vi "Waveform 64-128 channels LP pt by pt.vi"(4 "Enum":T1(ring), 6 "order":i32=2, 8 "fl":dbl, 10 "fs":dbl, 11 "Array in":waveform(dbl)[](array[waveform])) -> (3 "Array out":waveform(dbl)[](array[waveform]))   [LabVIEW 2016, in "LockinDAQ.lvclass"]
uses:
  LockinDAQ.lvclass
  <vilib>/Analysis/3filter.llb/Filter Passband Type.ctl
  <vilib>/Analysis/baseanly.llb/Mean (DBL).vi
  <vilib>/addons/Digital Filter Design/Process.llb/DFD Filtering (Wfm NChan).vi
  <vilib>/addons/System Identification/Data Preprocess.llb/SI Lowpass Filter (SISO Waveform).vi
  <vilib>/Analysis/3filter.llb/Butterworth Filter (DBL).vi
  <vilib>/ptbypt/NI_PtbyPt.lvlib
  <vilib>/Analysis/NI_AALBase.lvlib
  <vilib>/addons/System Identification/NI_SysID.lvlib
  <vilib>/addons/Digital Filter Design/NI_DigFilterLicensed.lvlib
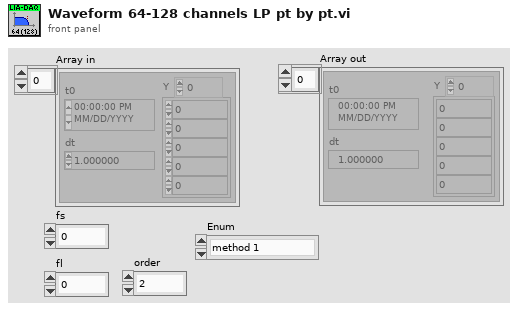
[diagram p1: front panel]
types:
  T1 = enum16{"method 1", "method 2", "method 3", "method 4", "method 5"}
  T2 = typedef "NI_AALBase.lvlib/Filter Passband Type.ctl" = enum32{"Lowpass", "Highpass", "Bandpass", "Bandstop"}
  T3 = enum16{"Lowpass", "Highpass", "Bandpass", "Bandstop"}
  T4 = typedef "NI_DigFilterLicensed.lvlib/DFD Filter Obj.ctl" = cluster{"mSRate_Fs":dbl, "mSRate_Version":string, "mSRate_Comments":string, "mSRate_OrgCoef":T5, "mSRate_CurCoef":T5, "mSRate_Quantized?":bool, "mSRate_QCoef":T5, "mSRate_QSettings":T7[], "mSRate_Order":i32, "mSRate_Scaling":cluster{"mSRate_ScaleByPowerOf2?":bool, "mSRate_ScaleType":T9}}
  T5 = typedef "NI_DigFilterLicensed.lvlib/DFD Filter Coef.ctl" = cluster{"type":T6, "gain":dbl, "coef a (k)":dbl[], "coef b (v)":dbl[]}
  T6 = typedef "NI_DigFilterLicensed.lvlib/DFD Filter Structure Type Selector.ctl" = enum16{"Undefined", "FIR Direct Form", "FIR Direct Form Transposed", "FIR Symmetric", "FIR Antisymmetric", "IIR Direct Form I", "IIR Direct Form I Transposed", "IIR Direct Form II", "IIR Direct Form II Transposed", "IIR Cascaded Second Order Sections Form I", "IIR Cascaded Second Order Sections Form I Transposed", "IIR Cascaded Second Order Sections Form II", "IIR Cascaded Second Order Sections Form II Transposed", "Lattice Allpass (basic sections)", "Lattice Allpass (one multiplier sections)", "Lattice Allpass (normalized sections)", "Lattice AR (basic sections)", "Lattice AR (one multiplier sections)", "Lattice AR (normalized sections)", "Lattice MA (minimum phase)", "Lattice MA (maximum phase)", "Lattice ARMA (basic sections)", "Lattice ARMA (one multiplier sections)", "Lattice ARMA (normalized sections)"}
  T7 = typedef "NI_DigFilterLicensed.lvlib/dfd_Internal Quantization Settings.ctl" = cluster{"source":T8, "wl":i16, "iwl":i16, "overflow mode":enum16{"Saturation", "Wrap"}, "rounding mode":enum16{"Nearest", "Truncation"}, "signed?":bool}
  T8 = typedef "NI_DigFilterLicensed.lvlib/dfd_Internal Quantization Srcs.ctl" = u16
  T9 = typedef "NI_DigFilterLicensed.lvlib/DFD Coef Norm Type.ctl" = enum16{"No Norm", "Time Domain 1-Norm", "Time Domain 2-Norm", "Time Domain Inf-Norm"}
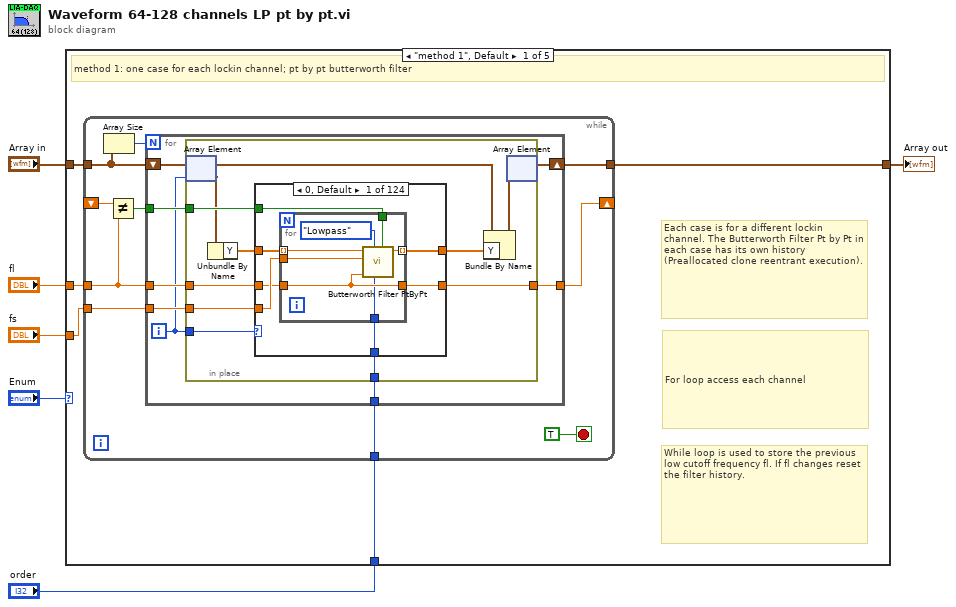
[diagram p0: block diagram]
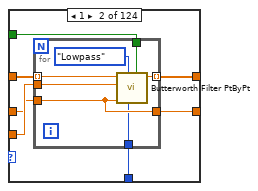
[diagram p2: hidden frame]
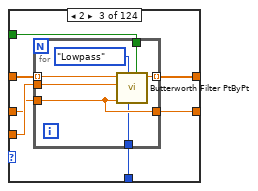
[diagram p3: hidden frame]
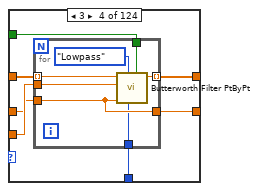
[diagram p4: hidden frame]
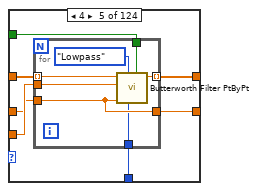
[diagram p5: hidden frame]
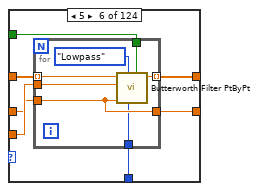
[diagram p6: hidden frame]
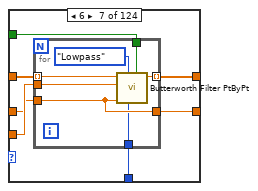
[diagram p7: hidden frame]
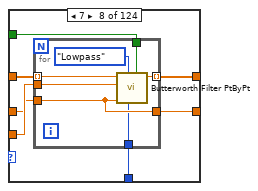
[diagram p8: hidden frame]
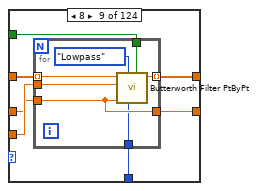
[diagram p9: hidden frame]
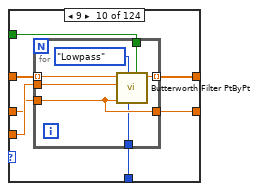
[diagram p10: hidden frame]
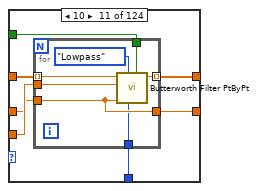
[diagram p11: hidden frame]
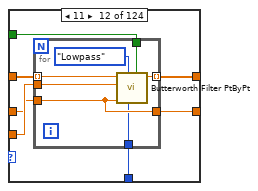
[diagram p12: hidden frame]
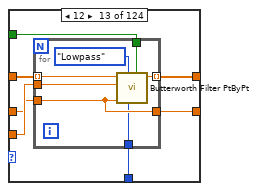
[diagram p13: hidden frame]
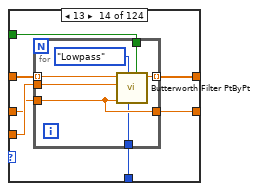
[diagram p14: hidden frame]
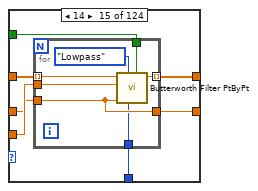
[diagram p15: hidden frame]
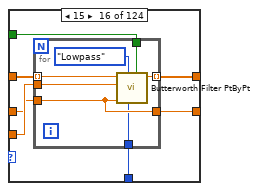
[diagram p16: hidden frame]
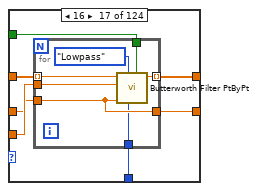
[diagram p17: hidden frame]
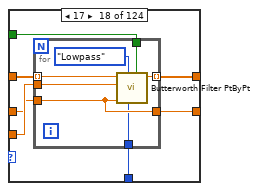
[diagram p18: hidden frame]
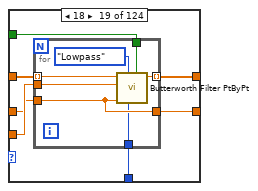
[diagram p19: hidden frame]
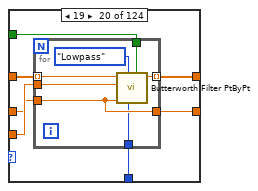
[diagram p20: hidden frame]
diagram:
  n1 = case shown="\"method 1\", Default" "Enum" {
    tunnel: "Array in" -> [w11 w1780 w3493 w3511 w3532]
    tunnel: [w10 w1779 w3492 w3510 w3531] -> w4
    tunnel: "fs" -> [w9 w1778 w3491 w3509 w3530]
    tunnel: "fl" -> [w8 w1777 w3490 w3508 w3529]
    tunnel: "order" -> [w7 w1776 w3489 w3507 w3528]
    frame "method 1", Default {
      # "For loop access each channel"
      # "While loop is used to store the previous low cutoff frequency fl. If fl changes reset the filter history."
      # "Each case is for a different lockin channel. The Butterworth Filter Pt by Pt in each case has its own history (Preallocated clone reentrant execution)."
      # "method 1: one case for each lockin channel; pt by pt butterworth filter"
      n2 = while {
        tunnel: w11 -> [w12]
        tunnel: [w21] -> w10
        tunnel: w9 -> [w18]
        tunnel: w8 -> [w15]
        shift-right: [w19] -> _
        shift-left: _ -> [w17]
        tunnel: w7 -> [w16]
        stop <- TRUE stop-if-true
        n3 = Array Size(array=w12) -> (size(s)=w13:i32)
        n4 = Not Equal?(x=w17, y=w15) -> (x != y?=w14:bool)
        n5 = for {
          N: w13 -> [_]
          tunnel: w18 -> [w29]
          tunnel: w15 -> [w28]
          tunnel: [w27] -> w19
          tunnel: w14 -> [w26]
          tunnel: w16 -> [w25]
          shift-right: [w22] -> w21
          shift-left: w12 -> [w24]
          i -> [w23]
          n6 = in-place {
            in-place-border: w29 -> [w39]
            in-place-border: w28 -> [w38]
            in-place-border: [w37] -> w27
            in-place-border: w26 -> [w36]
            in-place-border: w25 -> [w35]
            in-place-border: w23 -> [w32]
            n7 = in-place-array #1(w24, w23) -> (w31:waveform(dbl))
            n8 = Unbundle By Name(w31) -> ("Y"=w33:dbl[])
            n9 = case shown="0, Default" w32 {
              tunnel: w39 -> [w46 w60 w74 w88 w102 w116 w130 w144 w158 w172 w186 w200 w214 w228 w242 w256 w270 w284 w298 w312 w326 w340 w354 w368 w382 w396 w410 w424 w438 w452 w466 w480 w494 w508 w522 w536 w550 w564 w578 w592 w606 w620 w634 w648 w662 w676 w690 w704 w718 w732 w746 w760 w774 w788 w802 w816 w830 w844 w858 w872 w886 w900 w914 w928 w942 w956 w970 w984 w998 w1012 w1026 w1040 w1054 w1068 w1082 w1096 w1110 w1124 w1138 w1152 w1166 w1180 w1194 w1208 w1222 w1236 w1250 w1264 w1278 w1292 w1306 w1320 w1334 w1348 w1362 w1376 w1390 w1404 w1418 w1432 w1446 w1460 w1474 w1488 w1502 w1516 w1530 w1544 w1558 w1572 w1586 w1600 w1614 w1628 w1642 w1656 w1670 w1684 w1698 w1712 w1726 w1740 w1754 w1768]
              tunnel: w38 -> [w45 w59 w73 w87 w101 w115 w129 w143 w157 w171 w185 w199 w213 w227 w241 w255 w269 w283 w297 w311 w325 w339 w353 w367 w381 w395 w409 w423 w437 w451 w465 w479 w493 w507 w521 w535 w549 w563 w577 w591 w605 w619 w633 w647 w661 w675 w689 w703 w717 w731 w745 w759 w773 w787 w801 w815 w829 w843 w857 w871 w885 w899 w913 w927 w941 w955 w969 w983 w997 w1011 w1025 w1039 w1053 w1067 w1081 w1095 w1109 w1123 w1137 w1151 w1165 w1179 w1193 w1207 w1221 w1235 w1249 w1263 w1277 w1291 w1305 w1319 w1333 w1347 w1361 w1375 w1389 w1403 w1417 w1431 w1445 w1459 w1473 w1487 w1501 w1515 w1529 w1543 w1557 w1571 w1585 w1599 w1613 w1627 w1641 w1655 w1669 w1683 w1697 w1711 w1725 w1739 w1753 w1767]
              tunnel: [w44 w58 w72 w86 w100 w114 w128 w142 w156 w170 w184 w198 w212 w226 w240 w254 w268 w282 w296 w310 w324 w338 w352 w366 w380 w394 w408 w422 w436 w450 w464 w478 w492 w506 w520 w534 w548 w562 w576 w590 w604 w618 w632 w646 w660 w674 w688 w702 w716 w730 w744 w758 w772 w786 w800 w814 w828 w842 w856 w870 w884 w898 w912 w926 w940 w954 w968 w982 w996 w1010 w1024 w1038 w1052 w1066 w1080 w1094 w1108 w1122 w1136 w1150 w1164 w1178 w1192 w1206 w1220 w1234 w1248 w1262 w1276 w1290 w1304 w1318 w1332 w1346 w1360 w1374 w1388 w1402 w1416 w1430 w1444 w1458 w1472 w1486 w1500 w1514 w1528 w1542 w1556 w1570 w1584 w1598 w1612 w1626 w1640 w1654 w1668 w1682 w1696 w1710 w1724 w1738 w1752 w1766] -> w37
              tunnel: w36 -> [w43 w57 w71 w85 w99 w113 w127 w141 w155 w169 w183 w197 w211 w225 w239 w253 w267 w281 w295 w309 w323 w337 w351 w365 w379 w393 w407 w421 w435 w449 w463 w477 w491 w505 w519 w533 w547 w561 w575 w589 w603 w617 w631 w645 w659 w673 w687 w701 w715 w729 w743 w757 w771 w785 w799 w813 w827 w841 w855 w869 w883 w897 w911 w925 w939 w953 w967 w981 w995 w1009 w1023 w1037 w1051 w1065 w1079 w1093 w1107 w1121 w1135 w1149 w1163 w1177 w1191 w1205 w1219 w1233 w1247 w1261 w1275 w1289 w1303 w1317 w1331 w1345 w1359 w1373 w1387 w1401 w1415 w1429 w1443 w1457 w1471 w1485 w1499 w1513 w1527 w1541 w1555 w1569 w1583 w1597 w1611 w1625 w1639 w1653 w1667 w1681 w1695 w1709 w1723 w1737 w1751 w1765]
              tunnel: w35 -> [w42 w56 w70 w84 w98 w112 w126 w140 w154 w168 w182 w196 w210 w224 w238 w252 w266 w280 w294 w308 w322 w336 w350 w364 w378 w392 w406 w420 w434 w448 w462 w476 w490 w504 w518 w532 w546 w560 w574 w588 w602 w616 w630 w644 w658 w672 w686 w700 w714 w728 w742 w756 w770 w784 w798 w812 w826 w840 w854 w868 w882 w896 w910 w924 w938 w952 w966 w980 w994 w1008 w1022 w1036 w1050 w1064 w1078 w1092 w1106 w1120 w1134 w1148 w1162 w1176 w1190 w1204 w1218 w1232 w1246 w1260 w1274 w1288 w1302 w1316 w1330 w1344 w1358 w1372 w1386 w1400 w1414 w1428 w1442 w1456 w1470 w1484 w1498 w1512 w1526 w1540 w1554 w1568 w1582 w1596 w1610 w1624 w1638 w1652 w1666 w1680 w1694 w1708 w1722 w1736 w1750 w1764]
              tunnel: [w41 w55 w69 w83 w97 w111 w125 w139 w153 w167 w181 w195 w209 w223 w237 w251 w265 w279 w293 w307 w321 w335 w349 w363 w377 w391 w405 w419 w433 w447 w461 w475 w489 w503 w517 w531 w545 w559 w573 w587 w601 w615 w629 w643 w657 w671 w685 w699 w713 w727 w741 w755 w769 w783 w797 w811 w825 w839 w853 w867 w881 w895 w909 w923 w937 w951 w965 w979 w993 w1007 w1021 w1035 w1049 w1063 w1077 w1091 w1105 w1119 w1133 w1147 w1161 w1175 w1189 w1203 w1217 w1231 w1245 w1259 w1273 w1287 w1301 w1315 w1329 w1343 w1357 w1371 w1385 w1399 w1413 w1427 w1441 w1455 w1469 w1483 w1497 w1511 w1525 w1539 w1553 w1567 w1581 w1595 w1609 w1623 w1637 w1651 w1665 w1679 w1693 w1707 w1721 w1735 w1749 w1763] -> w34
              tunnel: w33 -> [w40 w54 w68 w82 w96 w110 w124 w138 w152 w166 w180 w194 w208 w222 w236 w250 w264 w278 w292 w306 w320 w334 w348 w362 w376 w390 w404 w418 w432 w446 w460 w474 w488 w502 w516 w530 w544 w558 w572 w586 w600 w614 w628 w642 w656 w670 w684 w698 w712 w726 w740 w754 w768 w782 w796 w810 w824 w838 w852 w866 w880 w894 w908 w922 w936 w950 w964 w978 w992 w1006 w1020 w1034 w1048 w1062 w1076 w1090 w1104 w1118 w1132 w1146 w1160 w1174 w1188 w1202 w1216 w1230 w1244 w1258 w1272 w1286 w1300 w1314 w1328 w1342 w1356 w1370 w1384 w1398 w1412 w1426 w1440 w1454 w1468 w1482 w1496 w1510 w1524 w1538 w1552 w1566 w1580 w1594 w1608 w1622 w1636 w1650 w1664 w1678 w1692 w1706 w1720 w1734 w1748 w1762]
              frame 0, Default {
                n10 = for {
                  tunnel: w40 -> [w53] mode=indexing
                  tunnel: w45 -> [w50]
                  tunnel: w46 -> [w52]
                  tunnel: [w51] -> w41 mode=indexing
                  tunnel: [w50] -> w44
                  tunnel: w43 -> [w48]
                  tunnel: w42 -> [w47]
                  n11 = call <vilib>:"Butterworth Filter PtByPt.vi"("initialize"=w48, "order"=w47, "filter type"=Filter_Passband_Type."Lowpass", "low cutoff freq: fl"=w50, "sampling freq: fs"=w52, "x"=w53) -> ("Filtered x"=w51:dbl)  [unwired: 3 in, 1 out]
                }
              }
              frame 1 {
                n12 = for {
                  tunnel: w54 -> [w67] mode=indexing
                  tunnel: w59 -> [w64]
                  tunnel: w60 -> [w66]
                  tunnel: [w65] -> w55 mode=indexing
                  tunnel: [w64] -> w58
                  tunnel: w57 -> [w62]
                  tunnel: w56 -> [w61]
                  n13 = call <vilib>:"Butterworth Filter PtByPt.vi"("initialize"=w62, "order"=w61, "filter type"=Filter_Passband_Type."Lowpass", "low cutoff freq: fl"=w64, "sampling freq: fs"=w66, "x"=w67) -> ("Filtered x"=w65:dbl)  [unwired: 3 in, 1 out]
                }
              }
              frame 2 {
                n14 = for {
                  tunnel: w68 -> [w81] mode=indexing
                  tunnel: w73 -> [w78]
                  tunnel: w74 -> [w80]
                  tunnel: [w79] -> w69 mode=indexing
                  tunnel: [w78] -> w72
                  tunnel: w71 -> [w76]
                  tunnel: w70 -> [w75]
                  n15 = call <vilib>:"Butterworth Filter PtByPt.vi"("initialize"=w76, "order"=w75, "filter type"=Filter_Passband_Type."Lowpass", "low cutoff freq: fl"=w78, "sampling freq: fs"=w80, "x"=w81) -> ("Filtered x"=w79:dbl)  [unwired: 3 in, 1 out]
                }
              }
              frame 3 {
                n16 = for {
                  tunnel: w82 -> [w95] mode=indexing
                  tunnel: w87 -> [w92]
                  tunnel: w88 -> [w94]
                  tunnel: [w93] -> w83 mode=indexing
                  tunnel: [w92] -> w86
                  tunnel: w85 -> [w90]
                  tunnel: w84 -> [w89]
                  n17 = call <vilib>:"Butterworth Filter PtByPt.vi"("initialize"=w90, "order"=w89, "filter type"=Filter_Passband_Type."Lowpass", "low cutoff freq: fl"=w92, "sampling freq: fs"=w94, "x"=w95) -> ("Filtered x"=w93:dbl)  [unwired: 3 in, 1 out]
                }
              }
              frame 4 {
                n18 = for {
                  tunnel: w96 -> [w109] mode=indexing
                  tunnel: w101 -> [w106]
                  tunnel: w102 -> [w108]
                  tunnel: [w107] -> w97 mode=indexing
                  tunnel: [w106] -> w100
                  tunnel: w99 -> [w104]
                  tunnel: w98 -> [w103]
                  n19 = call <vilib>:"Butterworth Filter PtByPt.vi"("initialize"=w104, "order"=w103, "filter type"=Filter_Passband_Type."Lowpass", "low cutoff freq: fl"=w106, "sampling freq: fs"=w108, "x"=w109) -> ("Filtered x"=w107:dbl)  [unwired: 3 in, 1 out]
                }
              }
              frame 5 {
                n20 = for {
                  tunnel: w110 -> [w123] mode=indexing
                  tunnel: w115 -> [w120]
                  tunnel: w116 -> [w122]
                  tunnel: [w121] -> w111 mode=indexing
                  tunnel: [w120] -> w114
                  tunnel: w113 -> [w118]
                  tunnel: w112 -> [w117]
                  n21 = call <vilib>:"Butterworth Filter PtByPt.vi"("initialize"=w118, "order"=w117, "filter type"=Filter_Passband_Type."Lowpass", "low cutoff freq: fl"=w120, "sampling freq: fs"=w122, "x"=w123) -> ("Filtered x"=w121:dbl)  [unwired: 3 in, 1 out]
                }
              }
              frame 6 {
                n22 = for {
                  tunnel: w124 -> [w137] mode=indexing
                  tunnel: w129 -> [w134]
                  tunnel: w130 -> [w136]
                  tunnel: [w135] -> w125 mode=indexing
                  tunnel: [w134] -> w128
                  tunnel: w127 -> [w132]
                  tunnel: w126 -> [w131]
                  n23 = call <vilib>:"Butterworth Filter PtByPt.vi"("initialize"=w132, "order"=w131, "filter type"=Filter_Passband_Type."Lowpass", "low cutoff freq: fl"=w134, "sampling freq: fs"=w136, "x"=w137) -> ("Filtered x"=w135:dbl)  [unwired: 3 in, 1 out]
                }
              }
              frame 7 {
                n24 = for {
                  tunnel: w138 -> [w151] mode=indexing
                  tunnel: w143 -> [w148]
                  tunnel: w144 -> [w150]
                  tunnel: [w149] -> w139 mode=indexing
                  tunnel: [w148] -> w142
                  tunnel: w141 -> [w146]
                  tunnel: w140 -> [w145]
                  n25 = call <vilib>:"Butterworth Filter PtByPt.vi"("initialize"=w146, "order"=w145, "filter type"=Filter_Passband_Type."Lowpass", "low cutoff freq: fl"=w148, "sampling freq: fs"=w150, "x"=w151) -> ("Filtered x"=w149:dbl)  [unwired: 3 in, 1 out]
                }
              }
              frame 8 {
                n26 = for {
                  tunnel: w152 -> [w165] mode=indexing
                  tunnel: w157 -> [w162]
                  tunnel: w158 -> [w164]
                  tunnel: [w163] -> w153 mode=indexing
                  tunnel: [w162] -> w156
                  tunnel: w155 -> [w160]
                  tunnel: w154 -> [w159]
                  n27 = call <vilib>:"Butterworth Filter PtByPt.vi"("initialize"=w160, "order"=w159, "filter type"=Filter_Passband_Type."Lowpass", "low cutoff freq: fl"=w162, "sampling freq: fs"=w164, "x"=w165) -> ("Filtered x"=w163:dbl)  [unwired: 3 in, 1 out]
                }
              }
              frame 9 {
                n28 = for {
                  tunnel: w166 -> [w179] mode=indexing
                  tunnel: w171 -> [w176]
                  tunnel: w172 -> [w178]
                  tunnel: [w177] -> w167 mode=indexing
                  tunnel: [w176] -> w170
                  tunnel: w169 -> [w174]
                  tunnel: w168 -> [w173]
                  n29 = call <vilib>:"Butterworth Filter PtByPt.vi"("initialize"=w174, "order"=w173, "filter type"=Filter_Passband_Type."Lowpass", "low cutoff freq: fl"=w176, "sampling freq: fs"=w178, "x"=w179) -> ("Filtered x"=w177:dbl)  [unwired: 3 in, 1 out]
                }
              }
              frame 10 {
                n30 = for {
                  tunnel: w180 -> [w193] mode=indexing
                  tunnel: w185 -> [w190]
                  tunnel: w186 -> [w192]
                  tunnel: [w191] -> w181 mode=indexing
                  tunnel: [w190] -> w184
                  tunnel: w183 -> [w188]
                  tunnel: w182 -> [w187]
                  n31 = call <vilib>:"Butterworth Filter PtByPt.vi"("initialize"=w188, "order"=w187, "filter type"=Filter_Passband_Type."Lowpass", "low cutoff freq: fl"=w190, "sampling freq: fs"=w192, "x"=w193) -> ("Filtered x"=w191:dbl)  [unwired: 3 in, 1 out]
                }
              }
              frame 11 {
                n32 = for {
                  tunnel: w194 -> [w207] mode=indexing
                  tunnel: w199 -> [w204]
                  tunnel: w200 -> [w206]
                  tunnel: [w205] -> w195 mode=indexing
                  tunnel: [w204] -> w198
                  tunnel: w197 -> [w202]
                  tunnel: w196 -> [w201]
                  n33 = call <vilib>:"Butterworth Filter PtByPt.vi"("initialize"=w202, "order"=w201, "filter type"=Filter_Passband_Type."Lowpass", "low cutoff freq: fl"=w204, "sampling freq: fs"=w206, "x"=w207) -> ("Filtered x"=w205:dbl)  [unwired: 3 in, 1 out]
                }
              }
              frame 12 {
                n34 = for {
                  tunnel: w208 -> [w221] mode=indexing
                  tunnel: w213 -> [w218]
                  tunnel: w214 -> [w220]
                  tunnel: [w219] -> w209 mode=indexing
                  tunnel: [w218] -> w212
                  tunnel: w211 -> [w216]
                  tunnel: w210 -> [w215]
                  n35 = call <vilib>:"Butterworth Filter PtByPt.vi"("initialize"=w216, "order"=w215, "filter type"=Filter_Passband_Type."Lowpass", "low cutoff freq: fl"=w218, "sampling freq: fs"=w220, "x"=w221) -> ("Filtered x"=w219:dbl)  [unwired: 3 in, 1 out]
                }
              }
              frame 13 {
                n36 = for {
                  tunnel: w222 -> [w235] mode=indexing
                  tunnel: w227 -> [w232]
                  tunnel: w228 -> [w234]
                  tunnel: [w233] -> w223 mode=indexing
                  tunnel: [w232] -> w226
                  tunnel: w225 -> [w230]
                  tunnel: w224 -> [w229]
                  n37 = call <vilib>:"Butterworth Filter PtByPt.vi"("initialize"=w230, "order"=w229, "filter type"=Filter_Passband_Type."Lowpass", "low cutoff freq: fl"=w232, "sampling freq: fs"=w234, "x"=w235) -> ("Filtered x"=w233:dbl)  [unwired: 3 in, 1 out]
                }
              }
              frame 14 {
                n38 = for {
                  tunnel: w236 -> [w249] mode=indexing
                  tunnel: w241 -> [w246]
                  tunnel: w242 -> [w248]
                  tunnel: [w247] -> w237 mode=indexing
                  tunnel: [w246] -> w240
                  tunnel: w239 -> [w244]
                  tunnel: w238 -> [w243]
                  n39 = call <vilib>:"Butterworth Filter PtByPt.vi"("initialize"=w244, "order"=w243, "filter type"=Filter_Passband_Type."Lowpass", "low cutoff freq: fl"=w246, "sampling freq: fs"=w248, "x"=w249) -> ("Filtered x"=w247:dbl)  [unwired: 3 in, 1 out]
                }
              }
              frame 15 {
                n40 = for {
                  tunnel: w250 -> [w263] mode=indexing
                  tunnel: w255 -> [w260]
                  tunnel: w256 -> [w262]
                  tunnel: [w261] -> w251 mode=indexing
                  tunnel: [w260] -> w254
                  tunnel: w253 -> [w258]
                  tunnel: w252 -> [w257]
                  n41 = call <vilib>:"Butterworth Filter PtByPt.vi"("initialize"=w258, "order"=w257, "filter type"=Filter_Passband_Type."Lowpass", "low cutoff freq: fl"=w260, "sampling freq: fs"=w262, "x"=w263) -> ("Filtered x"=w261:dbl)  [unwired: 3 in, 1 out]
                }
              }
              frame 16 {
                n42 = for {
                  tunnel: w264 -> [w277] mode=indexing
                  tunnel: w269 -> [w274]
                  tunnel: w270 -> [w276]
                  tunnel: [w275] -> w265 mode=indexing
                  tunnel: [w274] -> w268
                  tunnel: w267 -> [w272]
                  tunnel: w266 -> [w271]
                  n43 = call <vilib>:"Butterworth Filter PtByPt.vi"("initialize"=w272, "order"=w271, "filter type"=Filter_Passband_Type."Lowpass", "low cutoff freq: fl"=w274, "sampling freq: fs"=w276, "x"=w277) -> ("Filtered x"=w275:dbl)  [unwired: 3 in, 1 out]
                }
              }
              frame 17 {
                n44 = for {
                  tunnel: w278 -> [w291] mode=indexing
                  tunnel: w283 -> [w288]
                  tunnel: w284 -> [w290]
                  tunnel: [w289] -> w279 mode=indexing
                  tunnel: [w288] -> w282
                  tunnel: w281 -> [w286]
                  tunnel: w280 -> [w285]
                  n45 = call <vilib>:"Butterworth Filter PtByPt.vi"("initialize"=w286, "order"=w285, "filter type"=Filter_Passband_Type."Lowpass", "low cutoff freq: fl"=w288, "sampling freq: fs"=w290, "x"=w291) -> ("Filtered x"=w289:dbl)  [unwired: 3 in, 1 out]
                }
              }
              frame 18 {
                n46 = for {
                  tunnel: w292 -> [w305] mode=indexing
                  tunnel: w297 -> [w302]
                  tunnel: w298 -> [w304]
                  tunnel: [w303] -> w293 mode=indexing
                  tunnel: [w302] -> w296
                  tunnel: w295 -> [w300]
                  tunnel: w294 -> [w299]
                  n47 = call <vilib>:"Butterworth Filter PtByPt.vi"("initialize"=w300, "order"=w299, "filter type"=Filter_Passband_Type."Lowpass", "low cutoff freq: fl"=w302, "sampling freq: fs"=w304, "x"=w305) -> ("Filtered x"=w303:dbl)  [unwired: 3 in, 1 out]
                }
              }
              frame 19 {
                n48 = for {
                  tunnel: w306 -> [w319] mode=indexing
                  tunnel: w311 -> [w316]
                  tunnel: w312 -> [w318]
                  tunnel: [w317] -> w307 mode=indexing
                  tunnel: [w316] -> w310
                  tunnel: w309 -> [w314]
                  tunnel: w308 -> [w313]
                  n49 = call <vilib>:"Butterworth Filter PtByPt.vi"("initialize"=w314, "order"=w313, "filter type"=Filter_Passband_Type."Lowpass", "low cutoff freq: fl"=w316, "sampling freq: fs"=w318, "x"=w319) -> ("Filtered x"=w317:dbl)  [unwired: 3 in, 1 out]
                }
              }
              frame 20 {
                n50 = for {
                  tunnel: w320 -> [w333] mode=indexing
                  tunnel: w325 -> [w330]
                  tunnel: w326 -> [w332]
                  tunnel: [w331] -> w321 mode=indexing
                  tunnel: [w330] -> w324
                  tunnel: w323 -> [w328]
                  tunnel: w322 -> [w327]
                  n51 = call <vilib>:"Butterworth Filter PtByPt.vi"("initialize"=w328, "order"=w327, "filter type"=Filter_Passband_Type."Lowpass", "low cutoff freq: fl"=w330, "sampling freq: fs"=w332, "x"=w333) -> ("Filtered x"=w331:dbl)  [unwired: 3 in, 1 out]
                }
              }
              frame 21 {
                n52 = for {
                  tunnel: w334 -> [w347] mode=indexing
                  tunnel: w339 -> [w344]
                  tunnel: w340 -> [w346]
                  tunnel: [w345] -> w335 mode=indexing
                  tunnel: [w344] -> w338
                  tunnel: w337 -> [w342]
                  tunnel: w336 -> [w341]
                  n53 = call <vilib>:"Butterworth Filter PtByPt.vi"("initialize"=w342, "order"=w341, "filter type"=Filter_Passband_Type."Lowpass", "low cutoff freq: fl"=w344, "sampling freq: fs"=w346, "x"=w347) -> ("Filtered x"=w345:dbl)  [unwired: 3 in, 1 out]
                }
              }
              frame 22 {
                n54 = for {
                  tunnel: w348 -> [w361] mode=indexing
                  tunnel: w353 -> [w358]
                  tunnel: w354 -> [w360]
                  tunnel: [w359] -> w349 mode=indexing
                  tunnel: [w358] -> w352
                  tunnel: w351 -> [w356]
                  tunnel: w350 -> [w355]
                  n55 = call <vilib>:"Butterworth Filter PtByPt.vi"("initialize"=w356, "order"=w355, "filter type"=Filter_Passband_Type."Lowpass", "low cutoff freq: fl"=w358, "sampling freq: fs"=w360, "x"=w361) -> ("Filtered x"=w359:dbl)  [unwired: 3 in, 1 out]
                }
              }
              frame 23 {
                n56 = for {
                  tunnel: w362 -> [w375] mode=indexing
                  tunnel: w367 -> [w372]
                  tunnel: w368 -> [w374]
                  tunnel: [w373] -> w363 mode=indexing
                  tunnel: [w372] -> w366
                  tunnel: w365 -> [w370]
                  tunnel: w364 -> [w369]
                  n57 = call <vilib>:"Butterworth Filter PtByPt.vi"("initialize"=w370, "order"=w369, "filter type"=Filter_Passband_Type."Lowpass", "low cutoff freq: fl"=w372, "sampling freq: fs"=w374, "x"=w375) -> ("Filtered x"=w373:dbl)  [unwired: 3 in, 1 out]
                }
              }
              frame 24 {
                n58 = for {
                  tunnel: w376 -> [w389] mode=indexing
                  tunnel: w381 -> [w386]
                  tunnel: w382 -> [w388]
                  tunnel: [w387] -> w377 mode=indexing
                  tunnel: [w386] -> w380
                  tunnel: w379 -> [w384]
                  tunnel: w378 -> [w383]
                  n59 = call <vilib>:"Butterworth Filter PtByPt.vi"("initialize"=w384, "order"=w383, "filter type"=Filter_Passband_Type."Lowpass", "low cutoff freq: fl"=w386, "sampling freq: fs"=w388, "x"=w389) -> ("Filtered x"=w387:dbl)  [unwired: 3 in, 1 out]
                }
              }
              frame 25 {
                n60 = for {
                  tunnel: w390 -> [w403] mode=indexing
                  tunnel: w395 -> [w400]
                  tunnel: w396 -> [w402]
                  tunnel: [w401] -> w391 mode=indexing
                  tunnel: [w400] -> w394
                  tunnel: w393 -> [w398]
                  tunnel: w392 -> [w397]
                  n61 = call <vilib>:"Butterworth Filter PtByPt.vi"("initialize"=w398, "order"=w397, "filter type"=Filter_Passband_Type."Lowpass", "low cutoff freq: fl"=w400, "sampling freq: fs"=w402, "x"=w403) -> ("Filtered x"=w401:dbl)  [unwired: 3 in, 1 out]
                }
              }
              frame 26 {
                n62 = for {
                  tunnel: w404 -> [w417] mode=indexing
                  tunnel: w409 -> [w414]
                  tunnel: w410 -> [w416]
                  tunnel: [w415] -> w405 mode=indexing
                  tunnel: [w414] -> w408
                  tunnel: w407 -> [w412]
                  tunnel: w406 -> [w411]
                  n63 = call <vilib>:"Butterworth Filter PtByPt.vi"("initialize"=w412, "order"=w411, "filter type"=Filter_Passband_Type."Lowpass", "low cutoff freq: fl"=w414, "sampling freq: fs"=w416, "x"=w417) -> ("Filtered x"=w415:dbl)  [unwired: 3 in, 1 out]
                }
              }
              frame 27 {
                n64 = for {
                  tunnel: w418 -> [w431] mode=indexing
                  tunnel: w423 -> [w428]
                  tunnel: w424 -> [w430]
                  tunnel: [w429] -> w419 mode=indexing
                  tunnel: [w428] -> w422
                  tunnel: w421 -> [w426]
                  tunnel: w420 -> [w425]
                  n65 = call <vilib>:"Butterworth Filter PtByPt.vi"("initialize"=w426, "order"=w425, "filter type"=Filter_Passband_Type."Lowpass", "low cutoff freq: fl"=w428, "sampling freq: fs"=w430, "x"=w431) -> ("Filtered x"=w429:dbl)  [unwired: 3 in, 1 out]
                }
              }
              frame 28 {
                n66 = for {
                  tunnel: w432 -> [w445] mode=indexing
                  tunnel: w437 -> [w442]
                  tunnel: w438 -> [w444]
                  tunnel: [w443] -> w433 mode=indexing
                  tunnel: [w442] -> w436
                  tunnel: w435 -> [w440]
                  tunnel: w434 -> [w439]
                  n67 = call <vilib>:"Butterworth Filter PtByPt.vi"("initialize"=w440, "order"=w439, "filter type"=Filter_Passband_Type."Lowpass", "low cutoff freq: fl"=w442, "sampling freq: fs"=w444, "x"=w445) -> ("Filtered x"=w443:dbl)  [unwired: 3 in, 1 out]
                }
              }
              frame 29 {
                n68 = for {
                  tunnel: w446 -> [w459] mode=indexing
                  tunnel: w451 -> [w456]
                  tunnel: w452 -> [w458]
                  tunnel: [w457] -> w447 mode=indexing
                  tunnel: [w456] -> w450
                  tunnel: w449 -> [w454]
                  tunnel: w448 -> [w453]
                  n69 = call <vilib>:"Butterworth Filter PtByPt.vi"("initialize"=w454, "order"=w453, "filter type"=Filter_Passband_Type."Lowpass", "low cutoff freq: fl"=w456, "sampling freq: fs"=w458, "x"=w459) -> ("Filtered x"=w457:dbl)  [unwired: 3 in, 1 out]
                }
              }
              frame 30 {
                n70 = for {
                  tunnel: w460 -> [w473] mode=indexing
                  tunnel: w465 -> [w470]
                  tunnel: w466 -> [w472]
                  tunnel: [w471] -> w461 mode=indexing
                  tunnel: [w470] -> w464
                  tunnel: w463 -> [w468]
                  tunnel: w462 -> [w467]
                  n71 = call <vilib>:"Butterworth Filter PtByPt.vi"("initialize"=w468, "order"=w467, "filter type"=Filter_Passband_Type."Lowpass", "low cutoff freq: fl"=w470, "sampling freq: fs"=w472, "x"=w473) -> ("Filtered x"=w471:dbl)  [unwired: 3 in, 1 out]
                }
              }
              frame 31 {
                n72 = for {
                  tunnel: w474 -> [w487] mode=indexing
                  tunnel: w479 -> [w484]
                  tunnel: w480 -> [w486]
                  tunnel: [w485] -> w475 mode=indexing
                  tunnel: [w484] -> w478
                  tunnel: w477 -> [w482]
                  tunnel: w476 -> [w481]
                  n73 = call <vilib>:"Butterworth Filter PtByPt.vi"("initialize"=w482, "order"=w481, "filter type"=Filter_Passband_Type."Lowpass", "low cutoff freq: fl"=w484, "sampling freq: fs"=w486, "x"=w487) -> ("Filtered x"=w485:dbl)  [unwired: 3 in, 1 out]
                }
              }
              frame 32 {
                n74 = for {
                  tunnel: w488 -> [w501] mode=indexing
                  tunnel: w493 -> [w498]
                  tunnel: w494 -> [w500]
                  tunnel: [w499] -> w489 mode=indexing
                  tunnel: [w498] -> w492
                  tunnel: w491 -> [w496]
                  tunnel: w490 -> [w495]
                  n75 = call <vilib>:"Butterworth Filter PtByPt.vi"("initialize"=w496, "order"=w495, "filter type"=Filter_Passband_Type."Lowpass", "low cutoff freq: fl"=w498, "sampling freq: fs"=w500, "x"=w501) -> ("Filtered x"=w499:dbl)  [unwired: 3 in, 1 out]
                }
              }
              frame 33 {
                n76 = for {
                  tunnel: w502 -> [w515] mode=indexing
                  tunnel: w507 -> [w512]
                  tunnel: w508 -> [w514]
                  tunnel: [w513] -> w503 mode=indexing
                  tunnel: [w512] -> w506
                  tunnel: w505 -> [w510]
                  tunnel: w504 -> [w509]
                  n77 = call <vilib>:"Butterworth Filter PtByPt.vi"("initialize"=w510, "order"=w509, "filter type"=Filter_Passband_Type."Lowpass", "low cutoff freq: fl"=w512, "sampling freq: fs"=w514, "x"=w515) -> ("Filtered x"=w513:dbl)  [unwired: 3 in, 1 out]
                }
              }
              frame 34 {
                n78 = for {
                  tunnel: w516 -> [w529] mode=indexing
                  tunnel: w521 -> [w526]
                  tunnel: w522 -> [w528]
                  tunnel: [w527] -> w517 mode=indexing
                  tunnel: [w526] -> w520
                  tunnel: w519 -> [w524]
                  tunnel: w518 -> [w523]
                  n79 = call <vilib>:"Butterworth Filter PtByPt.vi"("initialize"=w524, "order"=w523, "filter type"=Filter_Passband_Type."Lowpass", "low cutoff freq: fl"=w526, "sampling freq: fs"=w528, "x"=w529) -> ("Filtered x"=w527:dbl)  [unwired: 3 in, 1 out]
                }
              }
              frame 35 {
                n80 = for {
                  tunnel: w530 -> [w543] mode=indexing
                  tunnel: w535 -> [w540]
                  tunnel: w536 -> [w542]
                  tunnel: [w541] -> w531 mode=indexing
                  tunnel: [w540] -> w534
                  tunnel: w533 -> [w538]
                  tunnel: w532 -> [w537]
                  n81 = call <vilib>:"Butterworth Filter PtByPt.vi"("initialize"=w538, "order"=w537, "filter type"=Filter_Passband_Type."Lowpass", "low cutoff freq: fl"=w540, "sampling freq: fs"=w542, "x"=w543) -> ("Filtered x"=w541:dbl)  [unwired: 3 in, 1 out]
                }
              }
              frame 36 {
                n82 = for {
                  tunnel: w544 -> [w557] mode=indexing
                  tunnel: w549 -> [w554]
                  tunnel: w550 -> [w556]
                  tunnel: [w555] -> w545 mode=indexing
                  tunnel: [w554] -> w548
                  tunnel: w547 -> [w552]
                  tunnel: w546 -> [w551]
                  n83 = call <vilib>:"Butterworth Filter PtByPt.vi"("initialize"=w552, "order"=w551, "filter type"=Filter_Passband_Type."Lowpass", "low cutoff freq: fl"=w554, "sampling freq: fs"=w556, "x"=w557) -> ("Filtered x"=w555:dbl)  [unwired: 3 in, 1 out]
                }
              }
              frame 37 {
                n84 = for {
                  tunnel: w558 -> [w571] mode=indexing
                  tunnel: w563 -> [w568]
                  tunnel: w564 -> [w570]
                  tunnel: [w569] -> w559 mode=indexing
                  tunnel: [w568] -> w562
                  tunnel: w561 -> [w566]
                  tunnel: w560 -> [w565]
                  n85 = call <vilib>:"Butterworth Filter PtByPt.vi"("initialize"=w566, "order"=w565, "filter type"=Filter_Passband_Type."Lowpass", "low cutoff freq: fl"=w568, "sampling freq: fs"=w570, "x"=w571) -> ("Filtered x"=w569:dbl)  [unwired: 3 in, 1 out]
                }
              }
              frame 38 {
                n86 = for {
                  tunnel: w572 -> [w585] mode=indexing
                  tunnel: w577 -> [w582]
                  tunnel: w578 -> [w584]
                  tunnel: [w583] -> w573 mode=indexing
                  tunnel: [w582] -> w576
                  tunnel: w575 -> [w580]
                  tunnel: w574 -> [w579]
                  n87 = call <vilib>:"Butterworth Filter PtByPt.vi"("initialize"=w580, "order"=w579, "filter type"=Filter_Passband_Type."Lowpass", "low cutoff freq: fl"=w582, "sampling freq: fs"=w584, "x"=w585) -> ("Filtered x"=w583:dbl)  [unwired: 3 in, 1 out]
                }
              }
              frame 39 {
                n88 = for {
                  tunnel: w586 -> [w599] mode=indexing
                  tunnel: w591 -> [w596]
                  tunnel: w592 -> [w598]
                  tunnel: [w597] -> w587 mode=indexing
                  tunnel: [w596] -> w590
                  tunnel: w589 -> [w594]
                  tunnel: w588 -> [w593]
                  n89 = call <vilib>:"Butterworth Filter PtByPt.vi"("initialize"=w594, "order"=w593, "filter type"=Filter_Passband_Type."Lowpass", "low cutoff freq: fl"=w596, "sampling freq: fs"=w598, "x"=w599) -> ("Filtered x"=w597:dbl)  [unwired: 3 in, 1 out]
                }
              }
              frame 40 {
                n90 = for {
                  tunnel: w600 -> [w613] mode=indexing
                  tunnel: w605 -> [w610]
                  tunnel: w606 -> [w612]
                  tunnel: [w611] -> w601 mode=indexing
                  tunnel: [w610] -> w604
                  tunnel: w603 -> [w608]
                  tunnel: w602 -> [w607]
                  n91 = call <vilib>:"Butterworth Filter PtByPt.vi"("initialize"=w608, "order"=w607, "filter type"=Filter_Passband_Type."Lowpass", "low cutoff freq: fl"=w610, "sampling freq: fs"=w612, "x"=w613) -> ("Filtered x"=w611:dbl)  [unwired: 3 in, 1 out]
                }
              }
              frame 41 {
                n92 = for {
                  tunnel: w614 -> [w627] mode=indexing
                  tunnel: w619 -> [w624]
                  tunnel: w620 -> [w626]
                  tunnel: [w625] -> w615 mode=indexing
                  tunnel: [w624] -> w618
                  tunnel: w617 -> [w622]
                  tunnel: w616 -> [w621]
                  n93 = call <vilib>:"Butterworth Filter PtByPt.vi"("initialize"=w622, "order"=w621, "filter type"=Filter_Passband_Type."Lowpass", "low cutoff freq: fl"=w624, "sampling freq: fs"=w626, "x"=w627) -> ("Filtered x"=w625:dbl)  [unwired: 3 in, 1 out]
                }
              }
              frame 42 {
                n94 = for {
                  tunnel: w628 -> [w641] mode=indexing
                  tunnel: w633 -> [w638]
                  tunnel: w634 -> [w640]
                  tunnel: [w639] -> w629 mode=indexing
                  tunnel: [w638] -> w632
                  tunnel: w631 -> [w636]
                  tunnel: w630 -> [w635]
                  n95 = call <vilib>:"Butterworth Filter PtByPt.vi"("initialize"=w636, "order"=w635, "filter type"=Filter_Passband_Type."Lowpass", "low cutoff freq: fl"=w638, "sampling freq: fs"=w640, "x"=w641) -> ("Filtered x"=w639:dbl)  [unwired: 3 in, 1 out]
                }
              }
              frame 43 {
                n96 = for {
                  tunnel: w642 -> [w655] mode=indexing
                  tunnel: w647 -> [w652]
                  tunnel: w648 -> [w654]
                  tunnel: [w653] -> w643 mode=indexing
                  tunnel: [w652] -> w646
                  tunnel: w645 -> [w650]
                  tunnel: w644 -> [w649]
                  n97 = call <vilib>:"Butterworth Filter PtByPt.vi"("initialize"=w650, "order"=w649, "filter type"=Filter_Passband_Type."Lowpass", "low cutoff freq: fl"=w652, "sampling freq: fs"=w654, "x"=w655) -> ("Filtered x"=w653:dbl)  [unwired: 3 in, 1 out]
                }
              }
              frame 44 {
                n98 = for {
                  tunnel: w656 -> [w669] mode=indexing
                  tunnel: w661 -> [w666]
                  tunnel: w662 -> [w668]
                  tunnel: [w667] -> w657 mode=indexing
                  tunnel: [w666] -> w660
                  tunnel: w659 -> [w664]
                  tunnel: w658 -> [w663]
                  n99 = call <vilib>:"Butterworth Filter PtByPt.vi"("initialize"=w664, "order"=w663, "filter type"=Filter_Passband_Type."Lowpass", "low cutoff freq: fl"=w666, "sampling freq: fs"=w668, "x"=w669) -> ("Filtered x"=w667:dbl)  [unwired: 3 in, 1 out]
                }
              }
              frame 45 {
                n100 = for {
                  tunnel: w670 -> [w683] mode=indexing
                  tunnel: w675 -> [w680]
                  tunnel: w676 -> [w682]
                  tunnel: [w681] -> w671 mode=indexing
                  tunnel: [w680] -> w674
                  tunnel: w673 -> [w678]
                  tunnel: w672 -> [w677]
                  n101 = call <vilib>:"Butterworth Filter PtByPt.vi"("initialize"=w678, "order"=w677, "filter type"=Filter_Passband_Type."Lowpass", "low cutoff freq: fl"=w680, "sampling freq: fs"=w682, "x"=w683) -> ("Filtered x"=w681:dbl)  [unwired: 3 in, 1 out]
                }
              }
              frame 46 {
                n102 = for {
                  tunnel: w684 -> [w697] mode=indexing
                  tunnel: w689 -> [w694]
                  tunnel: w690 -> [w696]
                  tunnel: [w695] -> w685 mode=indexing
                  tunnel: [w694] -> w688
                  tunnel: w687 -> [w692]
                  tunnel: w686 -> [w691]
                  n103 = call <vilib>:"Butterworth Filter PtByPt.vi"("initialize"=w692, "order"=w691, "filter type"=Filter_Passband_Type."Lowpass", "low cutoff freq: fl"=w694, "sampling freq: fs"=w696, "x"=w697) -> ("Filtered x"=w695:dbl)  [unwired: 3 in, 1 out]
                }
              }
              frame 47 {
                n104 = for {
                  tunnel: w698 -> [w711] mode=indexing
                  tunnel: w703 -> [w708]
                  tunnel: w704 -> [w710]
                  tunnel: [w709] -> w699 mode=indexing
                  tunnel: [w708] -> w702
                  tunnel: w701 -> [w706]
                  tunnel: w700 -> [w705]
                  n105 = call <vilib>:"Butterworth Filter PtByPt.vi"("initialize"=w706, "order"=w705, "filter type"=Filter_Passband_Type."Lowpass", "low cutoff freq: fl"=w708, "sampling freq: fs"=w710, "x"=w711) -> ("Filtered x"=w709:dbl)  [unwired: 3 in, 1 out]
                }
              }
              frame 48 {
                n106 = for {
                  tunnel: w712 -> [w725] mode=indexing
                  tunnel: w717 -> [w722]
                  tunnel: w718 -> [w724]
                  tunnel: [w723] -> w713 mode=indexing
                  tunnel: [w722] -> w716
                  tunnel: w715 -> [w720]
                  tunnel: w714 -> [w719]
                  n107 = call <vilib>:"Butterworth Filter PtByPt.vi"("initialize"=w720, "order"=w719, "filter type"=Filter_Passband_Type."Lowpass", "low cutoff freq: fl"=w722, "sampling freq: fs"=w724, "x"=w725) -> ("Filtered x"=w723:dbl)  [unwired: 3 in, 1 out]
                }
              }
              frame 49 {
                n108 = for {
                  tunnel: w726 -> [w739] mode=indexing
                  tunnel: w731 -> [w736]
                  tunnel: w732 -> [w738]
                  tunnel: [w737] -> w727 mode=indexing
                  tunnel: [w736] -> w730
                  tunnel: w729 -> [w734]
                  tunnel: w728 -> [w733]
                  n109 = call <vilib>:"Butterworth Filter PtByPt.vi"("initialize"=w734, "order"=w733, "filter type"=Filter_Passband_Type."Lowpass", "low cutoff freq: fl"=w736, "sampling freq: fs"=w738, "x"=w739) -> ("Filtered x"=w737:dbl)  [unwired: 3 in, 1 out]
                }
              }
              frame 50 {
                n110 = for {
                  tunnel: w740 -> [w753] mode=indexing
                  tunnel: w745 -> [w750]
                  tunnel: w746 -> [w752]
                  tunnel: [w751] -> w741 mode=indexing
                  tunnel: [w750] -> w744
                  tunnel: w743 -> [w748]
                  tunnel: w742 -> [w747]
                  n111 = call <vilib>:"Butterworth Filter PtByPt.vi"("initialize"=w748, "order"=w747, "filter type"=Filter_Passband_Type."Lowpass", "low cutoff freq: fl"=w750, "sampling freq: fs"=w752, "x"=w753) -> ("Filtered x"=w751:dbl)  [unwired: 3 in, 1 out]
                }
              }
              frame 51 {
                n112 = for {
                  tunnel: w754 -> [w767] mode=indexing
                  tunnel: w759 -> [w764]
                  tunnel: w760 -> [w766]
                  tunnel: [w765] -> w755 mode=indexing
                  tunnel: [w764] -> w758
                  tunnel: w757 -> [w762]
                  tunnel: w756 -> [w761]
                  n113 = call <vilib>:"Butterworth Filter PtByPt.vi"("initialize"=w762, "order"=w761, "filter type"=Filter_Passband_Type."Lowpass", "low cutoff freq: fl"=w764, "sampling freq: fs"=w766, "x"=w767) -> ("Filtered x"=w765:dbl)  [unwired: 3 in, 1 out]
                }
              }
              frame 52 {
                n114 = for {
                  tunnel: w768 -> [w781] mode=indexing
                  tunnel: w773 -> [w778]
                  tunnel: w774 -> [w780]
                  tunnel: [w779] -> w769 mode=indexing
                  tunnel: [w778] -> w772
                  tunnel: w771 -> [w776]
                  tunnel: w770 -> [w775]
                  n115 = call <vilib>:"Butterworth Filter PtByPt.vi"("initialize"=w776, "order"=w775, "filter type"=Filter_Passband_Type."Lowpass", "low cutoff freq: fl"=w778, "sampling freq: fs"=w780, "x"=w781) -> ("Filtered x"=w779:dbl)  [unwired: 3 in, 1 out]
                }
              }
              frame 53 {
                n116 = for {
                  tunnel: w782 -> [w795] mode=indexing
                  tunnel: w787 -> [w792]
                  tunnel: w788 -> [w794]
                  tunnel: [w793] -> w783 mode=indexing
                  tunnel: [w792] -> w786
                  tunnel: w785 -> [w790]
                  tunnel: w784 -> [w789]
                  n117 = call <vilib>:"Butterworth Filter PtByPt.vi"("initialize"=w790, "order"=w789, "filter type"=Filter_Passband_Type."Lowpass", "low cutoff freq: fl"=w792, "sampling freq: fs"=w794, "x"=w795) -> ("Filtered x"=w793:dbl)  [unwired: 3 in, 1 out]
                }
              }
              frame 54 {
                n118 = for {
                  tunnel: w796 -> [w809] mode=indexing
                  tunnel: w801 -> [w806]
                  tunnel: w802 -> [w808]
                  tunnel: [w807] -> w797 mode=indexing
                  tunnel: [w806] -> w800
                  tunnel: w799 -> [w804]
                  tunnel: w798 -> [w803]
                  n119 = call <vilib>:"Butterworth Filter PtByPt.vi"("initialize"=w804, "order"=w803, "filter type"=Filter_Passband_Type."Lowpass", "low cutoff freq: fl"=w806, "sampling freq: fs"=w808, "x"=w809) -> ("Filtered x"=w807:dbl)  [unwired: 3 in, 1 out]
                }
              }
              frame 55 {
                n120 = for {
                  tunnel: w810 -> [w823] mode=indexing
                  tunnel: w815 -> [w820]
                  tunnel: w816 -> [w822]
                  tunnel: [w821] -> w811 mode=indexing
                  tunnel: [w820] -> w814
                  tunnel: w813 -> [w818]
                  tunnel: w812 -> [w817]
                  n121 = call <vilib>:"Butterworth Filter PtByPt.vi"("initialize"=w818, "order"=w817, "filter type"=Filter_Passband_Type."Lowpass", "low cutoff freq: fl"=w820, "sampling freq: fs"=w822, "x"=w823) -> ("Filtered x"=w821:dbl)  [unwired: 3 in, 1 out]
                }
              }
              frame 56 {
                n122 = for {
                  tunnel: w824 -> [w837] mode=indexing
                  tunnel: w829 -> [w834]
                  tunnel: w830 -> [w836]
                  tunnel: [w835] -> w825 mode=indexing
                  tunnel: [w834] -> w828
                  tunnel: w827 -> [w832]
                  tunnel: w826 -> [w831]
                  n123 = call <vilib>:"Butterworth Filter PtByPt.vi"("initialize"=w832, "order"=w831, "filter type"=Filter_Passband_Type."Lowpass", "low cutoff freq: fl"=w834, "sampling freq: fs"=w836, "x"=w837) -> ("Filtered x"=w835:dbl)  [unwired: 3 in, 1 out]
                }
              }
              frame 57 {
                n124 = for {
                  tunnel: w838 -> [w851] mode=indexing
                  tunnel: w843 -> [w848]
                  tunnel: w844 -> [w850]
                  tunnel: [w849] -> w839 mode=indexing
                  tunnel: [w848] -> w842
                  tunnel: w841 -> [w846]
                  tunnel: w840 -> [w845]
                  n125 = call <vilib>:"Butterworth Filter PtByPt.vi"("initialize"=w846, "order"=w845, "filter type"=Filter_Passband_Type."Lowpass", "low cutoff freq: fl"=w848, "sampling freq: fs"=w850, "x"=w851) -> ("Filtered x"=w849:dbl)  [unwired: 3 in, 1 out]
                }
              }
              frame 58 {
                n126 = for {
                  tunnel: w852 -> [w865] mode=indexing
                  tunnel: w857 -> [w862]
                  tunnel: w858 -> [w864]
                  tunnel: [w863] -> w853 mode=indexing
                  tunnel: [w862] -> w856
                  tunnel: w855 -> [w860]
                  tunnel: w854 -> [w859]
                  n127 = call <vilib>:"Butterworth Filter PtByPt.vi"("initialize"=w860, "order"=w859, "filter type"=Filter_Passband_Type."Lowpass", "low cutoff freq: fl"=w862, "sampling freq: fs"=w864, "x"=w865) -> ("Filtered x"=w863:dbl)  [unwired: 3 in, 1 out]
                }
              }
              frame 59 {
                n128 = for {
                  tunnel: w866 -> [w879] mode=indexing
                  tunnel: w871 -> [w876]
                  tunnel: w872 -> [w878]
                  tunnel: [w877] -> w867 mode=indexing
                  tunnel: [w876] -> w870
                  tunnel: w869 -> [w874]
                  tunnel: w868 -> [w873]
                  n129 = call <vilib>:"Butterworth Filter PtByPt.vi"("initialize"=w874, "order"=w873, "filter type"=Filter_Passband_Type."Lowpass", "low cutoff freq: fl"=w876, "sampling freq: fs"=w878, "x"=w879) -> ("Filtered x"=w877:dbl)  [unwired: 3 in, 1 out]
                }
              }
              frame 60 {
                n130 = for {
                  tunnel: w880 -> [w893] mode=indexing
                  tunnel: w885 -> [w890]
                  tunnel: w886 -> [w892]
                  tunnel: [w891] -> w881 mode=indexing
                  tunnel: [w890] -> w884
                  tunnel: w883 -> [w888]
                  tunnel: w882 -> [w887]
                  n131 = call <vilib>:"Butterworth Filter PtByPt.vi"("initialize"=w888, "order"=w887, "filter type"=Filter_Passband_Type."Lowpass", "low cutoff freq: fl"=w890, "sampling freq: fs"=w892, "x"=w893) -> ("Filtered x"=w891:dbl)  [unwired: 3 in, 1 out]
                }
              }
              frame 61 {
                n132 = for {
                  tunnel: w894 -> [w907] mode=indexing
                  tunnel: w899 -> [w904]
                  tunnel: w900 -> [w906]
                  tunnel: [w905] -> w895 mode=indexing
                  tunnel: [w904] -> w898
                  tunnel: w897 -> [w902]
                  tunnel: w896 -> [w901]
                  n133 = call <vilib>:"Butterworth Filter PtByPt.vi"("initialize"=w902, "order"=w901, "filter type"=Filter_Passband_Type."Lowpass", "low cutoff freq: fl"=w904, "sampling freq: fs"=w906, "x"=w907) -> ("Filtered x"=w905:dbl)  [unwired: 3 in, 1 out]
                }
              }
              frame 62 {
                n134 = for {
                  tunnel: w908 -> [w921] mode=indexing
                  tunnel: w913 -> [w918]
                  tunnel: w914 -> [w920]
                  tunnel: [w919] -> w909 mode=indexing
                  tunnel: [w918] -> w912
                  tunnel: w911 -> [w916]
                  tunnel: w910 -> [w915]
                  n135 = call <vilib>:"Butterworth Filter PtByPt.vi"("initialize"=w916, "order"=w915, "filter type"=Filter_Passband_Type."Lowpass", "low cutoff freq: fl"=w918, "sampling freq: fs"=w920, "x"=w921) -> ("Filtered x"=w919:dbl)  [unwired: 3 in, 1 out]
                }
              }
              frame 63 {
                n136 = for {
                  tunnel: w922 -> [w935] mode=indexing
                  tunnel: w927 -> [w932]
                  tunnel: w928 -> [w934]
                  tunnel: [w933] -> w923 mode=indexing
                  tunnel: [w932] -> w926
                  tunnel: w925 -> [w930]
                  tunnel: w924 -> [w929]
                  n137 = call <vilib>:"Butterworth Filter PtByPt.vi"("initialize"=w930, "order"=w929, "filter type"=Filter_Passband_Type."Lowpass", "low cutoff freq: fl"=w932, "sampling freq: fs"=w934, "x"=w935) -> ("Filtered x"=w933:dbl)  [unwired: 3 in, 1 out]
                }
              }
              frame 64 {
                n138 = for {
                  tunnel: w936 -> [w949] mode=indexing
                  tunnel: w941 -> [w946]
                  tunnel: w942 -> [w948]
                  tunnel: [w947] -> w937 mode=indexing
                  tunnel: [w946] -> w940
                  tunnel: w939 -> [w944]
                  tunnel: w938 -> [w943]
                  n139 = call <vilib>:"Butterworth Filter PtByPt.vi"("initialize"=w944, "order"=w943, "filter type"=Filter_Passband_Type."Lowpass", "low cutoff freq: fl"=w946, "sampling freq: fs"=w948, "x"=w949) -> ("Filtered x"=w947:dbl)  [unwired: 3 in, 1 out]
                }
              }
              frame 65 {
                n140 = for {
                  tunnel: w950 -> [w963] mode=indexing
                  tunnel: w955 -> [w960]
                  tunnel: w956 -> [w962]
                  tunnel: [w961] -> w951 mode=indexing
                  tunnel: [w960] -> w954
                  tunnel: w953 -> [w958]
                  tunnel: w952 -> [w957]
                  n141 = call <vilib>:"Butterworth Filter PtByPt.vi"("initialize"=w958, "order"=w957, "filter type"=Filter_Passband_Type."Lowpass", "low cutoff freq: fl"=w960, "sampling freq: fs"=w962, "x"=w963) -> ("Filtered x"=w961:dbl)  [unwired: 3 in, 1 out]
                }
              }
              frame 66 {
                n142 = for {
                  tunnel: w964 -> [w977] mode=indexing
                  tunnel: w969 -> [w974]
                  tunnel: w970 -> [w976]
                  tunnel: [w975] -> w965 mode=indexing
                  tunnel: [w974] -> w968
                  tunnel: w967 -> [w972]
                  tunnel: w966 -> [w971]
                  n143 = call <vilib>:"Butterworth Filter PtByPt.vi"("initialize"=w972, "order"=w971, "filter type"=Filter_Passband_Type."Lowpass", "low cutoff freq: fl"=w974, "sampling freq: fs"=w976, "x"=w977) -> ("Filtered x"=w975:dbl)  [unwired: 3 in, 1 out]
                }
              }
              frame 67 {
                n144 = for {
                  tunnel: w978 -> [w991] mode=indexing
                  tunnel: w983 -> [w988]
                  tunnel: w984 -> [w990]
                  tunnel: [w989] -> w979 mode=indexing
                  tunnel: [w988] -> w982
                  tunnel: w981 -> [w986]
                  tunnel: w980 -> [w985]
                  n145 = call <vilib>:"Butterworth Filter PtByPt.vi"("initialize"=w986, "order"=w985, "filter type"=Filter_Passband_Type."Lowpass", "low cutoff freq: fl"=w988, "sampling freq: fs"=w990, "x"=w991) -> ("Filtered x"=w989:dbl)  [unwired: 3 in, 1 out]
                }
              }
              frame 68 {
                n146 = for {
                  tunnel: w992 -> [w1005] mode=indexing
                  tunnel: w997 -> [w1002]
                  tunnel: w998 -> [w1004]
                  tunnel: [w1003] -> w993 mode=indexing
                  tunnel: [w1002] -> w996
                  tunnel: w995 -> [w1000]
                  tunnel: w994 -> [w999]
                  n147 = call <vilib>:"Butterworth Filter PtByPt.vi"("initialize"=w1000, "order"=w999, "filter type"=Filter_Passband_Type."Lowpass", "low cutoff freq: fl"=w1002, "sampling freq: fs"=w1004, "x"=w1005) -> ("Filtered x"=w1003:dbl)  [unwired: 3 in, 1 out]
                }
              }
              frame 69 {
                n148 = for {
                  tunnel: w1006 -> [w1019] mode=indexing
                  tunnel: w1011 -> [w1016]
                  tunnel: w1012 -> [w1018]
                  tunnel: [w1017] -> w1007 mode=indexing
                  tunnel: [w1016] -> w1010
                  tunnel: w1009 -> [w1014]
                  tunnel: w1008 -> [w1013]
                  n149 = call <vilib>:"Butterworth Filter PtByPt.vi"("initialize"=w1014, "order"=w1013, "filter type"=Filter_Passband_Type."Lowpass", "low cutoff freq: fl"=w1016, "sampling freq: fs"=w1018, "x"=w1019) -> ("Filtered x"=w1017:dbl)  [unwired: 3 in, 1 out]
                }
              }
              frame 70 {
                n150 = for {
                  tunnel: w1020 -> [w1033] mode=indexing
                  tunnel: w1025 -> [w1030]
                  tunnel: w1026 -> [w1032]
                  tunnel: [w1031] -> w1021 mode=indexing
                  tunnel: [w1030] -> w1024
                  tunnel: w1023 -> [w1028]
                  tunnel: w1022 -> [w1027]
                  n151 = call <vilib>:"Butterworth Filter PtByPt.vi"("initialize"=w1028, "order"=w1027, "filter type"=Filter_Passband_Type."Lowpass", "low cutoff freq: fl"=w1030, "sampling freq: fs"=w1032, "x"=w1033) -> ("Filtered x"=w1031:dbl)  [unwired: 3 in, 1 out]
                }
              }
              frame 71 {
                n152 = for {
                  tunnel: w1034 -> [w1047] mode=indexing
                  tunnel: w1039 -> [w1044]
                  tunnel: w1040 -> [w1046]
                  tunnel: [w1045] -> w1035 mode=indexing
                  tunnel: [w1044] -> w1038
                  tunnel: w1037 -> [w1042]
                  tunnel: w1036 -> [w1041]
                  n153 = call <vilib>:"Butterworth Filter PtByPt.vi"("initialize"=w1042, "order"=w1041, "filter type"=Filter_Passband_Type."Lowpass", "low cutoff freq: fl"=w1044, "sampling freq: fs"=w1046, "x"=w1047) -> ("Filtered x"=w1045:dbl)  [unwired: 3 in, 1 out]
                }
              }
              frame 72 {
                n154 = for {
                  tunnel: w1048 -> [w1061] mode=indexing
                  tunnel: w1053 -> [w1058]
                  tunnel: w1054 -> [w1060]
                  tunnel: [w1059] -> w1049 mode=indexing
                  tunnel: [w1058] -> w1052
                  tunnel: w1051 -> [w1056]
                  tunnel: w1050 -> [w1055]
                  n155 = call <vilib>:"Butterworth Filter PtByPt.vi"("initialize"=w1056, "order"=w1055, "filter type"=Filter_Passband_Type."Lowpass", "low cutoff freq: fl"=w1058, "sampling freq: fs"=w1060, "x"=w1061) -> ("Filtered x"=w1059:dbl)  [unwired: 3 in, 1 out]
                }
              }
              frame 73 {
                n156 = for {
                  tunnel: w1062 -> [w1075] mode=indexing
                  tunnel: w1067 -> [w1072]
                  tunnel: w1068 -> [w1074]
                  tunnel: [w1073] -> w1063 mode=indexing
                  tunnel: [w1072] -> w1066
                  tunnel: w1065 -> [w1070]
                  tunnel: w1064 -> [w1069]
                  n157 = call <vilib>:"Butterworth Filter PtByPt.vi"("initialize"=w1070, "order"=w1069, "filter type"=Filter_Passband_Type."Lowpass", "low cutoff freq: fl"=w1072, "sampling freq: fs"=w1074, "x"=w1075) -> ("Filtered x"=w1073:dbl)  [unwired: 3 in, 1 out]
                }
              }
              frame 74 {
                n158 = for {
                  tunnel: w1076 -> [w1089] mode=indexing
                  tunnel: w1081 -> [w1086]
                  tunnel: w1082 -> [w1088]
                  tunnel: [w1087] -> w1077 mode=indexing
                  tunnel: [w1086] -> w1080
                  tunnel: w1079 -> [w1084]
                  tunnel: w1078 -> [w1083]
                  n159 = call <vilib>:"Butterworth Filter PtByPt.vi"("initialize"=w1084, "order"=w1083, "filter type"=Filter_Passband_Type."Lowpass", "low cutoff freq: fl"=w1086, "sampling freq: fs"=w1088, "x"=w1089) -> ("Filtered x"=w1087:dbl)  [unwired: 3 in, 1 out]
                }
              }
              frame 75 {
                n160 = for {
                  tunnel: w1090 -> [w1103] mode=indexing
                  tunnel: w1095 -> [w1100]
                  tunnel: w1096 -> [w1102]
                  tunnel: [w1101] -> w1091 mode=indexing
                  tunnel: [w1100] -> w1094
                  tunnel: w1093 -> [w1098]
                  tunnel: w1092 -> [w1097]
                  n161 = call <vilib>:"Butterworth Filter PtByPt.vi"("initialize"=w1098, "order"=w1097, "filter type"=Filter_Passband_Type."Lowpass", "low cutoff freq: fl"=w1100, "sampling freq: fs"=w1102, "x"=w1103) -> ("Filtered x"=w1101:dbl)  [unwired: 3 in, 1 out]
                }
              }
              frame 76 {
                n162 = for {
                  tunnel: w1104 -> [w1117] mode=indexing
                  tunnel: w1109 -> [w1114]
                  tunnel: w1110 -> [w1116]
                  tunnel: [w1115] -> w1105 mode=indexing
                  tunnel: [w1114] -> w1108
                  tunnel: w1107 -> [w1112]
                  tunnel: w1106 -> [w1111]
                  n163 = call <vilib>:"Butterworth Filter PtByPt.vi"("initialize"=w1112, "order"=w1111, "filter type"=Filter_Passband_Type."Lowpass", "low cutoff freq: fl"=w1114, "sampling freq: fs"=w1116, "x"=w1117) -> ("Filtered x"=w1115:dbl)  [unwired: 3 in, 1 out]
                }
              }
              frame 77 {
                n164 = for {
                  tunnel: w1118 -> [w1131] mode=indexing
                  tunnel: w1123 -> [w1128]
                  tunnel: w1124 -> [w1130]
                  tunnel: [w1129] -> w1119 mode=indexing
                  tunnel: [w1128] -> w1122
                  tunnel: w1121 -> [w1126]
                  tunnel: w1120 -> [w1125]
                  n165 = call <vilib>:"Butterworth Filter PtByPt.vi"("initialize"=w1126, "order"=w1125, "filter type"=Filter_Passband_Type."Lowpass", "low cutoff freq: fl"=w1128, "sampling freq: fs"=w1130, "x"=w1131) -> ("Filtered x"=w1129:dbl)  [unwired: 3 in, 1 out]
                }
              }
              frame 78 {
                n166 = for {
                  tunnel: w1132 -> [w1145] mode=indexing
                  tunnel: w1137 -> [w1142]
                  tunnel: w1138 -> [w1144]
                  tunnel: [w1143] -> w1133 mode=indexing
                  tunnel: [w1142] -> w1136
                  tunnel: w1135 -> [w1140]
                  tunnel: w1134 -> [w1139]
                  n167 = call <vilib>:"Butterworth Filter PtByPt.vi"("initialize"=w1140, "order"=w1139, "filter type"=Filter_Passband_Type."Lowpass", "low cutoff freq: fl"=w1142, "sampling freq: fs"=w1144, "x"=w1145) -> ("Filtered x"=w1143:dbl)  [unwired: 3 in, 1 out]
                }
              }
              frame 79 {
                n168 = for {
                  tunnel: w1146 -> [w1159] mode=indexing
                  tunnel: w1151 -> [w1156]
                  tunnel: w1152 -> [w1158]
                  tunnel: [w1157] -> w1147 mode=indexing
                  tunnel: [w1156] -> w1150
                  tunnel: w1149 -> [w1154]
                  tunnel: w1148 -> [w1153]
                  n169 = call <vilib>:"Butterworth Filter PtByPt.vi"("initialize"=w1154, "order"=w1153, "filter type"=Filter_Passband_Type."Lowpass", "low cutoff freq: fl"=w1156, "sampling freq: fs"=w1158, "x"=w1159) -> ("Filtered x"=w1157:dbl)  [unwired: 3 in, 1 out]
                }
              }
              frame 80 {
                n170 = for {
                  tunnel: w1160 -> [w1173] mode=indexing
                  tunnel: w1165 -> [w1170]
                  tunnel: w1166 -> [w1172]
                  tunnel: [w1171] -> w1161 mode=indexing
                  tunnel: [w1170] -> w1164
                  tunnel: w1163 -> [w1168]
                  tunnel: w1162 -> [w1167]
                  n171 = call <vilib>:"Butterworth Filter PtByPt.vi"("initialize"=w1168, "order"=w1167, "filter type"=Filter_Passband_Type."Lowpass", "low cutoff freq: fl"=w1170, "sampling freq: fs"=w1172, "x"=w1173) -> ("Filtered x"=w1171:dbl)  [unwired: 3 in, 1 out]
                }
              }
              frame 81 {
                n172 = for {
                  tunnel: w1174 -> [w1187] mode=indexing
                  tunnel: w1179 -> [w1184]
                  tunnel: w1180 -> [w1186]
                  tunnel: [w1185] -> w1175 mode=indexing
                  tunnel: [w1184] -> w1178
                  tunnel: w1177 -> [w1182]
                  tunnel: w1176 -> [w1181]
                  n173 = call <vilib>:"Butterworth Filter PtByPt.vi"("initialize"=w1182, "order"=w1181, "filter type"=Filter_Passband_Type."Lowpass", "low cutoff freq: fl"=w1184, "sampling freq: fs"=w1186, "x"=w1187) -> ("Filtered x"=w1185:dbl)  [unwired: 3 in, 1 out]
                }
              }
              frame 82 {
                n174 = for {
                  tunnel: w1188 -> [w1201] mode=indexing
                  tunnel: w1193 -> [w1198]
                  tunnel: w1194 -> [w1200]
                  tunnel: [w1199] -> w1189 mode=indexing
                  tunnel: [w1198] -> w1192
                  tunnel: w1191 -> [w1196]
                  tunnel: w1190 -> [w1195]
                  n175 = call <vilib>:"Butterworth Filter PtByPt.vi"("initialize"=w1196, "order"=w1195, "filter type"=Filter_Passband_Type."Lowpass", "low cutoff freq: fl"=w1198, "sampling freq: fs"=w1200, "x"=w1201) -> ("Filtered x"=w1199:dbl)  [unwired: 3 in, 1 out]
                }
              }
              frame 83 {
                n176 = for {
                  tunnel: w1202 -> [w1215] mode=indexing
                  tunnel: w1207 -> [w1212]
                  tunnel: w1208 -> [w1214]
                  tunnel: [w1213] -> w1203 mode=indexing
                  tunnel: [w1212] -> w1206
                  tunnel: w1205 -> [w1210]
                  tunnel: w1204 -> [w1209]
                  n177 = call <vilib>:"Butterworth Filter PtByPt.vi"("initialize"=w1210, "order"=w1209, "filter type"=Filter_Passband_Type."Lowpass", "low cutoff freq: fl"=w1212, "sampling freq: fs"=w1214, "x"=w1215) -> ("Filtered x"=w1213:dbl)  [unwired: 3 in, 1 out]
                }
              }
              frame 84 {
                n178 = for {
                  tunnel: w1216 -> [w1229] mode=indexing
                  tunnel: w1221 -> [w1226]
                  tunnel: w1222 -> [w1228]
                  tunnel: [w1227] -> w1217 mode=indexing
                  tunnel: [w1226] -> w1220
                  tunnel: w1219 -> [w1224]
                  tunnel: w1218 -> [w1223]
                  n179 = call <vilib>:"Butterworth Filter PtByPt.vi"("initialize"=w1224, "order"=w1223, "filter type"=Filter_Passband_Type."Lowpass", "low cutoff freq: fl"=w1226, "sampling freq: fs"=w1228, "x"=w1229) -> ("Filtered x"=w1227:dbl)  [unwired: 3 in, 1 out]
                }
              }
              frame 85 {
                n180 = for {
                  tunnel: w1230 -> [w1243] mode=indexing
                  tunnel: w1235 -> [w1240]
                  tunnel: w1236 -> [w1242]
                  tunnel: [w1241] -> w1231 mode=indexing
                  tunnel: [w1240] -> w1234
                  tunnel: w1233 -> [w1238]
                  tunnel: w1232 -> [w1237]
                  n181 = call <vilib>:"Butterworth Filter PtByPt.vi"("initialize"=w1238, "order"=w1237, "filter type"=Filter_Passband_Type."Lowpass", "low cutoff freq: fl"=w1240, "sampling freq: fs"=w1242, "x"=w1243) -> ("Filtered x"=w1241:dbl)  [unwired: 3 in, 1 out]
                }
              }
              frame 86 {
                n182 = for {
                  tunnel: w1244 -> [w1257] mode=indexing
                  tunnel: w1249 -> [w1254]
                  tunnel: w1250 -> [w1256]
                  tunnel: [w1255] -> w1245 mode=indexing
                  tunnel: [w1254] -> w1248
                  tunnel: w1247 -> [w1252]
                  tunnel: w1246 -> [w1251]
                  n183 = call <vilib>:"Butterworth Filter PtByPt.vi"("initialize"=w1252, "order"=w1251, "filter type"=Filter_Passband_Type."Lowpass", "low cutoff freq: fl"=w1254, "sampling freq: fs"=w1256, "x"=w1257) -> ("Filtered x"=w1255:dbl)  [unwired: 3 in, 1 out]
                }
              }
              frame 87 {
                n184 = for {
                  tunnel: w1258 -> [w1271] mode=indexing
                  tunnel: w1263 -> [w1268]
                  tunnel: w1264 -> [w1270]
                  tunnel: [w1269] -> w1259 mode=indexing
                  tunnel: [w1268] -> w1262
                  tunnel: w1261 -> [w1266]
                  tunnel: w1260 -> [w1265]
                  n185 = call <vilib>:"Butterworth Filter PtByPt.vi"("initialize"=w1266, "order"=w1265, "filter type"=Filter_Passband_Type."Lowpass", "low cutoff freq: fl"=w1268, "sampling freq: fs"=w1270, "x"=w1271) -> ("Filtered x"=w1269:dbl)  [unwired: 3 in, 1 out]
                }
              }
              frame 88 {
                n186 = for {
                  tunnel: w1272 -> [w1285] mode=indexing
                  tunnel: w1277 -> [w1282]
                  tunnel: w1278 -> [w1284]
                  tunnel: [w1283] -> w1273 mode=indexing
                  tunnel: [w1282] -> w1276
                  tunnel: w1275 -> [w1280]
                  tunnel: w1274 -> [w1279]
                  n187 = call <vilib>:"Butterworth Filter PtByPt.vi"("initialize"=w1280, "order"=w1279, "filter type"=Filter_Passband_Type."Lowpass", "low cutoff freq: fl"=w1282, "sampling freq: fs"=w1284, "x"=w1285) -> ("Filtered x"=w1283:dbl)  [unwired: 3 in, 1 out]
                }
              }
              frame 89 {
                n188 = for {
                  tunnel: w1286 -> [w1299] mode=indexing
                  tunnel: w1291 -> [w1296]
                  tunnel: w1292 -> [w1298]
                  tunnel: [w1297] -> w1287 mode=indexing
                  tunnel: [w1296] -> w1290
                  tunnel: w1289 -> [w1294]
                  tunnel: w1288 -> [w1293]
                  n189 = call <vilib>:"Butterworth Filter PtByPt.vi"("initialize"=w1294, "order"=w1293, "filter type"=Filter_Passband_Type."Lowpass", "low cutoff freq: fl"=w1296, "sampling freq: fs"=w1298, "x"=w1299) -> ("Filtered x"=w1297:dbl)  [unwired: 3 in, 1 out]
                }
              }
              frame 90 {
                n190 = for {
                  tunnel: w1300 -> [w1313] mode=indexing
                  tunnel: w1305 -> [w1310]
                  tunnel: w1306 -> [w1312]
                  tunnel: [w1311] -> w1301 mode=indexing
                  tunnel: [w1310] -> w1304
                  tunnel: w1303 -> [w1308]
                  tunnel: w1302 -> [w1307]
                  n191 = call <vilib>:"Butterworth Filter PtByPt.vi"("initialize"=w1308, "order"=w1307, "filter type"=Filter_Passband_Type."Lowpass", "low cutoff freq: fl"=w1310, "sampling freq: fs"=w1312, "x"=w1313) -> ("Filtered x"=w1311:dbl)  [unwired: 3 in, 1 out]
                }
              }
              frame 91 {
                n192 = for {
                  tunnel: w1314 -> [w1327] mode=indexing
                  tunnel: w1319 -> [w1324]
                  tunnel: w1320 -> [w1326]
                  tunnel: [w1325] -> w1315 mode=indexing
                  tunnel: [w1324] -> w1318
                  tunnel: w1317 -> [w1322]
                  tunnel: w1316 -> [w1321]
                  n193 = call <vilib>:"Butterworth Filter PtByPt.vi"("initialize"=w1322, "order"=w1321, "filter type"=Filter_Passband_Type."Lowpass", "low cutoff freq: fl"=w1324, "sampling freq: fs"=w1326, "x"=w1327) -> ("Filtered x"=w1325:dbl)  [unwired: 3 in, 1 out]
                }
              }
              frame 92 {
                n194 = for {
                  tunnel: w1328 -> [w1341] mode=indexing
                  tunnel: w1333 -> [w1338]
                  tunnel: w1334 -> [w1340]
                  tunnel: [w1339] -> w1329 mode=indexing
                  tunnel: [w1338] -> w1332
                  tunnel: w1331 -> [w1336]
                  tunnel: w1330 -> [w1335]
                  n195 = call <vilib>:"Butterworth Filter PtByPt.vi"("initialize"=w1336, "order"=w1335, "filter type"=Filter_Passband_Type."Lowpass", "low cutoff freq: fl"=w1338, "sampling freq: fs"=w1340, "x"=w1341) -> ("Filtered x"=w1339:dbl)  [unwired: 3 in, 1 out]
                }
              }
              frame 93 {
                n196 = for {
                  tunnel: w1342 -> [w1355] mode=indexing
                  tunnel: w1347 -> [w1352]
                  tunnel: w1348 -> [w1354]
                  tunnel: [w1353] -> w1343 mode=indexing
                  tunnel: [w1352] -> w1346
                  tunnel: w1345 -> [w1350]
                  tunnel: w1344 -> [w1349]
                  n197 = call <vilib>:"Butterworth Filter PtByPt.vi"("initialize"=w1350, "order"=w1349, "filter type"=Filter_Passband_Type."Lowpass", "low cutoff freq: fl"=w1352, "sampling freq: fs"=w1354, "x"=w1355) -> ("Filtered x"=w1353:dbl)  [unwired: 3 in, 1 out]
                }
              }
              frame 94 {
                n198 = for {
                  tunnel: w1356 -> [w1369] mode=indexing
                  tunnel: w1361 -> [w1366]
                  tunnel: w1362 -> [w1368]
                  tunnel: [w1367] -> w1357 mode=indexing
                  tunnel: [w1366] -> w1360
                  tunnel: w1359 -> [w1364]
                  tunnel: w1358 -> [w1363]
                  n199 = call <vilib>:"Butterworth Filter PtByPt.vi"("initialize"=w1364, "order"=w1363, "filter type"=Filter_Passband_Type."Lowpass", "low cutoff freq: fl"=w1366, "sampling freq: fs"=w1368, "x"=w1369) -> ("Filtered x"=w1367:dbl)  [unwired: 3 in, 1 out]
                }
              }
              frame 95 {
                n200 = for {
                  tunnel: w1370 -> [w1383] mode=indexing
                  tunnel: w1375 -> [w1380]
                  tunnel: w1376 -> [w1382]
                  tunnel: [w1381] -> w1371 mode=indexing
                  tunnel: [w1380] -> w1374
                  tunnel: w1373 -> [w1378]
                  tunnel: w1372 -> [w1377]
                  n201 = call <vilib>:"Butterworth Filter PtByPt.vi"("initialize"=w1378, "order"=w1377, "filter type"=Filter_Passband_Type."Lowpass", "low cutoff freq: fl"=w1380, "sampling freq: fs"=w1382, "x"=w1383) -> ("Filtered x"=w1381:dbl)  [unwired: 3 in, 1 out]
                }
              }
              frame 96 {
                n202 = for {
                  tunnel: w1384 -> [w1397] mode=indexing
                  tunnel: w1389 -> [w1394]
                  tunnel: w1390 -> [w1396]
                  tunnel: [w1395] -> w1385 mode=indexing
                  tunnel: [w1394] -> w1388
                  tunnel: w1387 -> [w1392]
                  tunnel: w1386 -> [w1391]
                  n203 = call <vilib>:"Butterworth Filter PtByPt.vi"("initialize"=w1392, "order"=w1391, "filter type"=Filter_Passband_Type."Lowpass", "low cutoff freq: fl"=w1394, "sampling freq: fs"=w1396, "x"=w1397) -> ("Filtered x"=w1395:dbl)  [unwired: 3 in, 1 out]
                }
              }
              frame 97 {
                n204 = for {
                  tunnel: w1398 -> [w1411] mode=indexing
                  tunnel: w1403 -> [w1408]
                  tunnel: w1404 -> [w1410]
                  tunnel: [w1409] -> w1399 mode=indexing
                  tunnel: [w1408] -> w1402
                  tunnel: w1401 -> [w1406]
                  tunnel: w1400 -> [w1405]
                  n205 = call <vilib>:"Butterworth Filter PtByPt.vi"("initialize"=w1406, "order"=w1405, "filter type"=Filter_Passband_Type."Lowpass", "low cutoff freq: fl"=w1408, "sampling freq: fs"=w1410, "x"=w1411) -> ("Filtered x"=w1409:dbl)  [unwired: 3 in, 1 out]
                }
              }
              frame 98 {
                n206 = for {
                  tunnel: w1412 -> [w1425] mode=indexing
                  tunnel: w1417 -> [w1422]
                  tunnel: w1418 -> [w1424]
                  tunnel: [w1423] -> w1413 mode=indexing
                  tunnel: [w1422] -> w1416
                  tunnel: w1415 -> [w1420]
                  tunnel: w1414 -> [w1419]
                  n207 = call <vilib>:"Butterworth Filter PtByPt.vi"("initialize"=w1420, "order"=w1419, "filter type"=Filter_Passband_Type."Lowpass", "low cutoff freq: fl"=w1422, "sampling freq: fs"=w1424, "x"=w1425) -> ("Filtered x"=w1423:dbl)  [unwired: 3 in, 1 out]
                }
              }
              frame 99 {
                n208 = for {
                  tunnel: w1426 -> [w1439] mode=indexing
                  tunnel: w1431 -> [w1436]
                  tunnel: w1432 -> [w1438]
                  tunnel: [w1437] -> w1427 mode=indexing
                  tunnel: [w1436] -> w1430
                  tunnel: w1429 -> [w1434]
                  tunnel: w1428 -> [w1433]
                  n209 = call <vilib>:"Butterworth Filter PtByPt.vi"("initialize"=w1434, "order"=w1433, "filter type"=Filter_Passband_Type."Lowpass", "low cutoff freq: fl"=w1436, "sampling freq: fs"=w1438, "x"=w1439) -> ("Filtered x"=w1437:dbl)  [unwired: 3 in, 1 out]
                }
              }
              frame 100 {
                n210 = for {
                  tunnel: w1440 -> [w1453] mode=indexing
                  tunnel: w1445 -> [w1450]
                  tunnel: w1446 -> [w1452]
                  tunnel: [w1451] -> w1441 mode=indexing
                  tunnel: [w1450] -> w1444
                  tunnel: w1443 -> [w1448]
                  tunnel: w1442 -> [w1447]
                  n211 = call <vilib>:"Butterworth Filter PtByPt.vi"("initialize"=w1448, "order"=w1447, "filter type"=Filter_Passband_Type."Lowpass", "low cutoff freq: fl"=w1450, "sampling freq: fs"=w1452, "x"=w1453) -> ("Filtered x"=w1451:dbl)  [unwired: 3 in, 1 out]
                }
              }
              frame 101 {
                n212 = for {
                  tunnel: w1454 -> [w1467] mode=indexing
                  tunnel: w1459 -> [w1464]
                  tunnel: w1460 -> [w1466]
                  tunnel: [w1465] -> w1455 mode=indexing
                  tunnel: [w1464] -> w1458
                  tunnel: w1457 -> [w1462]
                  tunnel: w1456 -> [w1461]
                  n213 = call <vilib>:"Butterworth Filter PtByPt.vi"("initialize"=w1462, "order"=w1461, "filter type"=Filter_Passband_Type."Lowpass", "low cutoff freq: fl"=w1464, "sampling freq: fs"=w1466, "x"=w1467) -> ("Filtered x"=w1465:dbl)  [unwired: 3 in, 1 out]
                }
              }
              frame 102 {
                n214 = for {
                  tunnel: w1468 -> [w1481] mode=indexing
                  tunnel: w1473 -> [w1478]
                  tunnel: w1474 -> [w1480]
                  tunnel: [w1479] -> w1469 mode=indexing
                  tunnel: [w1478] -> w1472
                  tunnel: w1471 -> [w1476]
                  tunnel: w1470 -> [w1475]
                  n215 = call <vilib>:"Butterworth Filter PtByPt.vi"("initialize"=w1476, "order"=w1475, "filter type"=Filter_Passband_Type."Lowpass", "low cutoff freq: fl"=w1478, "sampling freq: fs"=w1480, "x"=w1481) -> ("Filtered x"=w1479:dbl)  [unwired: 3 in, 1 out]
                }
              }
              frame 103 {
                n216 = for {
                  tunnel: w1482 -> [w1495] mode=indexing
                  tunnel: w1487 -> [w1492]
                  tunnel: w1488 -> [w1494]
                  tunnel: [w1493] -> w1483 mode=indexing
                  tunnel: [w1492] -> w1486
                  tunnel: w1485 -> [w1490]
                  tunnel: w1484 -> [w1489]
                  n217 = call <vilib>:"Butterworth Filter PtByPt.vi"("initialize"=w1490, "order"=w1489, "filter type"=Filter_Passband_Type."Lowpass", "low cutoff freq: fl"=w1492, "sampling freq: fs"=w1494, "x"=w1495) -> ("Filtered x"=w1493:dbl)  [unwired: 3 in, 1 out]
                }
              }
              frame 104 {
                n218 = for {
                  tunnel: w1496 -> [w1509] mode=indexing
                  tunnel: w1501 -> [w1506]
                  tunnel: w1502 -> [w1508]
                  tunnel: [w1507] -> w1497 mode=indexing
                  tunnel: [w1506] -> w1500
                  tunnel: w1499 -> [w1504]
                  tunnel: w1498 -> [w1503]
                  n219 = call <vilib>:"Butterworth Filter PtByPt.vi"("initialize"=w1504, "order"=w1503, "filter type"=Filter_Passband_Type."Lowpass", "low cutoff freq: fl"=w1506, "sampling freq: fs"=w1508, "x"=w1509) -> ("Filtered x"=w1507:dbl)  [unwired: 3 in, 1 out]
                }
              }
              frame 105 {
                n220 = for {
                  tunnel: w1510 -> [w1523] mode=indexing
                  tunnel: w1515 -> [w1520]
                  tunnel: w1516 -> [w1522]
                  tunnel: [w1521] -> w1511 mode=indexing
                  tunnel: [w1520] -> w1514
                  tunnel: w1513 -> [w1518]
                  tunnel: w1512 -> [w1517]
                  n221 = call <vilib>:"Butterworth Filter PtByPt.vi"("initialize"=w1518, "order"=w1517, "filter type"=Filter_Passband_Type."Lowpass", "low cutoff freq: fl"=w1520, "sampling freq: fs"=w1522, "x"=w1523) -> ("Filtered x"=w1521:dbl)  [unwired: 3 in, 1 out]
                }
              }
              frame 106 {
                n222 = for {
                  tunnel: w1524 -> [w1537] mode=indexing
                  tunnel: w1529 -> [w1534]
                  tunnel: w1530 -> [w1536]
                  tunnel: [w1535] -> w1525 mode=indexing
                  tunnel: [w1534] -> w1528
                  tunnel: w1527 -> [w1532]
                  tunnel: w1526 -> [w1531]
                  n223 = call <vilib>:"Butterworth Filter PtByPt.vi"("initialize"=w1532, "order"=w1531, "filter type"=Filter_Passband_Type."Lowpass", "low cutoff freq: fl"=w1534, "sampling freq: fs"=w1536, "x"=w1537) -> ("Filtered x"=w1535:dbl)  [unwired: 3 in, 1 out]
                }
              }
              frame 107 {
                n224 = for {
                  tunnel: w1538 -> [w1551] mode=indexing
                  tunnel: w1543 -> [w1548]
                  tunnel: w1544 -> [w1550]
                  tunnel: [w1549] -> w1539 mode=indexing
                  tunnel: [w1548] -> w1542
                  tunnel: w1541 -> [w1546]
                  tunnel: w1540 -> [w1545]
                  n225 = call <vilib>:"Butterworth Filter PtByPt.vi"("initialize"=w1546, "order"=w1545, "filter type"=Filter_Passband_Type."Lowpass", "low cutoff freq: fl"=w1548, "sampling freq: fs"=w1550, "x"=w1551) -> ("Filtered x"=w1549:dbl)  [unwired: 3 in, 1 out]
                }
              }
              frame 108 {
                n226 = for {
                  tunnel: w1552 -> [w1565] mode=indexing
                  tunnel: w1557 -> [w1562]
                  tunnel: w1558 -> [w1564]
                  tunnel: [w1563] -> w1553 mode=indexing
                  tunnel: [w1562] -> w1556
                  tunnel: w1555 -> [w1560]
                  tunnel: w1554 -> [w1559]
                  n227 = call <vilib>:"Butterworth Filter PtByPt.vi"("initialize"=w1560, "order"=w1559, "filter type"=Filter_Passband_Type."Lowpass", "low cutoff freq: fl"=w1562, "sampling freq: fs"=w1564, "x"=w1565) -> ("Filtered x"=w1563:dbl)  [unwired: 3 in, 1 out]
                }
              }
              frame 109 {
                n228 = for {
                  tunnel: w1566 -> [w1579] mode=indexing
                  tunnel: w1571 -> [w1576]
                  tunnel: w1572 -> [w1578]
                  tunnel: [w1577] -> w1567 mode=indexing
                  tunnel: [w1576] -> w1570
                  tunnel: w1569 -> [w1574]
                  tunnel: w1568 -> [w1573]
                  n229 = call <vilib>:"Butterworth Filter PtByPt.vi"("initialize"=w1574, "order"=w1573, "filter type"=Filter_Passband_Type."Lowpass", "low cutoff freq: fl"=w1576, "sampling freq: fs"=w1578, "x"=w1579) -> ("Filtered x"=w1577:dbl)  [unwired: 3 in, 1 out]
                }
              }
              frame 110 {
                n230 = for {
                  tunnel: w1580 -> [w1593] mode=indexing
                  tunnel: w1585 -> [w1590]
                  tunnel: w1586 -> [w1592]
                  tunnel: [w1591] -> w1581 mode=indexing
                  tunnel: [w1590] -> w1584
                  tunnel: w1583 -> [w1588]
                  tunnel: w1582 -> [w1587]
                  n231 = call <vilib>:"Butterworth Filter PtByPt.vi"("initialize"=w1588, "order"=w1587, "filter type"=Filter_Passband_Type."Lowpass", "low cutoff freq: fl"=w1590, "sampling freq: fs"=w1592, "x"=w1593) -> ("Filtered x"=w1591:dbl)  [unwired: 3 in, 1 out]
                }
              }
              frame 111 {
                n232 = for {
                  tunnel: w1594 -> [w1607] mode=indexing
                  tunnel: w1599 -> [w1604]
                  tunnel: w1600 -> [w1606]
                  tunnel: [w1605] -> w1595 mode=indexing
                  tunnel: [w1604] -> w1598
                  tunnel: w1597 -> [w1602]
                  tunnel: w1596 -> [w1601]
                  n233 = call <vilib>:"Butterworth Filter PtByPt.vi"("initialize"=w1602, "order"=w1601, "filter type"=Filter_Passband_Type."Lowpass", "low cutoff freq: fl"=w1604, "sampling freq: fs"=w1606, "x"=w1607) -> ("Filtered x"=w1605:dbl)  [unwired: 3 in, 1 out]
                }
              }
              frame 112 {
                n234 = for {
                  tunnel: w1608 -> [w1621] mode=indexing
                  tunnel: w1613 -> [w1618]
                  tunnel: w1614 -> [w1620]
                  tunnel: [w1619] -> w1609 mode=indexing
                  tunnel: [w1618] -> w1612
                  tunnel: w1611 -> [w1616]
                  tunnel: w1610 -> [w1615]
                  n235 = call <vilib>:"Butterworth Filter PtByPt.vi"("initialize"=w1616, "order"=w1615, "filter type"=Filter_Passband_Type."Lowpass", "low cutoff freq: fl"=w1618, "sampling freq: fs"=w1620, "x"=w1621) -> ("Filtered x"=w1619:dbl)  [unwired: 3 in, 1 out]
                }
              }
              frame 113 {
                n236 = for {
                  tunnel: w1622 -> [w1635] mode=indexing
                  tunnel: w1627 -> [w1632]
                  tunnel: w1628 -> [w1634]
                  tunnel: [w1633] -> w1623 mode=indexing
                  tunnel: [w1632] -> w1626
                  tunnel: w1625 -> [w1630]
                  tunnel: w1624 -> [w1629]
                  n237 = call <vilib>:"Butterworth Filter PtByPt.vi"("initialize"=w1630, "order"=w1629, "filter type"=Filter_Passband_Type."Lowpass", "low cutoff freq: fl"=w1632, "sampling freq: fs"=w1634, "x"=w1635) -> ("Filtered x"=w1633:dbl)  [unwired: 3 in, 1 out]
                }
              }
              frame 114 {
                n238 = for {
                  tunnel: w1636 -> [w1649] mode=indexing
                  tunnel: w1641 -> [w1646]
                  tunnel: w1642 -> [w1648]
                  tunnel: [w1647] -> w1637 mode=indexing
                  tunnel: [w1646] -> w1640
                  tunnel: w1639 -> [w1644]
                  tunnel: w1638 -> [w1643]
                  n239 = call <vilib>:"Butterworth Filter PtByPt.vi"("initialize"=w1644, "order"=w1643, "filter type"=Filter_Passband_Type."Lowpass", "low cutoff freq: fl"=w1646, "sampling freq: fs"=w1648, "x"=w1649) -> ("Filtered x"=w1647:dbl)  [unwired: 3 in, 1 out]
                }
              }
              frame 115 {
                n240 = for {
                  tunnel: w1650 -> [w1663] mode=indexing
                  tunnel: w1655 -> [w1660]
                  tunnel: w1656 -> [w1662]
                  tunnel: [w1661] -> w1651 mode=indexing
                  tunnel: [w1660] -> w1654
                  tunnel: w1653 -> [w1658]
                  tunnel: w1652 -> [w1657]
                  n241 = call <vilib>:"Butterworth Filter PtByPt.vi"("initialize"=w1658, "order"=w1657, "filter type"=Filter_Passband_Type."Lowpass", "low cutoff freq: fl"=w1660, "sampling freq: fs"=w1662, "x"=w1663) -> ("Filtered x"=w1661:dbl)  [unwired: 3 in, 1 out]
                }
              }
              frame 116 {
                n242 = for {
                  tunnel: w1664 -> [w1677] mode=indexing
                  tunnel: w1669 -> [w1674]
                  tunnel: w1670 -> [w1676]
                  tunnel: [w1675] -> w1665 mode=indexing
                  tunnel: [w1674] -> w1668
                  tunnel: w1667 -> [w1672]
                  tunnel: w1666 -> [w1671]
                  n243 = call <vilib>:"Butterworth Filter PtByPt.vi"("initialize"=w1672, "order"=w1671, "filter type"=Filter_Passband_Type."Lowpass", "low cutoff freq: fl"=w1674, "sampling freq: fs"=w1676, "x"=w1677) -> ("Filtered x"=w1675:dbl)  [unwired: 3 in, 1 out]
                }
              }
              frame 117 {
                n244 = for {
                  tunnel: w1678 -> [w1691] mode=indexing
                  tunnel: w1683 -> [w1688]
                  tunnel: w1684 -> [w1690]
                  tunnel: [w1689] -> w1679 mode=indexing
                  tunnel: [w1688] -> w1682
                  tunnel: w1681 -> [w1686]
                  tunnel: w1680 -> [w1685]
                  n245 = call <vilib>:"Butterworth Filter PtByPt.vi"("initialize"=w1686, "order"=w1685, "filter type"=Filter_Passband_Type."Lowpass", "low cutoff freq: fl"=w1688, "sampling freq: fs"=w1690, "x"=w1691) -> ("Filtered x"=w1689:dbl)  [unwired: 3 in, 1 out]
                }
              }
              frame 118 {
                n246 = for {
                  tunnel: w1692 -> [w1705] mode=indexing
                  tunnel: w1697 -> [w1702]
                  tunnel: w1698 -> [w1704]
                  tunnel: [w1703] -> w1693 mode=indexing
                  tunnel: [w1702] -> w1696
                  tunnel: w1695 -> [w1700]
                  tunnel: w1694 -> [w1699]
                  n247 = call <vilib>:"Butterworth Filter PtByPt.vi"("initialize"=w1700, "order"=w1699, "filter type"=Filter_Passband_Type."Lowpass", "low cutoff freq: fl"=w1702, "sampling freq: fs"=w1704, "x"=w1705) -> ("Filtered x"=w1703:dbl)  [unwired: 3 in, 1 out]
                }
              }
              frame 119 {
                n248 = for {
                  tunnel: w1706 -> [w1719] mode=indexing
                  tunnel: w1711 -> [w1716]
                  tunnel: w1712 -> [w1718]
                  tunnel: [w1717] -> w1707 mode=indexing
                  tunnel: [w1716] -> w1710
                  tunnel: w1709 -> [w1714]
                  tunnel: w1708 -> [w1713]
                  n249 = call <vilib>:"Butterworth Filter PtByPt.vi"("initialize"=w1714, "order"=w1713, "filter type"=Filter_Passband_Type."Lowpass", "low cutoff freq: fl"=w1716, "sampling freq: fs"=w1718, "x"=w1719) -> ("Filtered x"=w1717:dbl)  [unwired: 3 in, 1 out]
                }
              }
              frame 120 {
                n250 = for {
                  tunnel: w1720 -> [w1733] mode=indexing
                  tunnel: w1725 -> [w1730]
                  tunnel: w1726 -> [w1732]
                  tunnel: [w1731] -> w1721 mode=indexing
                  tunnel: [w1730] -> w1724
                  tunnel: w1723 -> [w1728]
                  tunnel: w1722 -> [w1727]
                  n251 = call <vilib>:"Butterworth Filter PtByPt.vi"("initialize"=w1728, "order"=w1727, "filter type"=Filter_Passband_Type."Lowpass", "low cutoff freq: fl"=w1730, "sampling freq: fs"=w1732, "x"=w1733) -> ("Filtered x"=w1731:dbl)  [unwired: 3 in, 1 out]
                }
              }
              frame 121 {
                n252 = for {
                  tunnel: w1734 -> [w1747] mode=indexing
                  tunnel: w1739 -> [w1744]
                  tunnel: w1740 -> [w1746]
                  tunnel: [w1745] -> w1735 mode=indexing
                  tunnel: [w1744] -> w1738
                  tunnel: w1737 -> [w1742]
                  tunnel: w1736 -> [w1741]
                  n253 = call <vilib>:"Butterworth Filter PtByPt.vi"("initialize"=w1742, "order"=w1741, "filter type"=Filter_Passband_Type."Lowpass", "low cutoff freq: fl"=w1744, "sampling freq: fs"=w1746, "x"=w1747) -> ("Filtered x"=w1745:dbl)  [unwired: 3 in, 1 out]
                }
              }
              frame 122 {
                n254 = for {
                  tunnel: w1748 -> [w1761] mode=indexing
                  tunnel: w1753 -> [w1758]
                  tunnel: w1754 -> [w1760]
                  tunnel: [w1759] -> w1749 mode=indexing
                  tunnel: [w1758] -> w1752
                  tunnel: w1751 -> [w1756]
                  tunnel: w1750 -> [w1755]
                  n255 = call <vilib>:"Butterworth Filter PtByPt.vi"("initialize"=w1756, "order"=w1755, "filter type"=Filter_Passband_Type."Lowpass", "low cutoff freq: fl"=w1758, "sampling freq: fs"=w1760, "x"=w1761) -> ("Filtered x"=w1759:dbl)  [unwired: 3 in, 1 out]
                }
              }
              frame 123 {
                n256 = for {
                  tunnel: w1762 -> [w1775] mode=indexing
                  tunnel: w1767 -> [w1772]
                  tunnel: w1768 -> [w1774]
                  tunnel: [w1773] -> w1763 mode=indexing
                  tunnel: [w1772] -> w1766
                  tunnel: w1765 -> [w1770]
                  tunnel: w1764 -> [w1769]
                  n257 = call <vilib>:"Butterworth Filter PtByPt.vi"("initialize"=w1770, "order"=w1769, "filter type"=Filter_Passband_Type."Lowpass", "low cutoff freq: fl"=w1772, "sampling freq: fs"=w1774, "x"=w1775) -> ("Filtered x"=w1773:dbl)  [unwired: 3 in, 1 out]
                }
              }
            }
            n258 = Bundle By Name(cluster=w31, "Y"=w34) -> (w30:waveform(dbl))
            n259 = in-place-array #1(w30) -> (w22:waveform(dbl)[])  [unwired: 1 out]
          }
        }
      }
    }
    frame "method 2" {
      # "For loop access each channel"
      # "While loop is used to store the previous low cutoff frequency fl. If fl changes reset the filter history."
      # "Each case is for a different lockin channel. The Butterworth Filter Pt by Pt in each case has its own history (Preallocated clone reentrant execution)."
      # "method 2: how to not use case structure? How to not use Pt by Pt filter?"
      n260 = while {
        tunnel: w1780 -> [w1781]
        tunnel: [w1790] -> w1779
        tunnel: w1778 -> [w1787]
        tunnel: w1777 -> [w1784]
        shift-right: [w1788] -> _
        shift-left: _ -> [w1786]
        tunnel: w1776 -> [w1785]
        stop <- TRUE stop-if-true
        n261 = Array Size(array=w1781) -> (size(s)=w1782:i32)
        n262 = Not Equal?(x=w1786, y=w1784) -> (x != y?=w1783:bool)
        n263 = for {
          N: w1782 -> [_]
          tunnel: w1787 -> [w1798]
          tunnel: w1784 -> [w1797]
          tunnel: [w1796] -> w1788
          tunnel: w1783 -> [w1795]
          tunnel: w1785 -> [w1794]
          shift-right: [w1791] -> w1790
          shift-left: w1781 -> [w1793]
          i -> [w1792]
          n264 = in-place {
            in-place-border: w1798 -> [w1808]
            in-place-border: w1797 -> [w1807]
            in-place-border: [w1806] -> w1796
            in-place-border: w1795 -> [w1805]
            in-place-border: w1794 -> [w1804]
            in-place-border: w1792 -> [w1801]
            n265 = in-place-array #2(w1793, w1792) -> (w1800:waveform(dbl))
            n266 = Unbundle By Name(w1800) -> ("Y"=w1802:dbl[])
            n267 = case shown="0, Default" w1801 {
              tunnel: w1808 -> [w1815 w1822 w1829 w1836 w1843 w1850 w1857 w1864 w1871 w1885 w1899 w1913 w1927 w1941 w1955 w1969 w1983 w1997 w2011 w2025 w2039 w2053 w2067 w2081 w2095 w2109 w2123 w2137 w2151 w2165 w2179 w2193 w2207 w2221 w2235 w2249 w2263 w2277 w2291 w2305 w2319 w2333 w2347 w2361 w2375 w2389 w2403 w2417 w2431 w2445 w2459 w2473 w2487 w2501 w2515 w2529 w2543 w2557 w2571 w2585 w2599 w2613 w2627 w2641 w2655 w2669 w2683 w2697 w2711 w2725 w2739 w2753 w2767 w2781 w2795 w2809 w2823 w2837 w2851 w2865 w2879 w2893 w2907 w2921 w2935 w2949 w2963 w2977 w2991 w3005 w3019 w3033 w3047 w3061 w3075 w3089 w3103 w3117 w3131 w3145 w3159 w3173 w3187 w3201 w3215 w3229 w3243 w3257 w3271 w3285 w3299 w3313 w3327 w3341 w3355 w3369 w3383 w3397 w3411 w3425 w3439 w3453 w3467 w3481]
              tunnel: w1807 -> [w1814 w1821 w1828 w1835 w1842 w1849 w1856 w1863 w1870 w1884 w1898 w1912 w1926 w1940 w1954 w1968 w1982 w1996 w2010 w2024 w2038 w2052 w2066 w2080 w2094 w2108 w2122 w2136 w2150 w2164 w2178 w2192 w2206 w2220 w2234 w2248 w2262 w2276 w2290 w2304 w2318 w2332 w2346 w2360 w2374 w2388 w2402 w2416 w2430 w2444 w2458 w2472 w2486 w2500 w2514 w2528 w2542 w2556 w2570 w2584 w2598 w2612 w2626 w2640 w2654 w2668 w2682 w2696 w2710 w2724 w2738 w2752 w2766 w2780 w2794 w2808 w2822 w2836 w2850 w2864 w2878 w2892 w2906 w2920 w2934 w2948 w2962 w2976 w2990 w3004 w3018 w3032 w3046 w3060 w3074 w3088 w3102 w3116 w3130 w3144 w3158 w3172 w3186 w3200 w3214 w3228 w3242 w3256 w3270 w3284 w3298 w3312 w3326 w3340 w3354 w3368 w3382 w3396 w3410 w3424 w3438 w3452 w3466 w3480]
              tunnel: [w1814 w1821 w1828 w1835 w1842 w1849 w1856 w1863 w1869 w1883 w1897 w1911 w1925 w1939 w1953 w1967 w1981 w1995 w2009 w2023 w2037 w2051 w2065 w2079 w2093 w2107 w2121 w2135 w2149 w2163 w2177 w2191 w2205 w2219 w2233 w2247 w2261 w2275 w2289 w2303 w2317 w2331 w2345 w2359 w2373 w2387 w2401 w2415 w2429 w2443 w2457 w2471 w2485 w2499 w2513 w2527 w2541 w2555 w2569 w2583 w2597 w2611 w2625 w2639 w2653 w2667 w2681 w2695 w2709 w2723 w2737 w2751 w2765 w2779 w2793 w2807 w2821 w2835 w2849 w2863 w2877 w2891 w2905 w2919 w2933 w2947 w2961 w2975 w2989 w3003 w3017 w3031 w3045 w3059 w3073 w3087 w3101 w3115 w3129 w3143 w3157 w3171 w3185 w3199 w3213 w3227 w3241 w3255 w3269 w3283 w3297 w3311 w3325 w3339 w3353 w3367 w3381 w3395 w3409 w3423 w3437 w3451 w3465 w3479] -> w1806
              tunnel: w1805 -> [w1813 w1820 w1827 w1834 w1841 w1848 w1855 w1862 w1868 w1882 w1896 w1910 w1924 w1938 w1952 w1966 w1980 w1994 w2008 w2022 w2036 w2050 w2064 w2078 w2092 w2106 w2120 w2134 w2148 w2162 w2176 w2190 w2204 w2218 w2232 w2246 w2260 w2274 w2288 w2302 w2316 w2330 w2344 w2358 w2372 w2386 w2400 w2414 w2428 w2442 w2456 w2470 w2484 w2498 w2512 w2526 w2540 w2554 w2568 w2582 w2596 w2610 w2624 w2638 w2652 w2666 w2680 w2694 w2708 w2722 w2736 w2750 w2764 w2778 w2792 w2806 w2820 w2834 w2848 w2862 w2876 w2890 w2904 w2918 w2932 w2946 w2960 w2974 w2988 w3002 w3016 w3030 w3044 w3058 w3072 w3086 w3100 w3114 w3128 w3142 w3156 w3170 w3184 w3198 w3212 w3226 w3240 w3254 w3268 w3282 w3296 w3310 w3324 w3338 w3352 w3366 w3380 w3394 w3408 w3422 w3436 w3450 w3464 w3478]
              tunnel: w1804 -> [w1812 w1819 w1826 w1833 w1840 w1847 w1854 w1861 w1867 w1881 w1895 w1909 w1923 w1937 w1951 w1965 w1979 w1993 w2007 w2021 w2035 w2049 w2063 w2077 w2091 w2105 w2119 w2133 w2147 w2161 w2175 w2189 w2203 w2217 w2231 w2245 w2259 w2273 w2287 w2301 w2315 w2329 w2343 w2357 w2371 w2385 w2399 w2413 w2427 w2441 w2455 w2469 w2483 w2497 w2511 w2525 w2539 w2553 w2567 w2581 w2595 w2609 w2623 w2637 w2651 w2665 w2679 w2693 w2707 w2721 w2735 w2749 w2763 w2777 w2791 w2805 w2819 w2833 w2847 w2861 w2875 w2889 w2903 w2917 w2931 w2945 w2959 w2973 w2987 w3001 w3015 w3029 w3043 w3057 w3071 w3085 w3099 w3113 w3127 w3141 w3155 w3169 w3183 w3197 w3211 w3225 w3239 w3253 w3267 w3281 w3295 w3309 w3323 w3337 w3351 w3365 w3379 w3393 w3407 w3421 w3435 w3449 w3463 w3477]
              tunnel: [w1809 w1816 w1823 w1830 w1837 w1844 w1851 w1858 w1866 w1880 w1894 w1908 w1922 w1936 w1950 w1964 w1978 w1992 w2006 w2020 w2034 w2048 w2062 w2076 w2090 w2104 w2118 w2132 w2146 w2160 w2174 w2188 w2202 w2216 w2230 w2244 w2258 w2272 w2286 w2300 w2314 w2328 w2342 w2356 w2370 w2384 w2398 w2412 w2426 w2440 w2454 w2468 w2482 w2496 w2510 w2524 w2538 w2552 w2566 w2580 w2594 w2608 w2622 w2636 w2650 w2664 w2678 w2692 w2706 w2720 w2734 w2748 w2762 w2776 w2790 w2804 w2818 w2832 w2846 w2860 w2874 w2888 w2902 w2916 w2930 w2944 w2958 w2972 w2986 w3000 w3014 w3028 w3042 w3056 w3070 w3084 w3098 w3112 w3126 w3140 w3154 w3168 w3182 w3196 w3210 w3224 w3238 w3252 w3266 w3280 w3294 w3308 w3322 w3336 w3350 w3364 w3378 w3392 w3406 w3420 w3434 w3448 w3462 w3476] -> w1803
              tunnel: w1802 -> [w1810 w1817 w1824 w1831 w1838 w1845 w1852 w1859 w1865 w1879 w1893 w1907 w1921 w1935 w1949 w1963 w1977 w1991 w2005 w2019 w2033 w2047 w2061 w2075 w2089 w2103 w2117 w2131 w2145 w2159 w2173 w2187 w2201 w2215 w2229 w2243 w2257 w2271 w2285 w2299 w2313 w2327 w2341 w2355 w2369 w2383 w2397 w2411 w2425 w2439 w2453 w2467 w2481 w2495 w2509 w2523 w2537 w2551 w2565 w2579 w2593 w2607 w2621 w2635 w2649 w2663 w2677 w2691 w2705 w2719 w2733 w2747 w2761 w2775 w2789 w2803 w2817 w2831 w2845 w2859 w2873 w2887 w2901 w2915 w2929 w2943 w2957 w2971 w2985 w2999 w3013 w3027 w3041 w3055 w3069 w3083 w3097 w3111 w3125 w3139 w3153 w3167 w3181 w3195 w3209 w3223 w3237 w3251 w3265 w3279 w3293 w3307 w3321 w3335 w3349 w3363 w3377 w3391 w3405 w3419 w3433 w3447 w3461 w3475]
              frame 0, Default {
                n268 = call-poly <vilib>:"Butterworth Filter.vi"("init/cont (init:F)"=w1813, "order"=w1812, "filter type"=Filter_Passband_Type."Lowpass", "low cutoff freq: fl"=w1814, "sampling freq: fs"=w1815, "X"=w1810) -> ("Filtered X"=w1809:dbl[])  [unwired: 2 in, 1 out]
              }
              frame 1 {
                n269 = call-poly <vilib>:"Butterworth Filter.vi"("init/cont (init:F)"=w1820, "order"=w1819, "filter type"=Filter_Passband_Type."Lowpass", "low cutoff freq: fl"=w1821, "sampling freq: fs"=w1822, "X"=w1817) -> ("Filtered X"=w1816:dbl[])  [unwired: 2 in, 1 out]
              }
              frame 2 {
                n270 = call-poly <vilib>:"Butterworth Filter.vi"("init/cont (init:F)"=w1827, "order"=w1826, "filter type"=Filter_Passband_Type."Lowpass", "low cutoff freq: fl"=w1828, "sampling freq: fs"=w1829, "X"=w1824) -> ("Filtered X"=w1823:dbl[])  [unwired: 2 in, 1 out]
              }
              frame 3 {
                n271 = call-poly <vilib>:"Butterworth Filter.vi"("init/cont (init:F)"=w1834, "order"=w1833, "filter type"=Filter_Passband_Type."Lowpass", "low cutoff freq: fl"=w1835, "sampling freq: fs"=w1836, "X"=w1831) -> ("Filtered X"=w1830:dbl[])  [unwired: 2 in, 1 out]
              }
              frame 4 {
                n272 = call-poly <vilib>:"Butterworth Filter.vi"("init/cont (init:F)"=w1841, "order"=w1840, "filter type"=Filter_Passband_Type."Lowpass", "low cutoff freq: fl"=w1842, "sampling freq: fs"=w1843, "X"=w1838) -> ("Filtered X"=w1837:dbl[])  [unwired: 2 in, 1 out]
              }
              frame 5 {
                n273 = call-poly <vilib>:"Butterworth Filter.vi"("init/cont (init:F)"=w1848, "order"=w1847, "filter type"=Filter_Passband_Type."Lowpass", "low cutoff freq: fl"=w1849, "sampling freq: fs"=w1850, "X"=w1845) -> ("Filtered X"=w1844:dbl[])  [unwired: 2 in, 1 out]
              }
              frame 6 {
                n274 = call-poly <vilib>:"Butterworth Filter.vi"("init/cont (init:F)"=w1855, "order"=w1854, "filter type"=Filter_Passband_Type."Lowpass", "low cutoff freq: fl"=w1856, "sampling freq: fs"=w1857, "X"=w1852) -> ("Filtered X"=w1851:dbl[])  [unwired: 2 in, 1 out]
              }
              frame 7 {
                n275 = call-poly <vilib>:"Butterworth Filter.vi"("init/cont (init:F)"=w1862, "order"=w1861, "filter type"=Filter_Passband_Type."Lowpass", "low cutoff freq: fl"=w1863, "sampling freq: fs"=w1864, "X"=w1859) -> ("Filtered X"=w1858:dbl[])  [unwired: 2 in, 1 out]
              }
              frame 8 {
                n276 = for {
                  tunnel: w1865 -> [w1878] mode=indexing
                  tunnel: w1870 -> [w1875]
                  tunnel: w1871 -> [w1877]
                  tunnel: [w1876] -> w1866 mode=indexing
                  tunnel: [w1875] -> w1869
                  tunnel: w1868 -> [w1873]
                  tunnel: w1867 -> [w1872]
                  n277 = call <vilib>:"Butterworth Filter PtByPt.vi"("initialize"=w1873, "order"=w1872, "filter type"=Filter_Passband_Type."Lowpass", "low cutoff freq: fl"=w1875, "sampling freq: fs"=w1877, "x"=w1878) -> ("Filtered x"=w1876:dbl)  [unwired: 3 in, 1 out]
                }
              }
              frame 9 {
                n278 = for {
                  tunnel: w1879 -> [w1892] mode=indexing
                  tunnel: w1884 -> [w1889]
                  tunnel: w1885 -> [w1891]
                  tunnel: [w1890] -> w1880 mode=indexing
                  tunnel: [w1889] -> w1883
                  tunnel: w1882 -> [w1887]
                  tunnel: w1881 -> [w1886]
                  n279 = call <vilib>:"Butterworth Filter PtByPt.vi"("initialize"=w1887, "order"=w1886, "filter type"=Filter_Passband_Type."Lowpass", "low cutoff freq: fl"=w1889, "sampling freq: fs"=w1891, "x"=w1892) -> ("Filtered x"=w1890:dbl)  [unwired: 3 in, 1 out]
                }
              }
              frame 10 {
                n280 = for {
                  tunnel: w1893 -> [w1906] mode=indexing
                  tunnel: w1898 -> [w1903]
                  tunnel: w1899 -> [w1905]
                  tunnel: [w1904] -> w1894 mode=indexing
                  tunnel: [w1903] -> w1897
                  tunnel: w1896 -> [w1901]
                  tunnel: w1895 -> [w1900]
                  n281 = call <vilib>:"Butterworth Filter PtByPt.vi"("initialize"=w1901, "order"=w1900, "filter type"=Filter_Passband_Type."Lowpass", "low cutoff freq: fl"=w1903, "sampling freq: fs"=w1905, "x"=w1906) -> ("Filtered x"=w1904:dbl)  [unwired: 3 in, 1 out]
                }
              }
              frame 11 {
                n282 = for {
                  tunnel: w1907 -> [w1920] mode=indexing
                  tunnel: w1912 -> [w1917]
                  tunnel: w1913 -> [w1919]
                  tunnel: [w1918] -> w1908 mode=indexing
                  tunnel: [w1917] -> w1911
                  tunnel: w1910 -> [w1915]
                  tunnel: w1909 -> [w1914]
                  n283 = call <vilib>:"Butterworth Filter PtByPt.vi"("initialize"=w1915, "order"=w1914, "filter type"=Filter_Passband_Type."Lowpass", "low cutoff freq: fl"=w1917, "sampling freq: fs"=w1919, "x"=w1920) -> ("Filtered x"=w1918:dbl)  [unwired: 3 in, 1 out]
                }
              }
              frame 12 {
                n284 = for {
                  tunnel: w1921 -> [w1934] mode=indexing
                  tunnel: w1926 -> [w1931]
                  tunnel: w1927 -> [w1933]
                  tunnel: [w1932] -> w1922 mode=indexing
                  tunnel: [w1931] -> w1925
                  tunnel: w1924 -> [w1929]
                  tunnel: w1923 -> [w1928]
                  n285 = call <vilib>:"Butterworth Filter PtByPt.vi"("initialize"=w1929, "order"=w1928, "filter type"=Filter_Passband_Type."Lowpass", "low cutoff freq: fl"=w1931, "sampling freq: fs"=w1933, "x"=w1934) -> ("Filtered x"=w1932:dbl)  [unwired: 3 in, 1 out]
                }
              }
              frame 13 {
                n286 = for {
                  tunnel: w1935 -> [w1948] mode=indexing
                  tunnel: w1940 -> [w1945]
                  tunnel: w1941 -> [w1947]
                  tunnel: [w1946] -> w1936 mode=indexing
                  tunnel: [w1945] -> w1939
                  tunnel: w1938 -> [w1943]
                  tunnel: w1937 -> [w1942]
                  n287 = call <vilib>:"Butterworth Filter PtByPt.vi"("initialize"=w1943, "order"=w1942, "filter type"=Filter_Passband_Type."Lowpass", "low cutoff freq: fl"=w1945, "sampling freq: fs"=w1947, "x"=w1948) -> ("Filtered x"=w1946:dbl)  [unwired: 3 in, 1 out]
                }
              }
              frame 14 {
                n288 = for {
                  tunnel: w1949 -> [w1962] mode=indexing
                  tunnel: w1954 -> [w1959]
                  tunnel: w1955 -> [w1961]
                  tunnel: [w1960] -> w1950 mode=indexing
                  tunnel: [w1959] -> w1953
                  tunnel: w1952 -> [w1957]
                  tunnel: w1951 -> [w1956]
                  n289 = call <vilib>:"Butterworth Filter PtByPt.vi"("initialize"=w1957, "order"=w1956, "filter type"=Filter_Passband_Type."Lowpass", "low cutoff freq: fl"=w1959, "sampling freq: fs"=w1961, "x"=w1962) -> ("Filtered x"=w1960:dbl)  [unwired: 3 in, 1 out]
                }
              }
              frame 15 {
                n290 = for {
                  tunnel: w1963 -> [w1976] mode=indexing
                  tunnel: w1968 -> [w1973]
                  tunnel: w1969 -> [w1975]
                  tunnel: [w1974] -> w1964 mode=indexing
                  tunnel: [w1973] -> w1967
                  tunnel: w1966 -> [w1971]
                  tunnel: w1965 -> [w1970]
                  n291 = call <vilib>:"Butterworth Filter PtByPt.vi"("initialize"=w1971, "order"=w1970, "filter type"=Filter_Passband_Type."Lowpass", "low cutoff freq: fl"=w1973, "sampling freq: fs"=w1975, "x"=w1976) -> ("Filtered x"=w1974:dbl)  [unwired: 3 in, 1 out]
                }
              }
              frame 16 {
                n292 = for {
                  tunnel: w1977 -> [w1990] mode=indexing
                  tunnel: w1982 -> [w1987]
                  tunnel: w1983 -> [w1989]
                  tunnel: [w1988] -> w1978 mode=indexing
                  tunnel: [w1987] -> w1981
                  tunnel: w1980 -> [w1985]
                  tunnel: w1979 -> [w1984]
                  n293 = call <vilib>:"Butterworth Filter PtByPt.vi"("initialize"=w1985, "order"=w1984, "filter type"=Filter_Passband_Type."Lowpass", "low cutoff freq: fl"=w1987, "sampling freq: fs"=w1989, "x"=w1990) -> ("Filtered x"=w1988:dbl)  [unwired: 3 in, 1 out]
                }
              }
              frame 17 {
                n294 = for {
                  tunnel: w1991 -> [w2004] mode=indexing
                  tunnel: w1996 -> [w2001]
                  tunnel: w1997 -> [w2003]
                  tunnel: [w2002] -> w1992 mode=indexing
                  tunnel: [w2001] -> w1995
                  tunnel: w1994 -> [w1999]
                  tunnel: w1993 -> [w1998]
                  n295 = call <vilib>:"Butterworth Filter PtByPt.vi"("initialize"=w1999, "order"=w1998, "filter type"=Filter_Passband_Type."Lowpass", "low cutoff freq: fl"=w2001, "sampling freq: fs"=w2003, "x"=w2004) -> ("Filtered x"=w2002:dbl)  [unwired: 3 in, 1 out]
                }
              }
              frame 18 {
                n296 = for {
                  tunnel: w2005 -> [w2018] mode=indexing
                  tunnel: w2010 -> [w2015]
                  tunnel: w2011 -> [w2017]
                  tunnel: [w2016] -> w2006 mode=indexing
                  tunnel: [w2015] -> w2009
                  tunnel: w2008 -> [w2013]
                  tunnel: w2007 -> [w2012]
                  n297 = call <vilib>:"Butterworth Filter PtByPt.vi"("initialize"=w2013, "order"=w2012, "filter type"=Filter_Passband_Type."Lowpass", "low cutoff freq: fl"=w2015, "sampling freq: fs"=w2017, "x"=w2018) -> ("Filtered x"=w2016:dbl)  [unwired: 3 in, 1 out]
                }
              }
              frame 19 {
                n298 = for {
                  tunnel: w2019 -> [w2032] mode=indexing
                  tunnel: w2024 -> [w2029]
                  tunnel: w2025 -> [w2031]
                  tunnel: [w2030] -> w2020 mode=indexing
                  tunnel: [w2029] -> w2023
                  tunnel: w2022 -> [w2027]
                  tunnel: w2021 -> [w2026]
                  n299 = call <vilib>:"Butterworth Filter PtByPt.vi"("initialize"=w2027, "order"=w2026, "filter type"=Filter_Passband_Type."Lowpass", "low cutoff freq: fl"=w2029, "sampling freq: fs"=w2031, "x"=w2032) -> ("Filtered x"=w2030:dbl)  [unwired: 3 in, 1 out]
                }
              }
              frame 20 {
                n300 = for {
                  tunnel: w2033 -> [w2046] mode=indexing
                  tunnel: w2038 -> [w2043]
                  tunnel: w2039 -> [w2045]
                  tunnel: [w2044] -> w2034 mode=indexing
                  tunnel: [w2043] -> w2037
                  tunnel: w2036 -> [w2041]
                  tunnel: w2035 -> [w2040]
                  n301 = call <vilib>:"Butterworth Filter PtByPt.vi"("initialize"=w2041, "order"=w2040, "filter type"=Filter_Passband_Type."Lowpass", "low cutoff freq: fl"=w2043, "sampling freq: fs"=w2045, "x"=w2046) -> ("Filtered x"=w2044:dbl)  [unwired: 3 in, 1 out]
                }
              }
              frame 21 {
                n302 = for {
                  tunnel: w2047 -> [w2060] mode=indexing
                  tunnel: w2052 -> [w2057]
                  tunnel: w2053 -> [w2059]
                  tunnel: [w2058] -> w2048 mode=indexing
                  tunnel: [w2057] -> w2051
                  tunnel: w2050 -> [w2055]
                  tunnel: w2049 -> [w2054]
                  n303 = call <vilib>:"Butterworth Filter PtByPt.vi"("initialize"=w2055, "order"=w2054, "filter type"=Filter_Passband_Type."Lowpass", "low cutoff freq: fl"=w2057, "sampling freq: fs"=w2059, "x"=w2060) -> ("Filtered x"=w2058:dbl)  [unwired: 3 in, 1 out]
                }
              }
              frame 22 {
                n304 = for {
                  tunnel: w2061 -> [w2074] mode=indexing
                  tunnel: w2066 -> [w2071]
                  tunnel: w2067 -> [w2073]
                  tunnel: [w2072] -> w2062 mode=indexing
                  tunnel: [w2071] -> w2065
                  tunnel: w2064 -> [w2069]
                  tunnel: w2063 -> [w2068]
                  n305 = call <vilib>:"Butterworth Filter PtByPt.vi"("initialize"=w2069, "order"=w2068, "filter type"=Filter_Passband_Type."Lowpass", "low cutoff freq: fl"=w2071, "sampling freq: fs"=w2073, "x"=w2074) -> ("Filtered x"=w2072:dbl)  [unwired: 3 in, 1 out]
                }
              }
              frame 23 {
                n306 = for {
                  tunnel: w2075 -> [w2088] mode=indexing
                  tunnel: w2080 -> [w2085]
                  tunnel: w2081 -> [w2087]
                  tunnel: [w2086] -> w2076 mode=indexing
                  tunnel: [w2085] -> w2079
                  tunnel: w2078 -> [w2083]
                  tunnel: w2077 -> [w2082]
                  n307 = call <vilib>:"Butterworth Filter PtByPt.vi"("initialize"=w2083, "order"=w2082, "filter type"=Filter_Passband_Type."Lowpass", "low cutoff freq: fl"=w2085, "sampling freq: fs"=w2087, "x"=w2088) -> ("Filtered x"=w2086:dbl)  [unwired: 3 in, 1 out]
                }
              }
              frame 24 {
                n308 = for {
                  tunnel: w2089 -> [w2102] mode=indexing
                  tunnel: w2094 -> [w2099]
                  tunnel: w2095 -> [w2101]
                  tunnel: [w2100] -> w2090 mode=indexing
                  tunnel: [w2099] -> w2093
                  tunnel: w2092 -> [w2097]
                  tunnel: w2091 -> [w2096]
                  n309 = call <vilib>:"Butterworth Filter PtByPt.vi"("initialize"=w2097, "order"=w2096, "filter type"=Filter_Passband_Type."Lowpass", "low cutoff freq: fl"=w2099, "sampling freq: fs"=w2101, "x"=w2102) -> ("Filtered x"=w2100:dbl)  [unwired: 3 in, 1 out]
                }
              }
              frame 25 {
                n310 = for {
                  tunnel: w2103 -> [w2116] mode=indexing
                  tunnel: w2108 -> [w2113]
                  tunnel: w2109 -> [w2115]
                  tunnel: [w2114] -> w2104 mode=indexing
                  tunnel: [w2113] -> w2107
                  tunnel: w2106 -> [w2111]
                  tunnel: w2105 -> [w2110]
                  n311 = call <vilib>:"Butterworth Filter PtByPt.vi"("initialize"=w2111, "order"=w2110, "filter type"=Filter_Passband_Type."Lowpass", "low cutoff freq: fl"=w2113, "sampling freq: fs"=w2115, "x"=w2116) -> ("Filtered x"=w2114:dbl)  [unwired: 3 in, 1 out]
                }
              }
              frame 26 {
                n312 = for {
                  tunnel: w2117 -> [w2130] mode=indexing
                  tunnel: w2122 -> [w2127]
                  tunnel: w2123 -> [w2129]
                  tunnel: [w2128] -> w2118 mode=indexing
                  tunnel: [w2127] -> w2121
                  tunnel: w2120 -> [w2125]
                  tunnel: w2119 -> [w2124]
                  n313 = call <vilib>:"Butterworth Filter PtByPt.vi"("initialize"=w2125, "order"=w2124, "filter type"=Filter_Passband_Type."Lowpass", "low cutoff freq: fl"=w2127, "sampling freq: fs"=w2129, "x"=w2130) -> ("Filtered x"=w2128:dbl)  [unwired: 3 in, 1 out]
                }
              }
              frame 27 {
                n314 = for {
                  tunnel: w2131 -> [w2144] mode=indexing
                  tunnel: w2136 -> [w2141]
                  tunnel: w2137 -> [w2143]
                  tunnel: [w2142] -> w2132 mode=indexing
                  tunnel: [w2141] -> w2135
                  tunnel: w2134 -> [w2139]
                  tunnel: w2133 -> [w2138]
                  n315 = call <vilib>:"Butterworth Filter PtByPt.vi"("initialize"=w2139, "order"=w2138, "filter type"=Filter_Passband_Type."Lowpass", "low cutoff freq: fl"=w2141, "sampling freq: fs"=w2143, "x"=w2144) -> ("Filtered x"=w2142:dbl)  [unwired: 3 in, 1 out]
                }
              }
              frame 28 {
                n316 = for {
                  tunnel: w2145 -> [w2158] mode=indexing
                  tunnel: w2150 -> [w2155]
                  tunnel: w2151 -> [w2157]
                  tunnel: [w2156] -> w2146 mode=indexing
                  tunnel: [w2155] -> w2149
                  tunnel: w2148 -> [w2153]
                  tunnel: w2147 -> [w2152]
                  n317 = call <vilib>:"Butterworth Filter PtByPt.vi"("initialize"=w2153, "order"=w2152, "filter type"=Filter_Passband_Type."Lowpass", "low cutoff freq: fl"=w2155, "sampling freq: fs"=w2157, "x"=w2158) -> ("Filtered x"=w2156:dbl)  [unwired: 3 in, 1 out]
                }
              }
              frame 29 {
                n318 = for {
                  tunnel: w2159 -> [w2172] mode=indexing
                  tunnel: w2164 -> [w2169]
                  tunnel: w2165 -> [w2171]
                  tunnel: [w2170] -> w2160 mode=indexing
                  tunnel: [w2169] -> w2163
                  tunnel: w2162 -> [w2167]
                  tunnel: w2161 -> [w2166]
                  n319 = call <vilib>:"Butterworth Filter PtByPt.vi"("initialize"=w2167, "order"=w2166, "filter type"=Filter_Passband_Type."Lowpass", "low cutoff freq: fl"=w2169, "sampling freq: fs"=w2171, "x"=w2172) -> ("Filtered x"=w2170:dbl)  [unwired: 3 in, 1 out]
                }
              }
              frame 30 {
                n320 = for {
                  tunnel: w2173 -> [w2186] mode=indexing
                  tunnel: w2178 -> [w2183]
                  tunnel: w2179 -> [w2185]
                  tunnel: [w2184] -> w2174 mode=indexing
                  tunnel: [w2183] -> w2177
                  tunnel: w2176 -> [w2181]
                  tunnel: w2175 -> [w2180]
                  n321 = call <vilib>:"Butterworth Filter PtByPt.vi"("initialize"=w2181, "order"=w2180, "filter type"=Filter_Passband_Type."Lowpass", "low cutoff freq: fl"=w2183, "sampling freq: fs"=w2185, "x"=w2186) -> ("Filtered x"=w2184:dbl)  [unwired: 3 in, 1 out]
                }
              }
              frame 31 {
                n322 = for {
                  tunnel: w2187 -> [w2200] mode=indexing
                  tunnel: w2192 -> [w2197]
                  tunnel: w2193 -> [w2199]
                  tunnel: [w2198] -> w2188 mode=indexing
                  tunnel: [w2197] -> w2191
                  tunnel: w2190 -> [w2195]
                  tunnel: w2189 -> [w2194]
                  n323 = call <vilib>:"Butterworth Filter PtByPt.vi"("initialize"=w2195, "order"=w2194, "filter type"=Filter_Passband_Type."Lowpass", "low cutoff freq: fl"=w2197, "sampling freq: fs"=w2199, "x"=w2200) -> ("Filtered x"=w2198:dbl)  [unwired: 3 in, 1 out]
                }
              }
              frame 32 {
                n324 = for {
                  tunnel: w2201 -> [w2214] mode=indexing
                  tunnel: w2206 -> [w2211]
                  tunnel: w2207 -> [w2213]
                  tunnel: [w2212] -> w2202 mode=indexing
                  tunnel: [w2211] -> w2205
                  tunnel: w2204 -> [w2209]
                  tunnel: w2203 -> [w2208]
                  n325 = call <vilib>:"Butterworth Filter PtByPt.vi"("initialize"=w2209, "order"=w2208, "filter type"=Filter_Passband_Type."Lowpass", "low cutoff freq: fl"=w2211, "sampling freq: fs"=w2213, "x"=w2214) -> ("Filtered x"=w2212:dbl)  [unwired: 3 in, 1 out]
                }
              }
              frame 33 {
                n326 = for {
                  tunnel: w2215 -> [w2228] mode=indexing
                  tunnel: w2220 -> [w2225]
                  tunnel: w2221 -> [w2227]
                  tunnel: [w2226] -> w2216 mode=indexing
                  tunnel: [w2225] -> w2219
                  tunnel: w2218 -> [w2223]
                  tunnel: w2217 -> [w2222]
                  n327 = call <vilib>:"Butterworth Filter PtByPt.vi"("initialize"=w2223, "order"=w2222, "filter type"=Filter_Passband_Type."Lowpass", "low cutoff freq: fl"=w2225, "sampling freq: fs"=w2227, "x"=w2228) -> ("Filtered x"=w2226:dbl)  [unwired: 3 in, 1 out]
                }
              }
              frame 34 {
                n328 = for {
                  tunnel: w2229 -> [w2242] mode=indexing
                  tunnel: w2234 -> [w2239]
                  tunnel: w2235 -> [w2241]
                  tunnel: [w2240] -> w2230 mode=indexing
                  tunnel: [w2239] -> w2233
                  tunnel: w2232 -> [w2237]
                  tunnel: w2231 -> [w2236]
                  n329 = call <vilib>:"Butterworth Filter PtByPt.vi"("initialize"=w2237, "order"=w2236, "filter type"=Filter_Passband_Type."Lowpass", "low cutoff freq: fl"=w2239, "sampling freq: fs"=w2241, "x"=w2242) -> ("Filtered x"=w2240:dbl)  [unwired: 3 in, 1 out]
                }
              }
              frame 35 {
                n330 = for {
                  tunnel: w2243 -> [w2256] mode=indexing
                  tunnel: w2248 -> [w2253]
                  tunnel: w2249 -> [w2255]
                  tunnel: [w2254] -> w2244 mode=indexing
                  tunnel: [w2253] -> w2247
                  tunnel: w2246 -> [w2251]
                  tunnel: w2245 -> [w2250]
                  n331 = call <vilib>:"Butterworth Filter PtByPt.vi"("initialize"=w2251, "order"=w2250, "filter type"=Filter_Passband_Type."Lowpass", "low cutoff freq: fl"=w2253, "sampling freq: fs"=w2255, "x"=w2256) -> ("Filtered x"=w2254:dbl)  [unwired: 3 in, 1 out]
                }
              }
              frame 36 {
                n332 = for {
                  tunnel: w2257 -> [w2270] mode=indexing
                  tunnel: w2262 -> [w2267]
                  tunnel: w2263 -> [w2269]
                  tunnel: [w2268] -> w2258 mode=indexing
                  tunnel: [w2267] -> w2261
                  tunnel: w2260 -> [w2265]
                  tunnel: w2259 -> [w2264]
                  n333 = call <vilib>:"Butterworth Filter PtByPt.vi"("initialize"=w2265, "order"=w2264, "filter type"=Filter_Passband_Type."Lowpass", "low cutoff freq: fl"=w2267, "sampling freq: fs"=w2269, "x"=w2270) -> ("Filtered x"=w2268:dbl)  [unwired: 3 in, 1 out]
                }
              }
              frame 37 {
                n334 = for {
                  tunnel: w2271 -> [w2284] mode=indexing
                  tunnel: w2276 -> [w2281]
                  tunnel: w2277 -> [w2283]
                  tunnel: [w2282] -> w2272 mode=indexing
                  tunnel: [w2281] -> w2275
                  tunnel: w2274 -> [w2279]
                  tunnel: w2273 -> [w2278]
                  n335 = call <vilib>:"Butterworth Filter PtByPt.vi"("initialize"=w2279, "order"=w2278, "filter type"=Filter_Passband_Type."Lowpass", "low cutoff freq: fl"=w2281, "sampling freq: fs"=w2283, "x"=w2284) -> ("Filtered x"=w2282:dbl)  [unwired: 3 in, 1 out]
                }
              }
              frame 38 {
                n336 = for {
                  tunnel: w2285 -> [w2298] mode=indexing
                  tunnel: w2290 -> [w2295]
                  tunnel: w2291 -> [w2297]
                  tunnel: [w2296] -> w2286 mode=indexing
                  tunnel: [w2295] -> w2289
                  tunnel: w2288 -> [w2293]
                  tunnel: w2287 -> [w2292]
                  n337 = call <vilib>:"Butterworth Filter PtByPt.vi"("initialize"=w2293, "order"=w2292, "filter type"=Filter_Passband_Type."Lowpass", "low cutoff freq: fl"=w2295, "sampling freq: fs"=w2297, "x"=w2298) -> ("Filtered x"=w2296:dbl)  [unwired: 3 in, 1 out]
                }
              }
              frame 39 {
                n338 = for {
                  tunnel: w2299 -> [w2312] mode=indexing
                  tunnel: w2304 -> [w2309]
                  tunnel: w2305 -> [w2311]
                  tunnel: [w2310] -> w2300 mode=indexing
                  tunnel: [w2309] -> w2303
                  tunnel: w2302 -> [w2307]
                  tunnel: w2301 -> [w2306]
                  n339 = call <vilib>:"Butterworth Filter PtByPt.vi"("initialize"=w2307, "order"=w2306, "filter type"=Filter_Passband_Type."Lowpass", "low cutoff freq: fl"=w2309, "sampling freq: fs"=w2311, "x"=w2312) -> ("Filtered x"=w2310:dbl)  [unwired: 3 in, 1 out]
                }
              }
              frame 40 {
                n340 = for {
                  tunnel: w2313 -> [w2326] mode=indexing
                  tunnel: w2318 -> [w2323]
                  tunnel: w2319 -> [w2325]
                  tunnel: [w2324] -> w2314 mode=indexing
                  tunnel: [w2323] -> w2317
                  tunnel: w2316 -> [w2321]
                  tunnel: w2315 -> [w2320]
                  n341 = call <vilib>:"Butterworth Filter PtByPt.vi"("initialize"=w2321, "order"=w2320, "filter type"=Filter_Passband_Type."Lowpass", "low cutoff freq: fl"=w2323, "sampling freq: fs"=w2325, "x"=w2326) -> ("Filtered x"=w2324:dbl)  [unwired: 3 in, 1 out]
                }
              }
              frame 41 {
                n342 = for {
                  tunnel: w2327 -> [w2340] mode=indexing
                  tunnel: w2332 -> [w2337]
                  tunnel: w2333 -> [w2339]
                  tunnel: [w2338] -> w2328 mode=indexing
                  tunnel: [w2337] -> w2331
                  tunnel: w2330 -> [w2335]
                  tunnel: w2329 -> [w2334]
                  n343 = call <vilib>:"Butterworth Filter PtByPt.vi"("initialize"=w2335, "order"=w2334, "filter type"=Filter_Passband_Type."Lowpass", "low cutoff freq: fl"=w2337, "sampling freq: fs"=w2339, "x"=w2340) -> ("Filtered x"=w2338:dbl)  [unwired: 3 in, 1 out]
                }
              }
              frame 42 {
                n344 = for {
                  tunnel: w2341 -> [w2354] mode=indexing
                  tunnel: w2346 -> [w2351]
                  tunnel: w2347 -> [w2353]
                  tunnel: [w2352] -> w2342 mode=indexing
                  tunnel: [w2351] -> w2345
                  tunnel: w2344 -> [w2349]
                  tunnel: w2343 -> [w2348]
                  n345 = call <vilib>:"Butterworth Filter PtByPt.vi"("initialize"=w2349, "order"=w2348, "filter type"=Filter_Passband_Type."Lowpass", "low cutoff freq: fl"=w2351, "sampling freq: fs"=w2353, "x"=w2354) -> ("Filtered x"=w2352:dbl)  [unwired: 3 in, 1 out]
                }
              }
              frame 43 {
                n346 = for {
                  tunnel: w2355 -> [w2368] mode=indexing
                  tunnel: w2360 -> [w2365]
                  tunnel: w2361 -> [w2367]
                  tunnel: [w2366] -> w2356 mode=indexing
                  tunnel: [w2365] -> w2359
                  tunnel: w2358 -> [w2363]
                  tunnel: w2357 -> [w2362]
                  n347 = call <vilib>:"Butterworth Filter PtByPt.vi"("initialize"=w2363, "order"=w2362, "filter type"=Filter_Passband_Type."Lowpass", "low cutoff freq: fl"=w2365, "sampling freq: fs"=w2367, "x"=w2368) -> ("Filtered x"=w2366:dbl)  [unwired: 3 in, 1 out]
                }
              }
              frame 44 {
                n348 = for {
                  tunnel: w2369 -> [w2382] mode=indexing
                  tunnel: w2374 -> [w2379]
                  tunnel: w2375 -> [w2381]
                  tunnel: [w2380] -> w2370 mode=indexing
                  tunnel: [w2379] -> w2373
                  tunnel: w2372 -> [w2377]
                  tunnel: w2371 -> [w2376]
                  n349 = call <vilib>:"Butterworth Filter PtByPt.vi"("initialize"=w2377, "order"=w2376, "filter type"=Filter_Passband_Type."Lowpass", "low cutoff freq: fl"=w2379, "sampling freq: fs"=w2381, "x"=w2382) -> ("Filtered x"=w2380:dbl)  [unwired: 3 in, 1 out]
                }
              }
              frame 45 {
                n350 = for {
                  tunnel: w2383 -> [w2396] mode=indexing
                  tunnel: w2388 -> [w2393]
                  tunnel: w2389 -> [w2395]
                  tunnel: [w2394] -> w2384 mode=indexing
                  tunnel: [w2393] -> w2387
                  tunnel: w2386 -> [w2391]
                  tunnel: w2385 -> [w2390]
                  n351 = call <vilib>:"Butterworth Filter PtByPt.vi"("initialize"=w2391, "order"=w2390, "filter type"=Filter_Passband_Type."Lowpass", "low cutoff freq: fl"=w2393, "sampling freq: fs"=w2395, "x"=w2396) -> ("Filtered x"=w2394:dbl)  [unwired: 3 in, 1 out]
                }
              }
              frame 46 {
                n352 = for {
                  tunnel: w2397 -> [w2410] mode=indexing
                  tunnel: w2402 -> [w2407]
                  tunnel: w2403 -> [w2409]
                  tunnel: [w2408] -> w2398 mode=indexing
                  tunnel: [w2407] -> w2401
                  tunnel: w2400 -> [w2405]
                  tunnel: w2399 -> [w2404]
                  n353 = call <vilib>:"Butterworth Filter PtByPt.vi"("initialize"=w2405, "order"=w2404, "filter type"=Filter_Passband_Type."Lowpass", "low cutoff freq: fl"=w2407, "sampling freq: fs"=w2409, "x"=w2410) -> ("Filtered x"=w2408:dbl)  [unwired: 3 in, 1 out]
                }
              }
              frame 47 {
                n354 = for {
                  tunnel: w2411 -> [w2424] mode=indexing
                  tunnel: w2416 -> [w2421]
                  tunnel: w2417 -> [w2423]
                  tunnel: [w2422] -> w2412 mode=indexing
                  tunnel: [w2421] -> w2415
                  tunnel: w2414 -> [w2419]
                  tunnel: w2413 -> [w2418]
                  n355 = call <vilib>:"Butterworth Filter PtByPt.vi"("initialize"=w2419, "order"=w2418, "filter type"=Filter_Passband_Type."Lowpass", "low cutoff freq: fl"=w2421, "sampling freq: fs"=w2423, "x"=w2424) -> ("Filtered x"=w2422:dbl)  [unwired: 3 in, 1 out]
                }
              }
              frame 48 {
                n356 = for {
                  tunnel: w2425 -> [w2438] mode=indexing
                  tunnel: w2430 -> [w2435]
                  tunnel: w2431 -> [w2437]
                  tunnel: [w2436] -> w2426 mode=indexing
                  tunnel: [w2435] -> w2429
                  tunnel: w2428 -> [w2433]
                  tunnel: w2427 -> [w2432]
                  n357 = call <vilib>:"Butterworth Filter PtByPt.vi"("initialize"=w2433, "order"=w2432, "filter type"=Filter_Passband_Type."Lowpass", "low cutoff freq: fl"=w2435, "sampling freq: fs"=w2437, "x"=w2438) -> ("Filtered x"=w2436:dbl)  [unwired: 3 in, 1 out]
                }
              }
              frame 49 {
                n358 = for {
                  tunnel: w2439 -> [w2452] mode=indexing
                  tunnel: w2444 -> [w2449]
                  tunnel: w2445 -> [w2451]
                  tunnel: [w2450] -> w2440 mode=indexing
                  tunnel: [w2449] -> w2443
                  tunnel: w2442 -> [w2447]
                  tunnel: w2441 -> [w2446]
                  n359 = call <vilib>:"Butterworth Filter PtByPt.vi"("initialize"=w2447, "order"=w2446, "filter type"=Filter_Passband_Type."Lowpass", "low cutoff freq: fl"=w2449, "sampling freq: fs"=w2451, "x"=w2452) -> ("Filtered x"=w2450:dbl)  [unwired: 3 in, 1 out]
                }
              }
              frame 50 {
                n360 = for {
                  tunnel: w2453 -> [w2466] mode=indexing
                  tunnel: w2458 -> [w2463]
                  tunnel: w2459 -> [w2465]
                  tunnel: [w2464] -> w2454 mode=indexing
                  tunnel: [w2463] -> w2457
                  tunnel: w2456 -> [w2461]
                  tunnel: w2455 -> [w2460]
                  n361 = call <vilib>:"Butterworth Filter PtByPt.vi"("initialize"=w2461, "order"=w2460, "filter type"=Filter_Passband_Type."Lowpass", "low cutoff freq: fl"=w2463, "sampling freq: fs"=w2465, "x"=w2466) -> ("Filtered x"=w2464:dbl)  [unwired: 3 in, 1 out]
                }
              }
              frame 51 {
                n362 = for {
                  tunnel: w2467 -> [w2480] mode=indexing
                  tunnel: w2472 -> [w2477]
                  tunnel: w2473 -> [w2479]
                  tunnel: [w2478] -> w2468 mode=indexing
                  tunnel: [w2477] -> w2471
                  tunnel: w2470 -> [w2475]
                  tunnel: w2469 -> [w2474]
                  n363 = call <vilib>:"Butterworth Filter PtByPt.vi"("initialize"=w2475, "order"=w2474, "filter type"=Filter_Passband_Type."Lowpass", "low cutoff freq: fl"=w2477, "sampling freq: fs"=w2479, "x"=w2480) -> ("Filtered x"=w2478:dbl)  [unwired: 3 in, 1 out]
                }
              }
              frame 52 {
                n364 = for {
                  tunnel: w2481 -> [w2494] mode=indexing
                  tunnel: w2486 -> [w2491]
                  tunnel: w2487 -> [w2493]
                  tunnel: [w2492] -> w2482 mode=indexing
                  tunnel: [w2491] -> w2485
                  tunnel: w2484 -> [w2489]
                  tunnel: w2483 -> [w2488]
                  n365 = call <vilib>:"Butterworth Filter PtByPt.vi"("initialize"=w2489, "order"=w2488, "filter type"=Filter_Passband_Type."Lowpass", "low cutoff freq: fl"=w2491, "sampling freq: fs"=w2493, "x"=w2494) -> ("Filtered x"=w2492:dbl)  [unwired: 3 in, 1 out]
                }
              }
              frame 53 {
                n366 = for {
                  tunnel: w2495 -> [w2508] mode=indexing
                  tunnel: w2500 -> [w2505]
                  tunnel: w2501 -> [w2507]
                  tunnel: [w2506] -> w2496 mode=indexing
                  tunnel: [w2505] -> w2499
                  tunnel: w2498 -> [w2503]
                  tunnel: w2497 -> [w2502]
                  n367 = call <vilib>:"Butterworth Filter PtByPt.vi"("initialize"=w2503, "order"=w2502, "filter type"=Filter_Passband_Type."Lowpass", "low cutoff freq: fl"=w2505, "sampling freq: fs"=w2507, "x"=w2508) -> ("Filtered x"=w2506:dbl)  [unwired: 3 in, 1 out]
                }
              }
              frame 54 {
                n368 = for {
                  tunnel: w2509 -> [w2522] mode=indexing
                  tunnel: w2514 -> [w2519]
                  tunnel: w2515 -> [w2521]
                  tunnel: [w2520] -> w2510 mode=indexing
                  tunnel: [w2519] -> w2513
                  tunnel: w2512 -> [w2517]
                  tunnel: w2511 -> [w2516]
                  n369 = call <vilib>:"Butterworth Filter PtByPt.vi"("initialize"=w2517, "order"=w2516, "filter type"=Filter_Passband_Type."Lowpass", "low cutoff freq: fl"=w2519, "sampling freq: fs"=w2521, "x"=w2522) -> ("Filtered x"=w2520:dbl)  [unwired: 3 in, 1 out]
                }
              }
              frame 55 {
                n370 = for {
                  tunnel: w2523 -> [w2536] mode=indexing
                  tunnel: w2528 -> [w2533]
                  tunnel: w2529 -> [w2535]
                  tunnel: [w2534] -> w2524 mode=indexing
                  tunnel: [w2533] -> w2527
                  tunnel: w2526 -> [w2531]
                  tunnel: w2525 -> [w2530]
                  n371 = call <vilib>:"Butterworth Filter PtByPt.vi"("initialize"=w2531, "order"=w2530, "filter type"=Filter_Passband_Type."Lowpass", "low cutoff freq: fl"=w2533, "sampling freq: fs"=w2535, "x"=w2536) -> ("Filtered x"=w2534:dbl)  [unwired: 3 in, 1 out]
                }
              }
              frame 56 {
                n372 = for {
                  tunnel: w2537 -> [w2550] mode=indexing
                  tunnel: w2542 -> [w2547]
                  tunnel: w2543 -> [w2549]
                  tunnel: [w2548] -> w2538 mode=indexing
                  tunnel: [w2547] -> w2541
                  tunnel: w2540 -> [w2545]
                  tunnel: w2539 -> [w2544]
                  n373 = call <vilib>:"Butterworth Filter PtByPt.vi"("initialize"=w2545, "order"=w2544, "filter type"=Filter_Passband_Type."Lowpass", "low cutoff freq: fl"=w2547, "sampling freq: fs"=w2549, "x"=w2550) -> ("Filtered x"=w2548:dbl)  [unwired: 3 in, 1 out]
                }
              }
              frame 57 {
                n374 = for {
                  tunnel: w2551 -> [w2564] mode=indexing
                  tunnel: w2556 -> [w2561]
                  tunnel: w2557 -> [w2563]
                  tunnel: [w2562] -> w2552 mode=indexing
                  tunnel: [w2561] -> w2555
                  tunnel: w2554 -> [w2559]
                  tunnel: w2553 -> [w2558]
                  n375 = call <vilib>:"Butterworth Filter PtByPt.vi"("initialize"=w2559, "order"=w2558, "filter type"=Filter_Passband_Type."Lowpass", "low cutoff freq: fl"=w2561, "sampling freq: fs"=w2563, "x"=w2564) -> ("Filtered x"=w2562:dbl)  [unwired: 3 in, 1 out]
                }
              }
              frame 58 {
                n376 = for {
                  tunnel: w2565 -> [w2578] mode=indexing
                  tunnel: w2570 -> [w2575]
                  tunnel: w2571 -> [w2577]
                  tunnel: [w2576] -> w2566 mode=indexing
                  tunnel: [w2575] -> w2569
                  tunnel: w2568 -> [w2573]
                  tunnel: w2567 -> [w2572]
                  n377 = call <vilib>:"Butterworth Filter PtByPt.vi"("initialize"=w2573, "order"=w2572, "filter type"=Filter_Passband_Type."Lowpass", "low cutoff freq: fl"=w2575, "sampling freq: fs"=w2577, "x"=w2578) -> ("Filtered x"=w2576:dbl)  [unwired: 3 in, 1 out]
                }
              }
              frame 59 {
                n378 = for {
                  tunnel: w2579 -> [w2592] mode=indexing
                  tunnel: w2584 -> [w2589]
                  tunnel: w2585 -> [w2591]
                  tunnel: [w2590] -> w2580 mode=indexing
                  tunnel: [w2589] -> w2583
                  tunnel: w2582 -> [w2587]
                  tunnel: w2581 -> [w2586]
                  n379 = call <vilib>:"Butterworth Filter PtByPt.vi"("initialize"=w2587, "order"=w2586, "filter type"=Filter_Passband_Type."Lowpass", "low cutoff freq: fl"=w2589, "sampling freq: fs"=w2591, "x"=w2592) -> ("Filtered x"=w2590:dbl)  [unwired: 3 in, 1 out]
                }
              }
              frame 60 {
                n380 = for {
                  tunnel: w2593 -> [w2606] mode=indexing
                  tunnel: w2598 -> [w2603]
                  tunnel: w2599 -> [w2605]
                  tunnel: [w2604] -> w2594 mode=indexing
                  tunnel: [w2603] -> w2597
                  tunnel: w2596 -> [w2601]
                  tunnel: w2595 -> [w2600]
                  n381 = call <vilib>:"Butterworth Filter PtByPt.vi"("initialize"=w2601, "order"=w2600, "filter type"=Filter_Passband_Type."Lowpass", "low cutoff freq: fl"=w2603, "sampling freq: fs"=w2605, "x"=w2606) -> ("Filtered x"=w2604:dbl)  [unwired: 3 in, 1 out]
                }
              }
              frame 61 {
                n382 = for {
                  tunnel: w2607 -> [w2620] mode=indexing
                  tunnel: w2612 -> [w2617]
                  tunnel: w2613 -> [w2619]
                  tunnel: [w2618] -> w2608 mode=indexing
                  tunnel: [w2617] -> w2611
                  tunnel: w2610 -> [w2615]
                  tunnel: w2609 -> [w2614]
                  n383 = call <vilib>:"Butterworth Filter PtByPt.vi"("initialize"=w2615, "order"=w2614, "filter type"=Filter_Passband_Type."Lowpass", "low cutoff freq: fl"=w2617, "sampling freq: fs"=w2619, "x"=w2620) -> ("Filtered x"=w2618:dbl)  [unwired: 3 in, 1 out]
                }
              }
              frame 62 {
                n384 = for {
                  tunnel: w2621 -> [w2634] mode=indexing
                  tunnel: w2626 -> [w2631]
                  tunnel: w2627 -> [w2633]
                  tunnel: [w2632] -> w2622 mode=indexing
                  tunnel: [w2631] -> w2625
                  tunnel: w2624 -> [w2629]
                  tunnel: w2623 -> [w2628]
                  n385 = call <vilib>:"Butterworth Filter PtByPt.vi"("initialize"=w2629, "order"=w2628, "filter type"=Filter_Passband_Type."Lowpass", "low cutoff freq: fl"=w2631, "sampling freq: fs"=w2633, "x"=w2634) -> ("Filtered x"=w2632:dbl)  [unwired: 3 in, 1 out]
                }
              }
              frame 63 {
                n386 = for {
                  tunnel: w2635 -> [w2648] mode=indexing
                  tunnel: w2640 -> [w2645]
                  tunnel: w2641 -> [w2647]
                  tunnel: [w2646] -> w2636 mode=indexing
                  tunnel: [w2645] -> w2639
                  tunnel: w2638 -> [w2643]
                  tunnel: w2637 -> [w2642]
                  n387 = call <vilib>:"Butterworth Filter PtByPt.vi"("initialize"=w2643, "order"=w2642, "filter type"=Filter_Passband_Type."Lowpass", "low cutoff freq: fl"=w2645, "sampling freq: fs"=w2647, "x"=w2648) -> ("Filtered x"=w2646:dbl)  [unwired: 3 in, 1 out]
                }
              }
              frame 64 {
                n388 = for {
                  tunnel: w2649 -> [w2662] mode=indexing
                  tunnel: w2654 -> [w2659]
                  tunnel: w2655 -> [w2661]
                  tunnel: [w2660] -> w2650 mode=indexing
                  tunnel: [w2659] -> w2653
                  tunnel: w2652 -> [w2657]
                  tunnel: w2651 -> [w2656]
                  n389 = call <vilib>:"Butterworth Filter PtByPt.vi"("initialize"=w2657, "order"=w2656, "filter type"=Filter_Passband_Type."Lowpass", "low cutoff freq: fl"=w2659, "sampling freq: fs"=w2661, "x"=w2662) -> ("Filtered x"=w2660:dbl)  [unwired: 3 in, 1 out]
                }
              }
              frame 65 {
                n390 = for {
                  tunnel: w2663 -> [w2676] mode=indexing
                  tunnel: w2668 -> [w2673]
                  tunnel: w2669 -> [w2675]
                  tunnel: [w2674] -> w2664 mode=indexing
                  tunnel: [w2673] -> w2667
                  tunnel: w2666 -> [w2671]
                  tunnel: w2665 -> [w2670]
                  n391 = call <vilib>:"Butterworth Filter PtByPt.vi"("initialize"=w2671, "order"=w2670, "filter type"=Filter_Passband_Type."Lowpass", "low cutoff freq: fl"=w2673, "sampling freq: fs"=w2675, "x"=w2676) -> ("Filtered x"=w2674:dbl)  [unwired: 3 in, 1 out]
                }
              }
              frame 66 {
                n392 = for {
                  tunnel: w2677 -> [w2690] mode=indexing
                  tunnel: w2682 -> [w2687]
                  tunnel: w2683 -> [w2689]
                  tunnel: [w2688] -> w2678 mode=indexing
                  tunnel: [w2687] -> w2681
                  tunnel: w2680 -> [w2685]
                  tunnel: w2679 -> [w2684]
                  n393 = call <vilib>:"Butterworth Filter PtByPt.vi"("initialize"=w2685, "order"=w2684, "filter type"=Filter_Passband_Type."Lowpass", "low cutoff freq: fl"=w2687, "sampling freq: fs"=w2689, "x"=w2690) -> ("Filtered x"=w2688:dbl)  [unwired: 3 in, 1 out]
                }
              }
              frame 67 {
                n394 = for {
                  tunnel: w2691 -> [w2704] mode=indexing
                  tunnel: w2696 -> [w2701]
                  tunnel: w2697 -> [w2703]
                  tunnel: [w2702] -> w2692 mode=indexing
                  tunnel: [w2701] -> w2695
                  tunnel: w2694 -> [w2699]
                  tunnel: w2693 -> [w2698]
                  n395 = call <vilib>:"Butterworth Filter PtByPt.vi"("initialize"=w2699, "order"=w2698, "filter type"=Filter_Passband_Type."Lowpass", "low cutoff freq: fl"=w2701, "sampling freq: fs"=w2703, "x"=w2704) -> ("Filtered x"=w2702:dbl)  [unwired: 3 in, 1 out]
                }
              }
              frame 68 {
                n396 = for {
                  tunnel: w2705 -> [w2718] mode=indexing
                  tunnel: w2710 -> [w2715]
                  tunnel: w2711 -> [w2717]
                  tunnel: [w2716] -> w2706 mode=indexing
                  tunnel: [w2715] -> w2709
                  tunnel: w2708 -> [w2713]
                  tunnel: w2707 -> [w2712]
                  n397 = call <vilib>:"Butterworth Filter PtByPt.vi"("initialize"=w2713, "order"=w2712, "filter type"=Filter_Passband_Type."Lowpass", "low cutoff freq: fl"=w2715, "sampling freq: fs"=w2717, "x"=w2718) -> ("Filtered x"=w2716:dbl)  [unwired: 3 in, 1 out]
                }
              }
              frame 69 {
                n398 = for {
                  tunnel: w2719 -> [w2732] mode=indexing
                  tunnel: w2724 -> [w2729]
                  tunnel: w2725 -> [w2731]
                  tunnel: [w2730] -> w2720 mode=indexing
                  tunnel: [w2729] -> w2723
                  tunnel: w2722 -> [w2727]
                  tunnel: w2721 -> [w2726]
                  n399 = call <vilib>:"Butterworth Filter PtByPt.vi"("initialize"=w2727, "order"=w2726, "filter type"=Filter_Passband_Type."Lowpass", "low cutoff freq: fl"=w2729, "sampling freq: fs"=w2731, "x"=w2732) -> ("Filtered x"=w2730:dbl)  [unwired: 3 in, 1 out]
                }
              }
              frame 70 {
                n400 = for {
                  tunnel: w2733 -> [w2746] mode=indexing
                  tunnel: w2738 -> [w2743]
                  tunnel: w2739 -> [w2745]
                  tunnel: [w2744] -> w2734 mode=indexing
                  tunnel: [w2743] -> w2737
                  tunnel: w2736 -> [w2741]
                  tunnel: w2735 -> [w2740]
                  n401 = call <vilib>:"Butterworth Filter PtByPt.vi"("initialize"=w2741, "order"=w2740, "filter type"=Filter_Passband_Type."Lowpass", "low cutoff freq: fl"=w2743, "sampling freq: fs"=w2745, "x"=w2746) -> ("Filtered x"=w2744:dbl)  [unwired: 3 in, 1 out]
                }
              }
              frame 71 {
                n402 = for {
                  tunnel: w2747 -> [w2760] mode=indexing
                  tunnel: w2752 -> [w2757]
                  tunnel: w2753 -> [w2759]
                  tunnel: [w2758] -> w2748 mode=indexing
                  tunnel: [w2757] -> w2751
                  tunnel: w2750 -> [w2755]
                  tunnel: w2749 -> [w2754]
                  n403 = call <vilib>:"Butterworth Filter PtByPt.vi"("initialize"=w2755, "order"=w2754, "filter type"=Filter_Passband_Type."Lowpass", "low cutoff freq: fl"=w2757, "sampling freq: fs"=w2759, "x"=w2760) -> ("Filtered x"=w2758:dbl)  [unwired: 3 in, 1 out]
                }
              }
              frame 72 {
                n404 = for {
                  tunnel: w2761 -> [w2774] mode=indexing
                  tunnel: w2766 -> [w2771]
                  tunnel: w2767 -> [w2773]
                  tunnel: [w2772] -> w2762 mode=indexing
                  tunnel: [w2771] -> w2765
                  tunnel: w2764 -> [w2769]
                  tunnel: w2763 -> [w2768]
                  n405 = call <vilib>:"Butterworth Filter PtByPt.vi"("initialize"=w2769, "order"=w2768, "filter type"=Filter_Passband_Type."Lowpass", "low cutoff freq: fl"=w2771, "sampling freq: fs"=w2773, "x"=w2774) -> ("Filtered x"=w2772:dbl)  [unwired: 3 in, 1 out]
                }
              }
              frame 73 {
                n406 = for {
                  tunnel: w2775 -> [w2788] mode=indexing
                  tunnel: w2780 -> [w2785]
                  tunnel: w2781 -> [w2787]
                  tunnel: [w2786] -> w2776 mode=indexing
                  tunnel: [w2785] -> w2779
                  tunnel: w2778 -> [w2783]
                  tunnel: w2777 -> [w2782]
                  n407 = call <vilib>:"Butterworth Filter PtByPt.vi"("initialize"=w2783, "order"=w2782, "filter type"=Filter_Passband_Type."Lowpass", "low cutoff freq: fl"=w2785, "sampling freq: fs"=w2787, "x"=w2788) -> ("Filtered x"=w2786:dbl)  [unwired: 3 in, 1 out]
                }
              }
              frame 74 {
                n408 = for {
                  tunnel: w2789 -> [w2802] mode=indexing
                  tunnel: w2794 -> [w2799]
                  tunnel: w2795 -> [w2801]
                  tunnel: [w2800] -> w2790 mode=indexing
                  tunnel: [w2799] -> w2793
                  tunnel: w2792 -> [w2797]
                  tunnel: w2791 -> [w2796]
                  n409 = call <vilib>:"Butterworth Filter PtByPt.vi"("initialize"=w2797, "order"=w2796, "filter type"=Filter_Passband_Type."Lowpass", "low cutoff freq: fl"=w2799, "sampling freq: fs"=w2801, "x"=w2802) -> ("Filtered x"=w2800:dbl)  [unwired: 3 in, 1 out]
                }
              }
              frame 75 {
                n410 = for {
                  tunnel: w2803 -> [w2816] mode=indexing
                  tunnel: w2808 -> [w2813]
                  tunnel: w2809 -> [w2815]
                  tunnel: [w2814] -> w2804 mode=indexing
                  tunnel: [w2813] -> w2807
                  tunnel: w2806 -> [w2811]
                  tunnel: w2805 -> [w2810]
                  n411 = call <vilib>:"Butterworth Filter PtByPt.vi"("initialize"=w2811, "order"=w2810, "filter type"=Filter_Passband_Type."Lowpass", "low cutoff freq: fl"=w2813, "sampling freq: fs"=w2815, "x"=w2816) -> ("Filtered x"=w2814:dbl)  [unwired: 3 in, 1 out]
                }
              }
              frame 76 {
                n412 = for {
                  tunnel: w2817 -> [w2830] mode=indexing
                  tunnel: w2822 -> [w2827]
                  tunnel: w2823 -> [w2829]
                  tunnel: [w2828] -> w2818 mode=indexing
                  tunnel: [w2827] -> w2821
                  tunnel: w2820 -> [w2825]
                  tunnel: w2819 -> [w2824]
                  n413 = call <vilib>:"Butterworth Filter PtByPt.vi"("initialize"=w2825, "order"=w2824, "filter type"=Filter_Passband_Type."Lowpass", "low cutoff freq: fl"=w2827, "sampling freq: fs"=w2829, "x"=w2830) -> ("Filtered x"=w2828:dbl)  [unwired: 3 in, 1 out]
                }
              }
              frame 77 {
                n414 = for {
                  tunnel: w2831 -> [w2844] mode=indexing
                  tunnel: w2836 -> [w2841]
                  tunnel: w2837 -> [w2843]
                  tunnel: [w2842] -> w2832 mode=indexing
                  tunnel: [w2841] -> w2835
                  tunnel: w2834 -> [w2839]
                  tunnel: w2833 -> [w2838]
                  n415 = call <vilib>:"Butterworth Filter PtByPt.vi"("initialize"=w2839, "order"=w2838, "filter type"=Filter_Passband_Type."Lowpass", "low cutoff freq: fl"=w2841, "sampling freq: fs"=w2843, "x"=w2844) -> ("Filtered x"=w2842:dbl)  [unwired: 3 in, 1 out]
                }
              }
              frame 78 {
                n416 = for {
                  tunnel: w2845 -> [w2858] mode=indexing
                  tunnel: w2850 -> [w2855]
                  tunnel: w2851 -> [w2857]
                  tunnel: [w2856] -> w2846 mode=indexing
                  tunnel: [w2855] -> w2849
                  tunnel: w2848 -> [w2853]
                  tunnel: w2847 -> [w2852]
                  n417 = call <vilib>:"Butterworth Filter PtByPt.vi"("initialize"=w2853, "order"=w2852, "filter type"=Filter_Passband_Type."Lowpass", "low cutoff freq: fl"=w2855, "sampling freq: fs"=w2857, "x"=w2858) -> ("Filtered x"=w2856:dbl)  [unwired: 3 in, 1 out]
                }
              }
              frame 79 {
                n418 = for {
                  tunnel: w2859 -> [w2872] mode=indexing
                  tunnel: w2864 -> [w2869]
                  tunnel: w2865 -> [w2871]
                  tunnel: [w2870] -> w2860 mode=indexing
                  tunnel: [w2869] -> w2863
                  tunnel: w2862 -> [w2867]
                  tunnel: w2861 -> [w2866]
                  n419 = call <vilib>:"Butterworth Filter PtByPt.vi"("initialize"=w2867, "order"=w2866, "filter type"=Filter_Passband_Type."Lowpass", "low cutoff freq: fl"=w2869, "sampling freq: fs"=w2871, "x"=w2872) -> ("Filtered x"=w2870:dbl)  [unwired: 3 in, 1 out]
                }
              }
              frame 80 {
                n420 = for {
                  tunnel: w2873 -> [w2886] mode=indexing
                  tunnel: w2878 -> [w2883]
                  tunnel: w2879 -> [w2885]
                  tunnel: [w2884] -> w2874 mode=indexing
                  tunnel: [w2883] -> w2877
                  tunnel: w2876 -> [w2881]
                  tunnel: w2875 -> [w2880]
                  n421 = call <vilib>:"Butterworth Filter PtByPt.vi"("initialize"=w2881, "order"=w2880, "filter type"=Filter_Passband_Type."Lowpass", "low cutoff freq: fl"=w2883, "sampling freq: fs"=w2885, "x"=w2886) -> ("Filtered x"=w2884:dbl)  [unwired: 3 in, 1 out]
                }
              }
              frame 81 {
                n422 = for {
                  tunnel: w2887 -> [w2900] mode=indexing
                  tunnel: w2892 -> [w2897]
                  tunnel: w2893 -> [w2899]
                  tunnel: [w2898] -> w2888 mode=indexing
                  tunnel: [w2897] -> w2891
                  tunnel: w2890 -> [w2895]
                  tunnel: w2889 -> [w2894]
                  n423 = call <vilib>:"Butterworth Filter PtByPt.vi"("initialize"=w2895, "order"=w2894, "filter type"=Filter_Passband_Type."Lowpass", "low cutoff freq: fl"=w2897, "sampling freq: fs"=w2899, "x"=w2900) -> ("Filtered x"=w2898:dbl)  [unwired: 3 in, 1 out]
                }
              }
              frame 82 {
                n424 = for {
                  tunnel: w2901 -> [w2914] mode=indexing
                  tunnel: w2906 -> [w2911]
                  tunnel: w2907 -> [w2913]
                  tunnel: [w2912] -> w2902 mode=indexing
                  tunnel: [w2911] -> w2905
                  tunnel: w2904 -> [w2909]
                  tunnel: w2903 -> [w2908]
                  n425 = call <vilib>:"Butterworth Filter PtByPt.vi"("initialize"=w2909, "order"=w2908, "filter type"=Filter_Passband_Type."Lowpass", "low cutoff freq: fl"=w2911, "sampling freq: fs"=w2913, "x"=w2914) -> ("Filtered x"=w2912:dbl)  [unwired: 3 in, 1 out]
                }
              }
              frame 83 {
                n426 = for {
                  tunnel: w2915 -> [w2928] mode=indexing
                  tunnel: w2920 -> [w2925]
                  tunnel: w2921 -> [w2927]
                  tunnel: [w2926] -> w2916 mode=indexing
                  tunnel: [w2925] -> w2919
                  tunnel: w2918 -> [w2923]
                  tunnel: w2917 -> [w2922]
                  n427 = call <vilib>:"Butterworth Filter PtByPt.vi"("initialize"=w2923, "order"=w2922, "filter type"=Filter_Passband_Type."Lowpass", "low cutoff freq: fl"=w2925, "sampling freq: fs"=w2927, "x"=w2928) -> ("Filtered x"=w2926:dbl)  [unwired: 3 in, 1 out]
                }
              }
              frame 84 {
                n428 = for {
                  tunnel: w2929 -> [w2942] mode=indexing
                  tunnel: w2934 -> [w2939]
                  tunnel: w2935 -> [w2941]
                  tunnel: [w2940] -> w2930 mode=indexing
                  tunnel: [w2939] -> w2933
                  tunnel: w2932 -> [w2937]
                  tunnel: w2931 -> [w2936]
                  n429 = call <vilib>:"Butterworth Filter PtByPt.vi"("initialize"=w2937, "order"=w2936, "filter type"=Filter_Passband_Type."Lowpass", "low cutoff freq: fl"=w2939, "sampling freq: fs"=w2941, "x"=w2942) -> ("Filtered x"=w2940:dbl)  [unwired: 3 in, 1 out]
                }
              }
              frame 85 {
                n430 = for {
                  tunnel: w2943 -> [w2956] mode=indexing
                  tunnel: w2948 -> [w2953]
                  tunnel: w2949 -> [w2955]
                  tunnel: [w2954] -> w2944 mode=indexing
                  tunnel: [w2953] -> w2947
                  tunnel: w2946 -> [w2951]
                  tunnel: w2945 -> [w2950]
                  n431 = call <vilib>:"Butterworth Filter PtByPt.vi"("initialize"=w2951, "order"=w2950, "filter type"=Filter_Passband_Type."Lowpass", "low cutoff freq: fl"=w2953, "sampling freq: fs"=w2955, "x"=w2956) -> ("Filtered x"=w2954:dbl)  [unwired: 3 in, 1 out]
                }
              }
              frame 86 {
                n432 = for {
                  tunnel: w2957 -> [w2970] mode=indexing
                  tunnel: w2962 -> [w2967]
                  tunnel: w2963 -> [w2969]
                  tunnel: [w2968] -> w2958 mode=indexing
                  tunnel: [w2967] -> w2961
                  tunnel: w2960 -> [w2965]
                  tunnel: w2959 -> [w2964]
                  n433 = call <vilib>:"Butterworth Filter PtByPt.vi"("initialize"=w2965, "order"=w2964, "filter type"=Filter_Passband_Type."Lowpass", "low cutoff freq: fl"=w2967, "sampling freq: fs"=w2969, "x"=w2970) -> ("Filtered x"=w2968:dbl)  [unwired: 3 in, 1 out]
                }
              }
              frame 87 {
                n434 = for {
                  tunnel: w2971 -> [w2984] mode=indexing
                  tunnel: w2976 -> [w2981]
                  tunnel: w2977 -> [w2983]
                  tunnel: [w2982] -> w2972 mode=indexing
                  tunnel: [w2981] -> w2975
                  tunnel: w2974 -> [w2979]
                  tunnel: w2973 -> [w2978]
                  n435 = call <vilib>:"Butterworth Filter PtByPt.vi"("initialize"=w2979, "order"=w2978, "filter type"=Filter_Passband_Type."Lowpass", "low cutoff freq: fl"=w2981, "sampling freq: fs"=w2983, "x"=w2984) -> ("Filtered x"=w2982:dbl)  [unwired: 3 in, 1 out]
                }
              }
              frame 88 {
                n436 = for {
                  tunnel: w2985 -> [w2998] mode=indexing
                  tunnel: w2990 -> [w2995]
                  tunnel: w2991 -> [w2997]
                  tunnel: [w2996] -> w2986 mode=indexing
                  tunnel: [w2995] -> w2989
                  tunnel: w2988 -> [w2993]
                  tunnel: w2987 -> [w2992]
                  n437 = call <vilib>:"Butterworth Filter PtByPt.vi"("initialize"=w2993, "order"=w2992, "filter type"=Filter_Passband_Type."Lowpass", "low cutoff freq: fl"=w2995, "sampling freq: fs"=w2997, "x"=w2998) -> ("Filtered x"=w2996:dbl)  [unwired: 3 in, 1 out]
                }
              }
              frame 89 {
                n438 = for {
                  tunnel: w2999 -> [w3012] mode=indexing
                  tunnel: w3004 -> [w3009]
                  tunnel: w3005 -> [w3011]
                  tunnel: [w3010] -> w3000 mode=indexing
                  tunnel: [w3009] -> w3003
                  tunnel: w3002 -> [w3007]
                  tunnel: w3001 -> [w3006]
                  n439 = call <vilib>:"Butterworth Filter PtByPt.vi"("initialize"=w3007, "order"=w3006, "filter type"=Filter_Passband_Type."Lowpass", "low cutoff freq: fl"=w3009, "sampling freq: fs"=w3011, "x"=w3012) -> ("Filtered x"=w3010:dbl)  [unwired: 3 in, 1 out]
                }
              }
              frame 90 {
                n440 = for {
                  tunnel: w3013 -> [w3026] mode=indexing
                  tunnel: w3018 -> [w3023]
                  tunnel: w3019 -> [w3025]
                  tunnel: [w3024] -> w3014 mode=indexing
                  tunnel: [w3023] -> w3017
                  tunnel: w3016 -> [w3021]
                  tunnel: w3015 -> [w3020]
                  n441 = call <vilib>:"Butterworth Filter PtByPt.vi"("initialize"=w3021, "order"=w3020, "filter type"=Filter_Passband_Type."Lowpass", "low cutoff freq: fl"=w3023, "sampling freq: fs"=w3025, "x"=w3026) -> ("Filtered x"=w3024:dbl)  [unwired: 3 in, 1 out]
                }
              }
              frame 91 {
                n442 = for {
                  tunnel: w3027 -> [w3040] mode=indexing
                  tunnel: w3032 -> [w3037]
                  tunnel: w3033 -> [w3039]
                  tunnel: [w3038] -> w3028 mode=indexing
                  tunnel: [w3037] -> w3031
                  tunnel: w3030 -> [w3035]
                  tunnel: w3029 -> [w3034]
                  n443 = call <vilib>:"Butterworth Filter PtByPt.vi"("initialize"=w3035, "order"=w3034, "filter type"=Filter_Passband_Type."Lowpass", "low cutoff freq: fl"=w3037, "sampling freq: fs"=w3039, "x"=w3040) -> ("Filtered x"=w3038:dbl)  [unwired: 3 in, 1 out]
                }
              }
              frame 92 {
                n444 = for {
                  tunnel: w3041 -> [w3054] mode=indexing
                  tunnel: w3046 -> [w3051]
                  tunnel: w3047 -> [w3053]
                  tunnel: [w3052] -> w3042 mode=indexing
                  tunnel: [w3051] -> w3045
                  tunnel: w3044 -> [w3049]
                  tunnel: w3043 -> [w3048]
                  n445 = call <vilib>:"Butterworth Filter PtByPt.vi"("initialize"=w3049, "order"=w3048, "filter type"=Filter_Passband_Type."Lowpass", "low cutoff freq: fl"=w3051, "sampling freq: fs"=w3053, "x"=w3054) -> ("Filtered x"=w3052:dbl)  [unwired: 3 in, 1 out]
                }
              }
              frame 93 {
                n446 = for {
                  tunnel: w3055 -> [w3068] mode=indexing
                  tunnel: w3060 -> [w3065]
                  tunnel: w3061 -> [w3067]
                  tunnel: [w3066] -> w3056 mode=indexing
                  tunnel: [w3065] -> w3059
                  tunnel: w3058 -> [w3063]
                  tunnel: w3057 -> [w3062]
                  n447 = call <vilib>:"Butterworth Filter PtByPt.vi"("initialize"=w3063, "order"=w3062, "filter type"=Filter_Passband_Type."Lowpass", "low cutoff freq: fl"=w3065, "sampling freq: fs"=w3067, "x"=w3068) -> ("Filtered x"=w3066:dbl)  [unwired: 3 in, 1 out]
                }
              }
              frame 94 {
                n448 = for {
                  tunnel: w3069 -> [w3082] mode=indexing
                  tunnel: w3074 -> [w3079]
                  tunnel: w3075 -> [w3081]
                  tunnel: [w3080] -> w3070 mode=indexing
                  tunnel: [w3079] -> w3073
                  tunnel: w3072 -> [w3077]
                  tunnel: w3071 -> [w3076]
                  n449 = call <vilib>:"Butterworth Filter PtByPt.vi"("initialize"=w3077, "order"=w3076, "filter type"=Filter_Passband_Type."Lowpass", "low cutoff freq: fl"=w3079, "sampling freq: fs"=w3081, "x"=w3082) -> ("Filtered x"=w3080:dbl)  [unwired: 3 in, 1 out]
                }
              }
              frame 95 {
                n450 = for {
                  tunnel: w3083 -> [w3096] mode=indexing
                  tunnel: w3088 -> [w3093]
                  tunnel: w3089 -> [w3095]
                  tunnel: [w3094] -> w3084 mode=indexing
                  tunnel: [w3093] -> w3087
                  tunnel: w3086 -> [w3091]
                  tunnel: w3085 -> [w3090]
                  n451 = call <vilib>:"Butterworth Filter PtByPt.vi"("initialize"=w3091, "order"=w3090, "filter type"=Filter_Passband_Type."Lowpass", "low cutoff freq: fl"=w3093, "sampling freq: fs"=w3095, "x"=w3096) -> ("Filtered x"=w3094:dbl)  [unwired: 3 in, 1 out]
                }
              }
              frame 96 {
                n452 = for {
                  tunnel: w3097 -> [w3110] mode=indexing
                  tunnel: w3102 -> [w3107]
                  tunnel: w3103 -> [w3109]
                  tunnel: [w3108] -> w3098 mode=indexing
                  tunnel: [w3107] -> w3101
                  tunnel: w3100 -> [w3105]
                  tunnel: w3099 -> [w3104]
                  n453 = call <vilib>:"Butterworth Filter PtByPt.vi"("initialize"=w3105, "order"=w3104, "filter type"=Filter_Passband_Type."Lowpass", "low cutoff freq: fl"=w3107, "sampling freq: fs"=w3109, "x"=w3110) -> ("Filtered x"=w3108:dbl)  [unwired: 3 in, 1 out]
                }
              }
              frame 97 {
                n454 = for {
                  tunnel: w3111 -> [w3124] mode=indexing
                  tunnel: w3116 -> [w3121]
                  tunnel: w3117 -> [w3123]
                  tunnel: [w3122] -> w3112 mode=indexing
                  tunnel: [w3121] -> w3115
                  tunnel: w3114 -> [w3119]
                  tunnel: w3113 -> [w3118]
                  n455 = call <vilib>:"Butterworth Filter PtByPt.vi"("initialize"=w3119, "order"=w3118, "filter type"=Filter_Passband_Type."Lowpass", "low cutoff freq: fl"=w3121, "sampling freq: fs"=w3123, "x"=w3124) -> ("Filtered x"=w3122:dbl)  [unwired: 3 in, 1 out]
                }
              }
              frame 98 {
                n456 = for {
                  tunnel: w3125 -> [w3138] mode=indexing
                  tunnel: w3130 -> [w3135]
                  tunnel: w3131 -> [w3137]
                  tunnel: [w3136] -> w3126 mode=indexing
                  tunnel: [w3135] -> w3129
                  tunnel: w3128 -> [w3133]
                  tunnel: w3127 -> [w3132]
                  n457 = call <vilib>:"Butterworth Filter PtByPt.vi"("initialize"=w3133, "order"=w3132, "filter type"=Filter_Passband_Type."Lowpass", "low cutoff freq: fl"=w3135, "sampling freq: fs"=w3137, "x"=w3138) -> ("Filtered x"=w3136:dbl)  [unwired: 3 in, 1 out]
                }
              }
              frame 99 {
                n458 = for {
                  tunnel: w3139 -> [w3152] mode=indexing
                  tunnel: w3144 -> [w3149]
                  tunnel: w3145 -> [w3151]
                  tunnel: [w3150] -> w3140 mode=indexing
                  tunnel: [w3149] -> w3143
                  tunnel: w3142 -> [w3147]
                  tunnel: w3141 -> [w3146]
                  n459 = call <vilib>:"Butterworth Filter PtByPt.vi"("initialize"=w3147, "order"=w3146, "filter type"=Filter_Passband_Type."Lowpass", "low cutoff freq: fl"=w3149, "sampling freq: fs"=w3151, "x"=w3152) -> ("Filtered x"=w3150:dbl)  [unwired: 3 in, 1 out]
                }
              }
              frame 100 {
                n460 = for {
                  tunnel: w3153 -> [w3166] mode=indexing
                  tunnel: w3158 -> [w3163]
                  tunnel: w3159 -> [w3165]
                  tunnel: [w3164] -> w3154 mode=indexing
                  tunnel: [w3163] -> w3157
                  tunnel: w3156 -> [w3161]
                  tunnel: w3155 -> [w3160]
                  n461 = call <vilib>:"Butterworth Filter PtByPt.vi"("initialize"=w3161, "order"=w3160, "filter type"=Filter_Passband_Type."Lowpass", "low cutoff freq: fl"=w3163, "sampling freq: fs"=w3165, "x"=w3166) -> ("Filtered x"=w3164:dbl)  [unwired: 3 in, 1 out]
                }
              }
              frame 101 {
                n462 = for {
                  tunnel: w3167 -> [w3180] mode=indexing
                  tunnel: w3172 -> [w3177]
                  tunnel: w3173 -> [w3179]
                  tunnel: [w3178] -> w3168 mode=indexing
                  tunnel: [w3177] -> w3171
                  tunnel: w3170 -> [w3175]
                  tunnel: w3169 -> [w3174]
                  n463 = call <vilib>:"Butterworth Filter PtByPt.vi"("initialize"=w3175, "order"=w3174, "filter type"=Filter_Passband_Type."Lowpass", "low cutoff freq: fl"=w3177, "sampling freq: fs"=w3179, "x"=w3180) -> ("Filtered x"=w3178:dbl)  [unwired: 3 in, 1 out]
                }
              }
              frame 102 {
                n464 = for {
                  tunnel: w3181 -> [w3194] mode=indexing
                  tunnel: w3186 -> [w3191]
                  tunnel: w3187 -> [w3193]
                  tunnel: [w3192] -> w3182 mode=indexing
                  tunnel: [w3191] -> w3185
                  tunnel: w3184 -> [w3189]
                  tunnel: w3183 -> [w3188]
                  n465 = call <vilib>:"Butterworth Filter PtByPt.vi"("initialize"=w3189, "order"=w3188, "filter type"=Filter_Passband_Type."Lowpass", "low cutoff freq: fl"=w3191, "sampling freq: fs"=w3193, "x"=w3194) -> ("Filtered x"=w3192:dbl)  [unwired: 3 in, 1 out]
                }
              }
              frame 103 {
                n466 = for {
                  tunnel: w3195 -> [w3208] mode=indexing
                  tunnel: w3200 -> [w3205]
                  tunnel: w3201 -> [w3207]
                  tunnel: [w3206] -> w3196 mode=indexing
                  tunnel: [w3205] -> w3199
                  tunnel: w3198 -> [w3203]
                  tunnel: w3197 -> [w3202]
                  n467 = call <vilib>:"Butterworth Filter PtByPt.vi"("initialize"=w3203, "order"=w3202, "filter type"=Filter_Passband_Type."Lowpass", "low cutoff freq: fl"=w3205, "sampling freq: fs"=w3207, "x"=w3208) -> ("Filtered x"=w3206:dbl)  [unwired: 3 in, 1 out]
                }
              }
              frame 104 {
                n468 = for {
                  tunnel: w3209 -> [w3222] mode=indexing
                  tunnel: w3214 -> [w3219]
                  tunnel: w3215 -> [w3221]
                  tunnel: [w3220] -> w3210 mode=indexing
                  tunnel: [w3219] -> w3213
                  tunnel: w3212 -> [w3217]
                  tunnel: w3211 -> [w3216]
                  n469 = call <vilib>:"Butterworth Filter PtByPt.vi"("initialize"=w3217, "order"=w3216, "filter type"=Filter_Passband_Type."Lowpass", "low cutoff freq: fl"=w3219, "sampling freq: fs"=w3221, "x"=w3222) -> ("Filtered x"=w3220:dbl)  [unwired: 3 in, 1 out]
                }
              }
              frame 105 {
                n470 = for {
                  tunnel: w3223 -> [w3236] mode=indexing
                  tunnel: w3228 -> [w3233]
                  tunnel: w3229 -> [w3235]
                  tunnel: [w3234] -> w3224 mode=indexing
                  tunnel: [w3233] -> w3227
                  tunnel: w3226 -> [w3231]
                  tunnel: w3225 -> [w3230]
                  n471 = call <vilib>:"Butterworth Filter PtByPt.vi"("initialize"=w3231, "order"=w3230, "filter type"=Filter_Passband_Type."Lowpass", "low cutoff freq: fl"=w3233, "sampling freq: fs"=w3235, "x"=w3236) -> ("Filtered x"=w3234:dbl)  [unwired: 3 in, 1 out]
                }
              }
              frame 106 {
                n472 = for {
                  tunnel: w3237 -> [w3250] mode=indexing
                  tunnel: w3242 -> [w3247]
                  tunnel: w3243 -> [w3249]
                  tunnel: [w3248] -> w3238 mode=indexing
                  tunnel: [w3247] -> w3241
                  tunnel: w3240 -> [w3245]
                  tunnel: w3239 -> [w3244]
                  n473 = call <vilib>:"Butterworth Filter PtByPt.vi"("initialize"=w3245, "order"=w3244, "filter type"=Filter_Passband_Type."Lowpass", "low cutoff freq: fl"=w3247, "sampling freq: fs"=w3249, "x"=w3250) -> ("Filtered x"=w3248:dbl)  [unwired: 3 in, 1 out]
                }
              }
              frame 107 {
                n474 = for {
                  tunnel: w3251 -> [w3264] mode=indexing
                  tunnel: w3256 -> [w3261]
                  tunnel: w3257 -> [w3263]
                  tunnel: [w3262] -> w3252 mode=indexing
                  tunnel: [w3261] -> w3255
                  tunnel: w3254 -> [w3259]
                  tunnel: w3253 -> [w3258]
                  n475 = call <vilib>:"Butterworth Filter PtByPt.vi"("initialize"=w3259, "order"=w3258, "filter type"=Filter_Passband_Type."Lowpass", "low cutoff freq: fl"=w3261, "sampling freq: fs"=w3263, "x"=w3264) -> ("Filtered x"=w3262:dbl)  [unwired: 3 in, 1 out]
                }
              }
              frame 108 {
                n476 = for {
                  tunnel: w3265 -> [w3278] mode=indexing
                  tunnel: w3270 -> [w3275]
                  tunnel: w3271 -> [w3277]
                  tunnel: [w3276] -> w3266 mode=indexing
                  tunnel: [w3275] -> w3269
                  tunnel: w3268 -> [w3273]
                  tunnel: w3267 -> [w3272]
                  n477 = call <vilib>:"Butterworth Filter PtByPt.vi"("initialize"=w3273, "order"=w3272, "filter type"=Filter_Passband_Type."Lowpass", "low cutoff freq: fl"=w3275, "sampling freq: fs"=w3277, "x"=w3278) -> ("Filtered x"=w3276:dbl)  [unwired: 3 in, 1 out]
                }
              }
              frame 109 {
                n478 = for {
                  tunnel: w3279 -> [w3292] mode=indexing
                  tunnel: w3284 -> [w3289]
                  tunnel: w3285 -> [w3291]
                  tunnel: [w3290] -> w3280 mode=indexing
                  tunnel: [w3289] -> w3283
                  tunnel: w3282 -> [w3287]
                  tunnel: w3281 -> [w3286]
                  n479 = call <vilib>:"Butterworth Filter PtByPt.vi"("initialize"=w3287, "order"=w3286, "filter type"=Filter_Passband_Type."Lowpass", "low cutoff freq: fl"=w3289, "sampling freq: fs"=w3291, "x"=w3292) -> ("Filtered x"=w3290:dbl)  [unwired: 3 in, 1 out]
                }
              }
              frame 110 {
                n480 = for {
                  tunnel: w3293 -> [w3306] mode=indexing
                  tunnel: w3298 -> [w3303]
                  tunnel: w3299 -> [w3305]
                  tunnel: [w3304] -> w3294 mode=indexing
                  tunnel: [w3303] -> w3297
                  tunnel: w3296 -> [w3301]
                  tunnel: w3295 -> [w3300]
                  n481 = call <vilib>:"Butterworth Filter PtByPt.vi"("initialize"=w3301, "order"=w3300, "filter type"=Filter_Passband_Type."Lowpass", "low cutoff freq: fl"=w3303, "sampling freq: fs"=w3305, "x"=w3306) -> ("Filtered x"=w3304:dbl)  [unwired: 3 in, 1 out]
                }
              }
              frame 111 {
                n482 = for {
                  tunnel: w3307 -> [w3320] mode=indexing
                  tunnel: w3312 -> [w3317]
                  tunnel: w3313 -> [w3319]
                  tunnel: [w3318] -> w3308 mode=indexing
                  tunnel: [w3317] -> w3311
                  tunnel: w3310 -> [w3315]
                  tunnel: w3309 -> [w3314]
                  n483 = call <vilib>:"Butterworth Filter PtByPt.vi"("initialize"=w3315, "order"=w3314, "filter type"=Filter_Passband_Type."Lowpass", "low cutoff freq: fl"=w3317, "sampling freq: fs"=w3319, "x"=w3320) -> ("Filtered x"=w3318:dbl)  [unwired: 3 in, 1 out]
                }
              }
              frame 112 {
                n484 = for {
                  tunnel: w3321 -> [w3334] mode=indexing
                  tunnel: w3326 -> [w3331]
                  tunnel: w3327 -> [w3333]
                  tunnel: [w3332] -> w3322 mode=indexing
                  tunnel: [w3331] -> w3325
                  tunnel: w3324 -> [w3329]
                  tunnel: w3323 -> [w3328]
                  n485 = call <vilib>:"Butterworth Filter PtByPt.vi"("initialize"=w3329, "order"=w3328, "filter type"=Filter_Passband_Type."Lowpass", "low cutoff freq: fl"=w3331, "sampling freq: fs"=w3333, "x"=w3334) -> ("Filtered x"=w3332:dbl)  [unwired: 3 in, 1 out]
                }
              }
              frame 113 {
                n486 = for {
                  tunnel: w3335 -> [w3348] mode=indexing
                  tunnel: w3340 -> [w3345]
                  tunnel: w3341 -> [w3347]
                  tunnel: [w3346] -> w3336 mode=indexing
                  tunnel: [w3345] -> w3339
                  tunnel: w3338 -> [w3343]
                  tunnel: w3337 -> [w3342]
                  n487 = call <vilib>:"Butterworth Filter PtByPt.vi"("initialize"=w3343, "order"=w3342, "filter type"=Filter_Passband_Type."Lowpass", "low cutoff freq: fl"=w3345, "sampling freq: fs"=w3347, "x"=w3348) -> ("Filtered x"=w3346:dbl)  [unwired: 3 in, 1 out]
                }
              }
              frame 114 {
                n488 = for {
                  tunnel: w3349 -> [w3362] mode=indexing
                  tunnel: w3354 -> [w3359]
                  tunnel: w3355 -> [w3361]
                  tunnel: [w3360] -> w3350 mode=indexing
                  tunnel: [w3359] -> w3353
                  tunnel: w3352 -> [w3357]
                  tunnel: w3351 -> [w3356]
                  n489 = call <vilib>:"Butterworth Filter PtByPt.vi"("initialize"=w3357, "order"=w3356, "filter type"=Filter_Passband_Type."Lowpass", "low cutoff freq: fl"=w3359, "sampling freq: fs"=w3361, "x"=w3362) -> ("Filtered x"=w3360:dbl)  [unwired: 3 in, 1 out]
                }
              }
              frame 115 {
                n490 = for {
                  tunnel: w3363 -> [w3376] mode=indexing
                  tunnel: w3368 -> [w3373]
                  tunnel: w3369 -> [w3375]
                  tunnel: [w3374] -> w3364 mode=indexing
                  tunnel: [w3373] -> w3367
                  tunnel: w3366 -> [w3371]
                  tunnel: w3365 -> [w3370]
                  n491 = call <vilib>:"Butterworth Filter PtByPt.vi"("initialize"=w3371, "order"=w3370, "filter type"=Filter_Passband_Type."Lowpass", "low cutoff freq: fl"=w3373, "sampling freq: fs"=w3375, "x"=w3376) -> ("Filtered x"=w3374:dbl)  [unwired: 3 in, 1 out]
                }
              }
              frame 116 {
                n492 = for {
                  tunnel: w3377 -> [w3390] mode=indexing
                  tunnel: w3382 -> [w3387]
                  tunnel: w3383 -> [w3389]
                  tunnel: [w3388] -> w3378 mode=indexing
                  tunnel: [w3387] -> w3381
                  tunnel: w3380 -> [w3385]
                  tunnel: w3379 -> [w3384]
                  n493 = call <vilib>:"Butterworth Filter PtByPt.vi"("initialize"=w3385, "order"=w3384, "filter type"=Filter_Passband_Type."Lowpass", "low cutoff freq: fl"=w3387, "sampling freq: fs"=w3389, "x"=w3390) -> ("Filtered x"=w3388:dbl)  [unwired: 3 in, 1 out]
                }
              }
              frame 117 {
                n494 = for {
                  tunnel: w3391 -> [w3404] mode=indexing
                  tunnel: w3396 -> [w3401]
                  tunnel: w3397 -> [w3403]
                  tunnel: [w3402] -> w3392 mode=indexing
                  tunnel: [w3401] -> w3395
                  tunnel: w3394 -> [w3399]
                  tunnel: w3393 -> [w3398]
                  n495 = call <vilib>:"Butterworth Filter PtByPt.vi"("initialize"=w3399, "order"=w3398, "filter type"=Filter_Passband_Type."Lowpass", "low cutoff freq: fl"=w3401, "sampling freq: fs"=w3403, "x"=w3404) -> ("Filtered x"=w3402:dbl)  [unwired: 3 in, 1 out]
                }
              }
              frame 118 {
                n496 = for {
                  tunnel: w3405 -> [w3418] mode=indexing
                  tunnel: w3410 -> [w3415]
                  tunnel: w3411 -> [w3417]
                  tunnel: [w3416] -> w3406 mode=indexing
                  tunnel: [w3415] -> w3409
                  tunnel: w3408 -> [w3413]
                  tunnel: w3407 -> [w3412]
                  n497 = call <vilib>:"Butterworth Filter PtByPt.vi"("initialize"=w3413, "order"=w3412, "filter type"=Filter_Passband_Type."Lowpass", "low cutoff freq: fl"=w3415, "sampling freq: fs"=w3417, "x"=w3418) -> ("Filtered x"=w3416:dbl)  [unwired: 3 in, 1 out]
                }
              }
              frame 119 {
                n498 = for {
                  tunnel: w3419 -> [w3432] mode=indexing
                  tunnel: w3424 -> [w3429]
                  tunnel: w3425 -> [w3431]
                  tunnel: [w3430] -> w3420 mode=indexing
                  tunnel: [w3429] -> w3423
                  tunnel: w3422 -> [w3427]
                  tunnel: w3421 -> [w3426]
                  n499 = call <vilib>:"Butterworth Filter PtByPt.vi"("initialize"=w3427, "order"=w3426, "filter type"=Filter_Passband_Type."Lowpass", "low cutoff freq: fl"=w3429, "sampling freq: fs"=w3431, "x"=w3432) -> ("Filtered x"=w3430:dbl)  [unwired: 3 in, 1 out]
                }
              }
              frame 120 {
                n500 = for {
                  tunnel: w3433 -> [w3446] mode=indexing
                  tunnel: w3438 -> [w3443]
                  tunnel: w3439 -> [w3445]
                  tunnel: [w3444] -> w3434 mode=indexing
                  tunnel: [w3443] -> w3437
                  tunnel: w3436 -> [w3441]
                  tunnel: w3435 -> [w3440]
                  n501 = call <vilib>:"Butterworth Filter PtByPt.vi"("initialize"=w3441, "order"=w3440, "filter type"=Filter_Passband_Type."Lowpass", "low cutoff freq: fl"=w3443, "sampling freq: fs"=w3445, "x"=w3446) -> ("Filtered x"=w3444:dbl)  [unwired: 3 in, 1 out]
                }
              }
              frame 121 {
                n502 = for {
                  tunnel: w3447 -> [w3460] mode=indexing
                  tunnel: w3452 -> [w3457]
                  tunnel: w3453 -> [w3459]
                  tunnel: [w3458] -> w3448 mode=indexing
                  tunnel: [w3457] -> w3451
                  tunnel: w3450 -> [w3455]
                  tunnel: w3449 -> [w3454]
                  n503 = call <vilib>:"Butterworth Filter PtByPt.vi"("initialize"=w3455, "order"=w3454, "filter type"=Filter_Passband_Type."Lowpass", "low cutoff freq: fl"=w3457, "sampling freq: fs"=w3459, "x"=w3460) -> ("Filtered x"=w3458:dbl)  [unwired: 3 in, 1 out]
                }
              }
              frame 122 {
                n504 = for {
                  tunnel: w3461 -> [w3474] mode=indexing
                  tunnel: w3466 -> [w3471]
                  tunnel: w3467 -> [w3473]
                  tunnel: [w3472] -> w3462 mode=indexing
                  tunnel: [w3471] -> w3465
                  tunnel: w3464 -> [w3469]
                  tunnel: w3463 -> [w3468]
                  n505 = call <vilib>:"Butterworth Filter PtByPt.vi"("initialize"=w3469, "order"=w3468, "filter type"=Filter_Passband_Type."Lowpass", "low cutoff freq: fl"=w3471, "sampling freq: fs"=w3473, "x"=w3474) -> ("Filtered x"=w3472:dbl)  [unwired: 3 in, 1 out]
                }
              }
              frame 123 {
                n506 = for {
                  tunnel: w3475 -> [w3488] mode=indexing
                  tunnel: w3480 -> [w3485]
                  tunnel: w3481 -> [w3487]
                  tunnel: [w3486] -> w3476 mode=indexing
                  tunnel: [w3485] -> w3479
                  tunnel: w3478 -> [w3483]
                  tunnel: w3477 -> [w3482]
                  n507 = call <vilib>:"Butterworth Filter PtByPt.vi"("initialize"=w3483, "order"=w3482, "filter type"=Filter_Passband_Type."Lowpass", "low cutoff freq: fl"=w3485, "sampling freq: fs"=w3487, "x"=w3488) -> ("Filtered x"=w3486:dbl)  [unwired: 3 in, 1 out]
                }
              }
            }
            n508 = Bundle By Name(cluster=w1800, "Y"=w1803) -> (w1799:waveform(dbl))
            n509 = in-place-array #2(w1799) -> (w1791:waveform(dbl)[])  [unwired: 1 out]
          }
        }
      }
    }
    frame "method 3" {
      # "For loop access each channel"
      # "While loop is used to store the previous low cutoff frequency fl. If fl changes reset the filter history."
      # "Each case is for a different lockin channel. The Butterworth Filter Pt by Pt in each case has its own history (Preallocated clone reentrant execution)."
      # "method 2: how to not use case structure? How to not use Pt by Pt filter?"
      n510 = while {
        tunnel: w3493 -> [w3496]
        tunnel: [w3502] -> w3492
        tunnel: w3491 -> [w3500]
        tunnel: w3490 -> [w3498]
        shift-right: [w3495] -> _
        shift-left: _ -> [w3494]
        tunnel: w3489 -> [w3499]
        stop <- TRUE stop-if-true
        n511 = Not Equal?(x=w3494, y=w3498) -> (x != y?=w3497:bool)
        n512 = for {
          tunnel: w3500 -> [_]
          tunnel: w3498 -> [w3503]
          tunnel: w3497 -> [_]
          tunnel: w3499 -> [w3504]
          tunnel: [w3503] -> w3495
          tunnel: w3496 -> [w3506] mode=indexing
          tunnel: [w3505] -> w3502 mode=indexing
          n513 = call-poly <vilib>:"SI Lowpass Filter.vi"("cutoff frequency"=w3503, "order"=w3504, "stimulus signal in"=w3506) -> ("stimulus signal out"=w3505:waveform(dbl))  [unwired: 6 in, 2 out]
        }
      }
    }
    frame "method 4" {
      # "For loop access each channel"
      # "While loop is used to store the previous low cutoff frequency fl. If fl changes reset the filter history."
      # "Each case is for a different lockin channel. The Butterworth Filter Pt by Pt in each case has its own history (Preallocated clone reentrant execution)."
      # "method 4: how to not use case structure? How to not use Pt by Pt filter?"
      n514 = while {
        tunnel: w3511 -> [w3514]
        tunnel: [w3520] -> w3510
        tunnel: w3509 -> [w3518]
        tunnel: w3508 -> [w3516]
        shift-right: [w3513] -> _
        shift-left: _ -> [w3512]
        tunnel: w3507 -> [w3517]
        stop <- TRUE stop-if-true
        n515 = Not Equal?(x=w3512, y=w3516) -> (x != y?=w3515:bool)
        n516 = for {
          tunnel: w3518 -> [_]
          tunnel: w3516 -> [w3527]
          tunnel: w3515 -> [_]
          tunnel: w3517 -> [_]
          tunnel: [w3527] -> w3513
          tunnel: w3514 -> [w3526] mode=indexing
          tunnel: [w3525] -> w3520 mode=indexing
          n517 = Unbundle By Name(w3526) -> ("Y"=w3523:dbl[])
          n518 = Array Size(array=w3523) -> ()  [unwired: 1 out]
          n519 = call-poly <vilib>:"Mean.vi"("X"=w3523) -> ("mean"=w3524:dbl)  [unwired: 1 out]
          n520 = Initialize Array(w3524, 1 ("dimension size")) -> (w3522:dbl[])
          n521 = Bundle By Name(cluster=w3526, "Y"=w3522) -> (w3525:waveform(dbl))
        }
      }
    }
    frame "method 5" {
      # "method 5: Digital Filter Toolkit has built-in method to filter Array of Waveforms!"
      n522 = while {
        tunnel: w3532 -> [w3541]
        tunnel: [w3540] -> w3531
        tunnel: w3530 -> [w3533]
        tunnel: w3529 -> [w3534]
        shift-right: [w3534] -> _
        shift-left: _ -> [w3542]
        tunnel: w3528 -> [w3535]
        stop <- TRUE stop-if-true
        n523 = Not Equal?(x=w3542, y=w3534) -> (x != y?=w3539:bool)
        n524 = call <vilib>:"DFD Butterworth Design.vi"("fs [Hz]"=w3533, "filter type"=T3."Lowpass", "low cutoff freq [Hz]"=w3534, "order"=w3535) -> ("error out"=w3536:errorcluster, "filter out"=w3537:T4)  [unwired: 6 in]
        n525 = call-poly <vilib>:"DFD Filtering.vi"("init? (F)"=w3539, "error in (no error)"=w3536, "filter"=w3537, "signal in"=w3541) -> ("signal out"=w3540:waveform(dbl)[])  [unwired: 6 in, 1 out]
      }
    }
  }
  "Array out" <- w4
